vi "CRYO_MASTER_FULL_RUN4.vi"() -> ()   [LabVIEW 2017]
uses:
  LSI218Data.lvclass
  LSI336Data.lvclass
  USBData.lvclass
  6240AData.lvclass
  DMMsData.lvclass
  LMData.lvclass
  <vilib>/DAQmx/miscellaneous.llb/DAQmx Fill In Error Info.vi
  <vilib>/DAQmx/create/channels.llb/DAQmx Create Channel (DO-Digital Output).vi
  <vilib>/DAQmx/create/channels.llb/DAQmx Create Channel (AO-Voltage-Basic).vi
  <vilib>/express/express arith-compare/Formula/XNode/ExpressFormulaBlockNode.xnode
  <vilib>/Analysis/NI_AALBase.lvlib
  istr.lib/Agilent 33XXX Series/Agilent 33XXX Series.lvlib
panel:
  out "Heat Cycle counter":i32
  in  "V_peak":dbl=65.0 format="%_4f"
  in  "Automatic \nScreenshots?":bool=TRUE
  in  "Frontpanel screenshots":bool
  in  "Screenshots interval":i64=3605
  in  "Record interval":i64=20
  out "Cycle #":u32=1
  in  "Measurement Interval (s)":dbl=1.0
  in  "Stop Button":bool
  in  "?":T1(tab)=enum."CHF"
  out "RUN Identifier":string="20210209_084357_RUNIII"
  in  "Base Path (screenshots)":path=path "C:/LabVIEW/DATA/Google/TUCAN Experiments/KEK_cryotests_2019-2020/data/screenshots"
  out "error out (USB6210/6218 AOUT)":errorcluster
  in  "AOUT Labels":string[](array[string])=["PWR400H_I", "PMC183A_I"]
  in  "DOUT Labels":string[](array[string])=["D_V1_NO", "D_V2_NC", "D_CV1", "D_H1"]
  in  "AOUT assignment":tag[](array[tag])=["Dev1/ao0", "Dev1/ao1"]
  out "AO task out":refnum<k21>="20210209_084357_RUNIII_AO"
  in  "Analog Out ON?":bool=TRUE
  in  "InstName (USB6218)":string="USB6218"
  in  "USB6218 Config":T2(array[cluster])=[{"Label"="F_1", "FileFormat"="%5.5f", "Active?"=TRUE, "Physical CH"="Dev1/ai0", " terminal\n type"=10083, "ConversionType"={"Type"=enum."SimpleProp", "ConversionParameters"=[0.0, 5.0, 0.0, 500.0]}, "VoltageLimits"=[0.0, 5.0]}, {"Label"="F_2", "FileFormat"="%5.5f", "Active?"=TRUE, "Physical CH"="Dev1/ai1", " terminal\n type"=10083, "ConversionType"={"Type"=enum."SimpleProp", "ConversionParameters"=[0.0, 5.0, 0.0, 200.0]}, "VoltageLimits"=[0.0, 5.0]}, {"Label"="F_3", "FileFormat"="%5.5f", "Active?"=TRUE, "Physical CH"="Dev1/ai2", " terminal\n type"=10083, "ConversionType"={"Type"=enum."SimpleProp", "ConversionParameters"=[0.0, 5.0, 0.0, 200.0]}, "VoltageLimits"=[0.0, 5.0]}, {"Label"="F_4", "FileFormat"="%5.5f", "Active?"=TRUE, "Physical CH"="Dev1/ai3", " terminal\n type"=10083, "ConversionType"={"Type"=enum."SimpleProp", "ConversionParameters"=[0.0, 5.0, 0.0, 500.0]}, "VoltageLimits"=[0.0, 5.0]}, {"Label"="F_5", "FileFormat"="%5.5f", "Active?"=TRUE, "Physical CH"="Dev1/ai4", " terminal\n type"=10083, "ConversionType"={"Type"=enum."SimpleProp", "ConversionParameters"=[0.0, 5.0, 0.0, 500.0]}, "VoltageLimits"=[0.0, 5.0]}, {"Label"="I_CV", "FileFormat"="%3.5f", "Active?"=TRUE, "Physical CH"="Dev1/ai5", " terminal\n type"=10083, "ConversionType"={"Type"=enum."Raw", "ConversionParameters"=[0.0, 0.0, 0.0, 0.0]}, "VoltageLimits"=[0.0, 10.0]}, {"Label"="CV1_answer", "FileFormat"="%3.5f", "Active?"=TRUE, "Physical CH"="Dev1/ai6", " terminal\n type"=10083, "ConversionType"={"Type"=enum."SimpleProp", "ConversionParameters"=[1.0, 5.0, 0.0, 100.0]}, "VoltageLimits"=[0.0, 5.0]}, {"Label"="P_Dewar", "FileFormat"="%5.5e", "Active?"=TRUE, "Physical CH"="Dev1/ai7", " terminal\n type"=10083, "ConversionType"={"Type"=enum."SimpleProp", "ConversionParameters"=[1.0, 5.0, 0.0, 200000.0]}, "VoltageLimits"=[0.0, 5.0]}, {"Label"="L_Dewar", "FileFormat"="%5.5f", "Active?"=TRUE, "Physical CH"="Dev1/ai8", " terminal\n type"=10083, "ConversionType"={"Type"=enum."SimpleProp", "ConversionParameters"=[0.0, 10.0, 0.0, 100.0]}, "VoltageLimits"=[0.0, 10.0]}] {"terminal\n type" items=["Default"=-1, "RSE"=10083, "NRSE"=10078, "Differential"=10106, "Pseudodifferential"=12529]}
  out "error out (USB6218)":errorcluster
  out "error out (USB6210/6218 DOUT)":errorcluster
  out "DOUT task out":refnum<k21>="20210209_084357_DO"
  in  "DOUT Physical CH":tag[](array[tag])=["Dev1/port1/line0", "Dev1/port1/line1", "Dev1/port1/line2", "Dev1/port1/line3"]
  in  "Digital Out ON?":bool=TRUE
  in  "USB6210 Config":T2(array[cluster])=[{"Label"="P_ins", "FileFormat"="%5.5e", "Active?"=TRUE, "Physical CH"="Dev2/ai0", " terminal\n type"=10083, "ConversionType"={"Type"=enum."CC-10_LOG", "ConversionParameters"=[0.5, 9.0, 0.0, 1.0]}, "VoltageLimits"=[0.0, 10.0]}, {"Label"="P_4Kres", "FileFormat"="%5.5e", "Active?"=TRUE, "Physical CH"="Dev2/ai1", " terminal\n type"=10083, "ConversionType"={"Type"=enum."SimpleProp", "ConversionParameters"=[1.0, 5.0, 0.0, 200000.0]}, "VoltageLimits"=[0.0, 5.0]}, {"Label"="P_3HeIN", "FileFormat"="%5.5e", "Active?"=TRUE, "Physical CH"="Dev2/ai2", " terminal\n type"=10083, "ConversionType"={"Type"=enum."SimpleProp", "ConversionParameters"=[1.0, 5.0, 0.0, 200000.0]}, "VoltageLimits"=[0.0, 5.0]}, {"Label"="P_SldRTN", "FileFormat"="%5.5e", "Active?"=TRUE, "Physical CH"="Dev2/ai3", " terminal\n type"=10083, "ConversionType"={"Type"=enum."SimpleProp", "ConversionParameters"=[1.0, 5.0, 0.0, 200000.0]}, "VoltageLimits"=[0.0, 5.0]}, {"Label"="P_3Hepot", "FileFormat"="%5.5e", "Active?"=TRUE, "Physical CH"="Dev2/ai4", " terminal\n type"=10083, "ConversionType"={"Type"=enum."SimpleProp", "ConversionParameters"=[0.0, 10.0, 0.0, 133320.0]}, "VoltageLimits"=[0.0, 10.0]}, {"Label"="P_1Kpot", "FileFormat"="%5.5e", "Active?"=TRUE, "Physical CH"="Dev2/ai5", " terminal\n type"=10083, "ConversionType"={"Type"=enum."SimpleProp", "ConversionParameters"=[0.0, 10.0, 0.0, 133320.0]}, "VoltageLimits"=[0.0, 10.0]}, {"Label"="P_Dewar(old)", "FileFormat"="%5.5e", "Active?"=FALSE, "Physical CH"="Dev2/ai6", " terminal\n type"=10083, "ConversionType"={"Type"=enum."SimpleProp", "ConversionParameters"=[1.0, 5.0, 0.0, 200000.0]}, "VoltageLimits"=[0.0, 5.0]}, {"Label"="DP_HEX4", "FileFormat"="%5.5e", "Active?"=TRUE, "Physical CH"="Dev2/ai7", " terminal\n type"=10083, "ConversionType"={"Type"=enum."SimpleProp", "ConversionParameters"=[1.0, 5.0, 0.0, 1000.0]}, "VoltageLimits"=[0.0, 5.0]}, {"Label"="DP_HEX5", "FileFormat"="%5.5e", "Active?"=TRUE, "Physical CH"="Dev2/ai8", " terminal\n type"=10083, "ConversionType"={"Type"=enum."SimpleProp", "ConversionParameters"=[1.0, 5.0, 0.0, 1000.0]}, "VoltageLimits"=[0.0, 5.0]}, {"Label"="L1(old)", "FileFormat"="%5.5f", "Active?"=TRUE, "Physical CH"="Dev2/ai9", " terminal\n type"=10083, "ConversionType"={"Type"=enum."SimpleProp", "ConversionParameters"=[0.0, 10.0, 0.0, 100.0]}, "VoltageLimits"=[0.0, 10.0]}, {"Label"="L2-1", "FileFormat"="%5.5f", "Active?"=TRUE, "Physical CH"="Dev2/ai10", " terminal\n type"=10083, "ConversionType"={"Type"=enum."SimpleProp", "ConversionParameters"=[0.0, 10.0, 0.0, 100.0]}, "VoltageLimits"=[0.0, 10.0]}, {"Label"="L2-2", "FileFormat"="%5.5f", "Active?"=TRUE, "Physical CH"="Dev2/ai11", " terminal\n type"=10083, "ConversionType"={"Type"=enum."SimpleProp", "ConversionParameters"=[0.0, 10.0, 0.0, 100.0]}, "VoltageLimits"=[0.0, 10.0]}, {"Label"="L3", "FileFormat"="%5.5f", "Active?"=TRUE, "Physical CH"="Dev2/ai12", " terminal\n type"=10083, "ConversionType"={"Type"=enum."SimpleProp", "ConversionParameters"=[0.0, 10.0, 0.0, 100.0]}, "VoltageLimits"=[0.0, 10.0]}, {"Label"="P_HEX7OUT", "FileFormat"="%5.5e", "Active?"=TRUE, "Physical CH"="Dev2/ai13", " terminal\n type"=10083, "ConversionType"={"Type"=enum."SimpleProp", "ConversionParameters"=[1.0, 5.0, 0.0, 200000.0]}, "VoltageLimits"=[0.0, 5.0]}, {"Label"="P_IP", "FileFormat"="%5.5e", "Active?"=TRUE, "Physical CH"="Dev2/ai14", " terminal\n type"=10083, "ConversionType"={"Type"=enum."CC-10_LOG", "ConversionParameters"=[0.5, 9.0, 0.0, 1.0]}, "VoltageLimits"=[0.0, 10.0]}, {"Label"="V_H1", "FileFormat"="%3.5f", "Active?"=TRUE, "Physical CH"="Dev2/ai15", " terminal\n type"=10083, "ConversionType"={"Type"=enum."Raw", "ConversionParameters"=[0.0, 1.0, 0.0, 1.0]}, "VoltageLimits"=[0.0, 10.0]}] {"terminal\n type" items=["Default"=-1, "RSE"=10083, "NRSE"=10078, "Differential"=10106, "Pseudodifferential"=12529]}
  in  "RUN label":string="RUNIII"
  in  "Base Path":path=path "C:/LabVIEW/DATA/RUN_3"
  in  "InstName (USB6210)":string="USB6210"
  out "error out (USB6210)":errorcluster
  out "File Refn USB AO":refnum<file>
  out "File Refn USB DO":refnum<file>
  in  "LM measurement interval (>0)":i64=1
  in  "Active? (HP34401 LM)":bool=TRUE
  in  "Labels (HP34401 LM)":string[](array[string])=["R_L1", "L1"]
  in  "FileFormat (HP34401 LM)":string[](array[string])=["%.4f", "%.4f"]
  in  "VISA (HP34401 LM)":refnum<visa-resource-name>="GPIB0::24::INSTR"
  in  "LevelCalibration (R0, R1, L0, L1)":dbl[](array[numeric])=[179.74, 0.0, 0.0, 100.0]
  in  "InstName (HP34401 LM)":string="HP34401LM"
  out "error out (LSI336)":errorcluster
  in  "InstName (LSI336)":string="LSI336"
  in  "FileFormat (336)":string="%4.4f"
  in  "LSI336Settings(X,Y)":T3(array[cluster])=[{"LSIName"="LSi336X", "Labels"=["T1K3-1", "T1K3-2", "T3He5", "T3He8"], "SensorLocations"=[enum."T1K3-1", enum."T1K3-2", enum."T3He5", enum."T3He8"], "Active?"=TRUE, "VISA res. name"="COM15_LSI336Y"}, {"LSIName"="LSi336Y", "Labels"=["T3He6-1", "T3He6-2", "T3He7-1", "T3He7-2"], "SensorLocations"=[enum."T3He6-1", enum."T3He6-2", enum."T3He7-1", enum."T3He7-2"], "Active?"=TRUE, "VISA res. name"="COM20_LSI336X"}]
  in  "FileFormat (218)":string="%4.4f"
  in  "InstName (LSI218)":string="LSI218"
  in  "LSI218Settings(A-F)":T3(array[cluster])=[{"LSIName"="LSI218A", "Labels"=["T3He10", "T3He1-1", "TTH3", "TTH4", "TTH1", "TTH2", "T4He1", "T1K1"], "SensorLocations"=[enum."T3He10", enum."T3He1-1", enum."TTH3", enum."TTH4", enum."TTH1", enum."TTH2", enum."T4He1", enum."T1K1"], "Active?"=TRUE, "VISA res. name"="GPIB0::7::INSTR"}, {"LSIName"="LSI218B", "Labels"=["N.C.", "N.C.", "N.C.", "N.C.", "T3He2-1", "T3He2-2", "T3He3", "T3He1-4"], "SensorLocations"=[enum."N.C.", enum."N.C.", enum."N.C.", enum."N.C.", enum."T3He2-1", enum."T3He2-2", enum."T3He3", enum."T3He1-4"], "Active?"=TRUE, "VISA res. name"="GPIB0::4::INSTR"}, {"LSIName"="LSI218C", "Labels"=["T4He3-1", "T4He3-2", "T4He3-3", "T4He3-4", "T4He2-1", "T4He2-2", "T4He4", "T4He5"], "SensorLocations"=[enum."T4He3-1", enum."T4He3-2", enum."T4He3-3", enum."T4He3-4", enum."T4He2-1", enum."T4He2-2", enum."T4He4", enum."T4He5"], "Active?"=TRUE, "VISA res. name"="GPIB0::3::INSTR"}, {"LSIName"="LSI218D", "Labels"=["T4He6", "T4He9", "T3He1-2", "T3He1-3", "T4He7", "T4He8", "T4He10", "T1K6"], "SensorLocations"=[enum."T4He6", enum."T4He9", enum."T3He1-2", enum."T3He1-3", enum."T4He7", enum."T4He8", enum."T4He10", enum."T1K6"], "Active?"=TRUE, "VISA res. name"="GPIB0::5::INSTR"}, {"LSIName"="LSI218E", "Labels"=["TIP1", "N.C.", "TIP2", "N.C.", "TIP3", "TIP4", "TIP5", "N.C."], "SensorLocations"=[enum."TIP1", enum."N.C.", enum."TIP2", enum."N.C.", enum."TIP3", enum."TIP4", enum."TIP5", enum."N.C."], "Active?"=TRUE, "VISA res. name"="GPIB0::11::INSTR"}, {"LSIName"="LSI218F", "Labels"=["T1K2", "T1K4", "T1K5", "T3He4", "T3He9", "TIP6", "N.C.", "N.C."], "SensorLocations"=[enum."T1K2", enum."T1K4", enum."T1K5", enum."T3He4", enum."T3He9", enum."TIP6", enum."N.C.", enum."N.C."], "Active?"=TRUE, "VISA res. name"="GPIB0::8::INSTR"}]
  out "error out (LSI218)":errorcluster={"status"=TRUE, "code"=-1073807338, "source"="VISA Close in Lake Shore Cryotronics 218.lvlib:Close.vi->LSI218Data.lvclass:LSI218Data_terminate.vi->CRYO_MASTER_FULL_RUN3.vi"}
  out "RUN Identifier 2":string="20210209_084357_RUNIII" caption="RUN Identifier"
  out "error out (HP34401 LM)":errorcluster
  out "Graph 3":T4(graph)=[{"TimeArray"=[timestamp(3695672639.4136896 s since 1904-01-01)], "DataArray"=[-0.36185606613019977]}, {"TimeArray"=[timestamp(3695672639.4136896 s since 1904-01-01)], "DataArray"=[-1.4204433335631088]}, {"TimeArray"=[timestamp(3695672639.4136896 s since 1904-01-01)], "DataArray"=[0.28794373208354185]}, {"TimeArray"=[timestamp(3695672639.4136896 s since 1904-01-01)], "DataArray"=[-3.0973798990583647]}, {"TimeArray"=[timestamp(3695672639.4136896 s since 1904-01-01)], "DataArray"=[18.382396544680894]}, {"TimeArray"=[timestamp(3695672639.4136896 s since 1904-01-01)], "DataArray"=[-0.0024966396874153696]}, {"TimeArray"=[timestamp(3695672639.4136896 s since 1904-01-01)], "DataArray"=[107.20664477077275]}] caption="XY Graph"
  out "Graph 1":T4(graph)=[{"TimeArray"=[timestamp(3695672639.4087214 s since 1904-01-01)], "DataArray"=[18.674861858538797]}, {"TimeArray"=[timestamp(3695672639.4087214 s since 1904-01-01)], "DataArray"=[97865.81349287118]}, {"TimeArray"=[timestamp(3695672639.4087214 s since 1904-01-01)], "DataArray"=[100998.44453584745]}, {"TimeArray"=[timestamp(3695672639.4087214 s since 1904-01-01)], "DataArray"=[100709.02551899779]}, {"TimeArray"=[timestamp(3695672639.4087214 s since 1904-01-01)], "DataArray"=[101407.09548804205]}, {"TimeArray"=[timestamp(3695672639.4087214 s since 1904-01-01)], "DataArray"=[101279.08758660906]}, {"TimeArray"=[timestamp(3695672639.4087214 s since 1904-01-01)], "DataArray"=[0.0]}, {"TimeArray"=[timestamp(3695672639.4087214 s since 1904-01-01)], "DataArray"=[100273.25274306418]}, {"TimeArray"=[timestamp(3695672639.4087214 s since 1904-01-01)], "DataArray"=[4.684755546764993e-05]}, {"TimeArray"=[timestamp(3695672639.4136896 s since 1904-01-01)], "DataArray"=[102243.79868545999]}] caption="XY Graph"
  in  "FIle suffix 4":string="Graph4_noise"
  in  "Take Screenshot! 4":bool
  in  "Take Screenshot! 3":bool
  in  "Take Screenshot! 2":bool
  in  "Take Screenshot! 1":bool
  in  "FIle suffix 3":string="Graph3_noise"
  in  "FIle suffix 2":string="Graph2_noise"
  in  "FIle suffix 1":string="Graph1_noise"
  in  "log/linear 2":bool
  in  "Tab Control 2":T5(tab)
  in  "Plot selecter (USB6210)\n    1      2     3     4":bool[][](array[boolean])=[[TRUE, FALSE, FALSE, FALSE], [TRUE, FALSE, FALSE, FALSE], [TRUE, FALSE, FALSE, FALSE], [TRUE, FALSE, FALSE, FALSE], [TRUE, FALSE, FALSE, FALSE], [TRUE, FALSE, FALSE, FALSE], [TRUE, FALSE, FALSE, FALSE], [FALSE, TRUE, FALSE, FALSE], [FALSE, TRUE, FALSE, FALSE], [FALSE, TRUE, FALSE, FALSE], [FALSE, TRUE, FALSE, FALSE], [FALSE, TRUE, FALSE, FALSE], [FALSE, TRUE, FALSE, FALSE], [TRUE, FALSE, FALSE, FALSE], [TRUE, FALSE, FALSE, FALSE], [FALSE, FALSE, FALSE, FALSE]]
  out "All Labels (USB6210)":string[](array[string])=["P_ins", "P_4Kres", "P_3HeIN", "P_SldRTN", "P_3Hepot", "P_1Kpot", "P_Dewar(old)", "DP_HEX4", "DP_HEX5", "L1(old)", "L2-1", "L2-2", "L3", "P_HEX7OUT", "P_IP", "V_H1"]
  out "Last Data \n(USB6210)":dbl[](array[numeric])=[18.674861858538797, 97865.81349287118, 100998.44453584745, 100709.02551899779, 101407.09548804205, 101279.08758660906, 0.0, -48.20456535494683, 0.06691412080322978, 10.108489682314854, 0.1698011167381339, -0.07483544992953703, 0.04024895650740204, 100273.25274306418, 4.684755546764993e-05, 5.953981760223165] format="%#_6e"
  out "Time of Last Measurement (USB6210)":timestamp=timestamp(3695672639.4087214 s since 1904-01-01)
  out "USB6210 Status":T6(ring)=enum."Ready"
  out "Last Vol\n(USB6210)":dbl[](array[numeric])=[8.135628698970727, 2.9573162698574236, 3.019968890716949, 3.0141805103799557, 7.606292790882241, 7.596691238119492, 0.0, 0.8071817385802127, 1.000267656483213, 1.0108489682314854, 0.01698011167381339, -0.007483544992953703, 0.004024895650740204, 3.0054650548612836, 5.335343467039768, 5.953981760223165] format="%_5f"
  out "Labels (HP34401 LM) 2":string[](array[string])=["R_L1", "L1"]
  out "LastData (HP34401 LM)":dbl[](array[numeric])=[166.68232, 7.2647602091910555]
  in  "Plot selecter (HP34401A)\n    1      2     3     4":bool[][](array[boolean])=[[FALSE, TRUE, FALSE, FALSE], [FALSE, TRUE, FALSE, FALSE], [TRUE, FALSE, FALSE, FALSE], [TRUE, FALSE, FALSE, FALSE], [TRUE, FALSE, FALSE, FALSE], [TRUE, FALSE, FALSE, FALSE], [TRUE, FALSE, FALSE, FALSE], [FALSE, TRUE, FALSE, FALSE], [FALSE, TRUE, FALSE, FALSE], [FALSE, TRUE, FALSE, FALSE], [FALSE, TRUE, FALSE, FALSE], [FALSE, TRUE, FALSE, FALSE], [FALSE, TRUE, FALSE, FALSE], [TRUE, FALSE, FALSE, FALSE], [TRUE, FALSE, FALSE, FALSE], [FALSE, FALSE, FALSE, FALSE]]
  out "Time of Last Measurement (USB6218)":timestamp=timestamp(3695672639.4136896 s since 1904-01-01)
  out "USB6218 Status":T6(ring)=enum."Ready"
  out "Last Vol \n(USB6218)":dbl[](array[numeric])=[-0.003618560661301998, -0.03551108333907772, 0.0071985933020885465, -0.030973798990583647, 0.18382396544680896, -0.0024966396874153696, -0.0029609827608362395, 3.0448759737091997, 10.720664477077275] format="%_5f"
  out "Last Data \n(USB6218)":dbl[](array[numeric])=[-0.36185606613019977, -1.4204433335631088, 0.28794373208354185, -3.0973798990583647, 18.382396544680894, -0.0024966396874153696, -25.07402456902091, 102243.79868545999, 107.20664477077275] format="%#_6e"
  out "All Labels (USB6218)":string[](array[string])=["F_1", "F_2", "F_3", "F_4", "F_5", "I_CV", "CV1_answer", "P_Dewar", "L_Dewar"]
  in  "Plot selecter (USB6218)\n    1      2     3     4":bool[][](array[boolean])=[[FALSE, FALSE, TRUE, FALSE], [FALSE, FALSE, TRUE, FALSE], [FALSE, FALSE, TRUE, FALSE], [FALSE, FALSE, TRUE, FALSE], [FALSE, FALSE, TRUE, FALSE], [FALSE, FALSE, TRUE, FALSE], [FALSE, FALSE, FALSE, FALSE], [TRUE, FALSE, FALSE, FALSE], [FALSE, FALSE, TRUE, FALSE], [FALSE, FALSE, FALSE, TRUE], [FALSE, FALSE, FALSE, TRUE], [FALSE, FALSE, FALSE, TRUE], [FALSE, FALSE, FALSE, TRUE], [FALSE, FALSE, FALSE, FALSE], [FALSE, FALSE, FALSE, FALSE], [FALSE, FALSE, FALSE, FALSE]]
  out "Time of Last Measurement (LSI218)":timestamp=timestamp(3695672639.4087214 s since 1904-01-01)
  out "LSI218 Status":T7(ring)=enum."Measuring"
  out "Last Data \nLSI218 (1)":dbl[](array[numeric])=[286.39, 292.79, 245.71, 242.82, 192.73, 208.05, 129.14, 157.86, 30.0, 0.0, 0.0, 0.0, 214.32, 209.26, 161.19, 290.41, 293.53, 293.65, 291.53, 291.58, 216.58, 205.59, 215.41, 218.49]
  out "Labels LSI218 (1)":string[](array[string])=["T3He10", "T3He1-1", "TTH3", "TTH4", "TTH1", "TTH2", "T4He1", "T1K1", "N.C.", "N.C.", "N.C.", "N.C.", "T3He2-1", "T3He2-2", "T3He3", "T3He1-4", "T4He3-1", "T4He3-2", "T4He3-3", "T4He3-4", "T4He2-1", "T4He2-2", "T4He4", "T4He5"]
  in  "Plot selecter LSI218(1)\n    1      2     3     4":bool[][](array[boolean])=[[FALSE, FALSE, FALSE, FALSE], [FALSE, FALSE, FALSE, FALSE], [FALSE, FALSE, FALSE, TRUE], [FALSE, FALSE, FALSE, TRUE], [FALSE, FALSE, FALSE, TRUE], [FALSE, FALSE, FALSE, TRUE], [FALSE, FALSE, FALSE, TRUE], [FALSE, FALSE, FALSE, TRUE], [FALSE, FALSE, FALSE, FALSE], [FALSE, FALSE, FALSE, FALSE], [FALSE, FALSE, FALSE, FALSE], [FALSE, FALSE, FALSE, FALSE], [FALSE, FALSE, FALSE, TRUE], [FALSE, FALSE, FALSE, TRUE], [FALSE, FALSE, FALSE, FALSE], [FALSE, FALSE, FALSE, FALSE], [FALSE, FALSE, FALSE, TRUE], [FALSE, FALSE, FALSE, TRUE], [FALSE, FALSE, FALSE, TRUE], [FALSE, FALSE, FALSE, TRUE], [FALSE, FALSE, FALSE, TRUE], [FALSE, FALSE, FALSE, TRUE], [FALSE, FALSE, FALSE, TRUE], [FALSE, FALSE, FALSE, FALSE]]
  out "Active?\n (1)":bool[](array[boolean])=[TRUE, TRUE, TRUE, TRUE, TRUE, TRUE, TRUE, TRUE, TRUE, TRUE, TRUE, TRUE, TRUE, TRUE, TRUE, TRUE, TRUE, TRUE, TRUE, TRUE, TRUE, TRUE, TRUE, TRUE]
  out "Labels LSI218 (2)":string[](array[string])=["T4He6", "T4He9", "T3He1-2", "T3He1-3", "T4He7", "T4He8", "T4He10", "T1K6", "TIP1", "N.C.", "TIP2", "N.C.", "TIP3", "TIP4", "TIP5", "N.C.", "T1K2", "T1K4", "T1K5", "T3He4", "T3He9", "TIP6", "N.C.", "N.C."]
  out "Active?\n(2)":bool[](array[boolean])=[TRUE, TRUE, TRUE, TRUE, TRUE, TRUE, TRUE, TRUE, TRUE, TRUE, TRUE, TRUE, TRUE, TRUE, TRUE, TRUE, TRUE, TRUE, TRUE, TRUE, TRUE, TRUE, TRUE, TRUE]
  out "Last Data \nLSI218 (2)":dbl[](array[numeric])=[214.17, 227.11, 292.96, 290.69, 256.79, 281.72, 274.72, 287.38, 279.49, 0.0, 232.53, 688.49, 216.83, 149.55, 173.98, 688.58, 178.46, 128.79, 144.74, 152.95, 140.88, 150.1, 0.433, 0.0]
  in  "Plot selecter LSI218(2)\n    1      2     3     4":bool[][](array[boolean])=[[FALSE, FALSE, FALSE, FALSE], [FALSE, FALSE, FALSE, FALSE], [FALSE, FALSE, FALSE, FALSE], [FALSE, FALSE, FALSE, FALSE], [FALSE, FALSE, FALSE, FALSE], [FALSE, FALSE, FALSE, FALSE], [FALSE, FALSE, FALSE, FALSE], [FALSE, FALSE, FALSE, FALSE], [FALSE, FALSE, FALSE, FALSE], [FALSE, FALSE, FALSE, FALSE], [FALSE, FALSE, FALSE, FALSE], [FALSE, FALSE, FALSE, FALSE], [FALSE, FALSE, FALSE, FALSE], [FALSE, FALSE, FALSE, FALSE], [FALSE, FALSE, FALSE, FALSE], [FALSE, FALSE, FALSE, FALSE], [FALSE, FALSE, FALSE, TRUE], [FALSE, FALSE, FALSE, TRUE], [FALSE, FALSE, FALSE, TRUE], [FALSE, FALSE, FALSE, TRUE], [FALSE, FALSE, FALSE, FALSE], [FALSE, FALSE, FALSE, FALSE], [FALSE, FALSE, FALSE, FALSE], [FALSE, FALSE, FALSE, FALSE]]
  in  "Plot selecter LSI336 \n     1      2     3     4":bool[][](array[boolean])=[[FALSE, FALSE, FALSE, TRUE], [FALSE, FALSE, FALSE, TRUE], [FALSE, FALSE, FALSE, TRUE], [FALSE, FALSE, FALSE, TRUE], [FALSE, FALSE, FALSE, TRUE], [FALSE, FALSE, FALSE, TRUE], [FALSE, FALSE, FALSE, TRUE], [FALSE, FALSE, FALSE, TRUE]]
  out "Time of Last Measurement (LSI336)":timestamp=timestamp(3695672639.4087214 s since 1904-01-01)
  out "Last Data \nLSI336":dbl[](array[numeric])=[117.963, 117.927, 169.419, 129.275, 167.919, 163.1, 162.659, 160.848]
  out "Active?\n(LSI336)":bool[](array[boolean])=[TRUE, TRUE, TRUE, TRUE, TRUE, TRUE, TRUE, TRUE]
  out "Labels LSI336":string[](array[string])=["T1K3-1", "T1K3-2", "T3He5", "T3He8", "T3He6-1", "T3He6-2", "T3He7-1", "T3He7-2"]
  out "LSI336 Status":T7(ring)=enum."Measuring"
  in  "log/linear 1":bool
  out "Graph 2":T4(graph)=[{"TimeArray"=[timestamp(3695672639.4087214 s since 1904-01-01)], "DataArray"=[-48.20456535494683]}, {"TimeArray"=[timestamp(3695672639.4087214 s since 1904-01-01)], "DataArray"=[0.06691412080322978]}, {"TimeArray"=[timestamp(3695672639.4087214 s since 1904-01-01)], "DataArray"=[10.108489682314854]}, {"TimeArray"=[timestamp(3695672639.4087214 s since 1904-01-01)], "DataArray"=[0.1698011167381339]}, {"TimeArray"=[timestamp(3695672639.4087214 s since 1904-01-01)], "DataArray"=[-0.07483544992953703]}, {"TimeArray"=[timestamp(3695672639.4087214 s since 1904-01-01)], "DataArray"=[0.04024895650740204]}, {"TimeArray"=[timestamp(3695672639.4087214 s since 1904-01-01)], "DataArray"=[166.68232]}, {"TimeArray"=[timestamp(3695672639.4087214 s since 1904-01-01)], "DataArray"=[7.2647602091910555]}] caption="XY Graph"
  out "Graph 4":T4(graph)=[{"TimeArray"=[timestamp(3695672639.4087214 s since 1904-01-01)], "DataArray"=[245.71]}, {"TimeArray"=[timestamp(3695672639.4087214 s since 1904-01-01)], "DataArray"=[242.82]}, {"TimeArray"=[timestamp(3695672639.4087214 s since 1904-01-01)], "DataArray"=[192.73]}, {"TimeArray"=[timestamp(3695672639.4087214 s since 1904-01-01)], "DataArray"=[208.05]}, {"TimeArray"=[timestamp(3695672639.4087214 s since 1904-01-01)], "DataArray"=[129.14]}, {"TimeArray"=[timestamp(3695672639.4087214 s since 1904-01-01)], "DataArray"=[157.86]}, {"TimeArray"=[timestamp(3695672639.4087214 s since 1904-01-01)], "DataArray"=[214.32]}, {"TimeArray"=[timestamp(3695672639.4087214 s since 1904-01-01)], "DataArray"=[209.26]}, {"TimeArray"=[timestamp(3695672639.4087214 s since 1904-01-01)], "DataArray"=[293.53]}, {"TimeArray"=[timestamp(3695672639.4087214 s since 1904-01-01)], "DataArray"=[293.65]}, {"TimeArray"=[timestamp(3695672639.4087214 s since 1904-01-01)], "DataArray"=[291.53]}, {"TimeArray"=[timestamp(3695672639.4087214 s since 1904-01-01)], "DataArray"=[291.58]}, {"TimeArray"=[timestamp(3695672639.4087214 s since 1904-01-01)], "DataArray"=[216.58]}, {"TimeArray"=[timestamp(3695672639.4087214 s since 1904-01-01)], "DataArray"=[205.59]}, {"TimeArray"=[timestamp(3695672639.4087214 s since 1904-01-01)], "DataArray"=[215.41]}, {"TimeArray"=[timestamp(3695672639.4087214 s since 1904-01-01)], "DataArray"=[178.46]}, {"TimeArray"=[timestamp(3695672639.4087214 s since 1904-01-01)], "DataArray"=[128.79]}, {"TimeArray"=[timestamp(3695672639.4087214 s since 1904-01-01)], "DataArray"=[144.74]}, {"TimeArray"=[timestamp(3695672639.4087214 s since 1904-01-01)], "DataArray"=[152.95]}, {"TimeArray"=[timestamp(3695672639.4087214 s since 1904-01-01)], "DataArray"=[117.963]}, {"TimeArray"=[timestamp(3695672639.4087214 s since 1904-01-01)], "DataArray"=[117.927]}, {"TimeArray"=[timestamp(3695672639.4087214 s since 1904-01-01)], "DataArray"=[169.419]}, {"TimeArray"=[timestamp(3695672639.4087214 s since 1904-01-01)], "DataArray"=[129.275]}, {"TimeArray"=[timestamp(3695672639.4087214 s since 1904-01-01)], "DataArray"=[167.919]}, {"TimeArray"=[timestamp(3695672639.4087214 s since 1904-01-01)], "DataArray"=[163.1]}, {"TimeArray"=[timestamp(3695672639.4087214 s since 1904-01-01)], "DataArray"=[162.659]}, {"TimeArray"=[timestamp(3695672639.4087214 s since 1904-01-01)], "DataArray"=[160.848]}] caption="XY Graph"
  in  "log/linear 4":bool
  in  "log/linear 3":bool
  out "RUN Identifier 3":string="20210209_084357_RUNIII" caption="RUN Identifier"
  in  "AutoFill Source (P)":T8(ring)=enum."USB6218AI"
  in  "AutoFill Source (L)":T8(ring)
  out "RUN Identifier 4":string="20210209_084357_RUNIII" caption="RUN Identifier"
  out "Fill (false)":bool=TRUE
  in  "Fill state":bool
  out "state 1 (false)":bool=TRUE
  out "state 1":bool
  out "state 2":bool
  out "state 2 (false)":bool=TRUE
  out "Status V2 CTRL":enum16{"Pressurize", "Release"}(ring)=enum."Release"
  out "Status V1 CTRL":enum16{"Pressurize", "Release"}(ring)
  out "Lav (%)":dbl=43.184746563343246 format="%0.2f"
  out "Lstd":dbl=0.005294410757043201 format="%0.2f"
  out "Last N M.A. Levels":dbl[](array[numeric])=[43.182022097916416, 43.178240727788925, 43.177254283449095, 43.18267972752829, 43.18366617192395, 43.184323801491566, 43.18859839376898, 43.188105171572296, 43.18498143104121, 43.18300854229432, 43.18415939405067, 43.181528875721675, 43.189256023335034, 43.19862724492309] format="%_5e"
  out "Lstd history":dbl(graph)=0.00311953003864109
  out "Lav history":dbl(graph)=43.183302126935246
  out "Target Index (L)":i32=12
  in  "Auto Fll He L. label":string="L3"
  out "Target Index (P)":i32=7
  in  "Auto Fll Dewar P. label":string="P_Dewar"
  out "He Level":T9(graph)=[{"TimeArray"=[timestamp(3695183960.9608912 s since 1904-01-01), timestamp(3695183961.957368 s since 1904-01-01), timestamp(3695183962.9580655 s since 1904-01-01), timestamp(3695183963.961592 s since 1904-01-01), timestamp(3695183964.958559 s since 1904-01-01), timestamp(3695183965.95824 s since 1904-01-01), timestamp(3695183966.9615526 s since 1904-01-01), timestamp(3695183967.9570584 s since 1904-01-01), timestamp(3695183969.170517 s since 1904-01-01), timestamp(3695183970.170328 s since 1904-01-01), timestamp(3695183971.2289977 s since 1904-01-01), timestamp(3695183972.234284 s since 1904-01-01), timestamp(3695183973.2368255 s since 1904-01-01), timestamp(3695183974.2384686 s since 1904-01-01)], "Filtered X"=[43.18185769046936, 43.17462376512705, 43.179227172287, 43.19501028222973, 43.18580346805203, 43.1772542833975, 43.19632554139665, 43.19303739344301, 43.17330850592768, 43.16936272840992, 43.20092894842209, 43.18251532012701, 43.204217096381115, 43.20684761476211]}, {"TimeArray"=[timestamp(3695183960.9608912 s since 1904-01-01), timestamp(3695183961.957368 s since 1904-01-01), timestamp(3695183962.9580655 s since 1904-01-01), timestamp(3695183963.961592 s since 1904-01-01), timestamp(3695183964.958559 s since 1904-01-01), timestamp(3695183965.95824 s since 1904-01-01), timestamp(3695183966.9615526 s since 1904-01-01), timestamp(3695183967.9570584 s since 1904-01-01), timestamp(3695183969.170517 s since 1904-01-01), timestamp(3695183970.170328 s since 1904-01-01), timestamp(3695183971.2289977 s since 1904-01-01), timestamp(3695183972.234284 s since 1904-01-01), timestamp(3695183973.2368255 s since 1904-01-01), timestamp(3695183974.2384686 s since 1904-01-01)], "Filtered X"=[43.182022097916416, 43.178240727788925, 43.177254283449095, 43.18267972752829, 43.18366617192395, 43.184323801491566, 43.18859839376898, 43.188105171572296, 43.18498143104121, 43.18300854229432, 43.18415939405067, 43.181528875721675, 43.189256023335034, 43.19862724492309]}] caption="XY Graph"
  in  "P_safelimit_high (Pa)":dbl=300000.0 format="%_4e"
  in  "P_safelimit_low (Pa)":dbl=100.0 format="%_4e"
  in  "Auto Fill ON?":bool
  out "Pstd history":dbl(graph)=65.22033190545778
  out "Pav history":dbl(graph)=109652.45552761255
  in  "Mov. Avg Interval":i64=4
  in  "V2 (N.C.)":bool
  in  "V1 (N.O.)":bool=TRUE
  in  "N for sampling":i64=7
  in  "L_low (%)":dbl=100.0 format="%_3f"
  in  "L_high (%)":dbl=100.0 format="%_3g"
  in  "P_2_low (Pa)":dbl=105000.0 format="%_4e"
  in  "P_1_low (Pa)":dbl=120000.0 format="%_4g"
  in  "P_2_high (Pa)":dbl=110000.0 format="%_4e"
  in  "P_1_high (Pa)":dbl=123000.0 format="%_4e"
  out "Dewar Pressure":T9(graph)=[{"TimeArray"=[timestamp(3695183960.9608912 s since 1904-01-01), timestamp(3695183961.957368 s since 1904-01-01), timestamp(3695183962.9580655 s since 1904-01-01), timestamp(3695183963.961592 s since 1904-01-01), timestamp(3695183964.958559 s since 1904-01-01), timestamp(3695183965.95824 s since 1904-01-01), timestamp(3695183966.9615526 s since 1904-01-01), timestamp(3695183967.9570584 s since 1904-01-01), timestamp(3695183969.170517 s since 1904-01-01), timestamp(3695183970.170328 s since 1904-01-01), timestamp(3695183971.2289977 s since 1904-01-01), timestamp(3695183972.234284 s since 1904-01-01), timestamp(3695183973.2368255 s since 1904-01-01), timestamp(3695183974.2384686 s since 1904-01-01)], "Filtered X"=[109963.7475690302, 109450.83786052199, 109450.8378612322, 109845.38379062472, 109769.7624867718, 109506.73186680171, 109649.75476646093, 109764.8306628372, 109529.74704682652, 109345.62561207346, 109794.42160760953, 109480.4288056041, 109766.4746046815, 109687.56541811737]}, {"TimeArray"=[timestamp(3695183960.9608912 s since 1904-01-01), timestamp(3695183961.957368 s since 1904-01-01), timestamp(3695183962.9580655 s since 1904-01-01), timestamp(3695183963.961592 s since 1904-01-01), timestamp(3695183964.958559 s since 1904-01-01), timestamp(3695183965.95824 s since 1904-01-01), timestamp(3695183966.9615526 s since 1904-01-01), timestamp(3695183967.9570584 s since 1904-01-01), timestamp(3695183969.170517 s since 1904-01-01), timestamp(3695183970.170328 s since 1904-01-01), timestamp(3695183971.2289977 s since 1904-01-01), timestamp(3695183972.234284 s since 1904-01-01), timestamp(3695183973.2368255 s since 1904-01-01), timestamp(3695183974.2384686 s since 1904-01-01)], "Filtered X"=[109738.52760097096, 109708.93665645414, 109668.24910755549, 109677.70177035227, 109629.20549978768, 109643.17900135761, 109692.90822766478, 109672.76994571791, 109612.7660857316, 109572.48952204952, 109608.65623233668, 109537.55576802841, 109596.73765749215, 109682.22260900313]}] caption="XY Graph"
  out "Last N M.A. Pressures":dbl[](array[numeric])=[109738.52760097096, 109708.93665645414, 109668.24910755549, 109677.70177035227, 109629.20549978768, 109643.17900135761, 109692.90822766478, 109672.76994571791, 109612.7660857316, 109572.48952204952, 109608.65623233668, 109537.55576802841, 109596.73765749215, 109682.22260900313] format="%_5e"
  out "Pav (Pa)":dbl=109645.85040603587 format="%0.4e"
  out "Pstd":dbl=55.905802738156126 format="%0.4e"
  out "File Refn DewarCTRL":refnum<file>
  out "Error Out (Dewar CTRL":errorcluster
  in  "lower limit (mA) \n(PMC)":dbl=4.0 format="%_3f"
  in  "upper limit (mA)\n (PMC)":dbl=40.0 format="%_3f"
  in  "OUTPUT\n(PMC)":bool
  in  "Set Current (mA)\n (PMC)":dbl=4.0 min=4.0 max=40.0 format="%_3g"
  in  "update values":bool
  out "Monitor Current (mA)":dbl=-0.1982033970495195 min=0.0 max=1.9 format="%_4e"
  in  "update current":bool
  out "USB 6218 AOUT":dbl[](array[numeric])=[0.004, 0.004, 0.06969546425555169, 0.06969546425555169]
  out "Graph 7":T10(graph) caption="XY Graph"
  in  "lower limit (mA) \n(PWR)":dbl=4.0 format="%_3f"
  in  "upper limit (mA)\n (PWR)":dbl=20.0 format="%_3f"
  in  "lower limit (mA)":dbl=4.0 format="%_3f"
  in  "SetCurrent 2 (mA)":dbl=4.0 min=4.0 max=500.0 format="%_3f"
  in  "upper limit (mA)":dbl=500.0 format="%_3f"
  out "error out (KIKUSI CTRL)":errorcluster
  out "ActualVoltage (V)":dbl[](array[numeric]) format="%_6g"
  out "ActualCurrent (A)":dbl[](array[numeric])=[0.004, 0.004] format="%_3e"
  in  "SetCurrent 1 (mA)":dbl=4.0 min=4.0 max=500.0 format="%_3g"
  in  "Output\n (ADCMT)":bool[](array[boolean])=[FALSE, FALSE]
  out "error out (ADCMT6420A)":errorcluster
  in  "Voltage limits (V)":dbl[](array[numeric])=[12.0, 12.0] format="%_3f"
  in  "CtrlLabels":string[](array[string])=["CV2", "CV3"]
  in  "VISA":refnum<visa-resource-name>[](array[refnum])=["GPIB0::1::INSTR", "GPIB0::12::INSTR"]
  out "Initialized?":bool
  in  "InstName":string="ADCMT6240"
  out "Graph 6":T9(graph)=[{"TimeArray"=[timestamp(3695085214.3168983 s since 1904-01-01), timestamp(3695085244.964852 s since 1904-01-01), timestamp(3695085246.0168433 s since 1904-01-01), timestamp(3695085588.0010176 s since 1904-01-01)], "Filtered X"=[0.001, 0.005, 0.005, 0.01]}, {"TimeArray"=[timestamp(3695085214.3168983 s since 1904-01-01), timestamp(3695085244.964852 s since 1904-01-01), timestamp(3695085246.0168433 s since 1904-01-01), timestamp(3695085588.0010176 s since 1904-01-01)], "Filtered X"=[0.004, 0.004, 0.004, 0.004]}, {"TimeArray"=[timestamp(3695085214.3168983 s since 1904-01-01), timestamp(3695085244.964852 s since 1904-01-01), timestamp(3695085246.0168433 s since 1904-01-01), timestamp(3695085588.0010176 s since 1904-01-01)], "Filtered X"=[0.001, 0.005, 0.005, 0.01]}, {"TimeArray"=[timestamp(3695085214.3168983 s since 1904-01-01), timestamp(3695085244.964852 s since 1904-01-01), timestamp(3695085246.0168433 s since 1904-01-01), timestamp(3695085588.0010176 s since 1904-01-01)], "Filtered X"=[0.004, 0.004, 0.004, 0.004]}] caption="XY Graph"
  in  "Initialize":bool
  in  "CONTROL KIKUSUI?":bool=TRUE
  in  "OUTPUT\n(PWR)":bool
  in  "Set Current (mA)\n (PWR)":dbl=4.0 min=4.0 max=20.0 format="%_3g"
  out "RUN Identifier 5":string="20210209_084357_RUNIII" caption="RUN Identifier"
  in  "DMMsConfig":T11(array[cluster])=[{"Label"="I_H1", "Active?"=TRUE, "VISA resource name"="USB0::0x1334::0x0204::262800066::INSTR", "Device"=enum."ADCMT7351", "Measurement"=enum."DC Currents", "FileFormat"="%.4e"}, {"Label"="V_H1", "Active?"=TRUE, "VISA resource name"="USB0::0x1334::0x0204::262800451::INSTR", "Device"=enum."ADCMT7351", "Measurement"=enum."DC Volts", "FileFormat"="%.4e"}, {"Label"="I_H2", "Active?"=TRUE, "VISA resource name"="GPIB0::23::INSTR", "Device"=enum."ADCMT7451", "Measurement"=enum."DC Currents", "FileFormat"="%.4e"}, {"Label"="V_H2", "Active?"=TRUE, "VISA resource name"="GPIB0::22::INSTR", "Device"=enum."Agilent34401A", "Measurement"=enum."DC Volts", "FileFormat"="%.4e"}, {"Label"="I_H4", "Active?"=TRUE, "VISA resource name"="GPIB0::21::INSTR", "Device"=enum."Agilent34401A", "Measurement"=enum."DC Currents", "FileFormat"="%.4e"}, {"Label"="V_H4", "Active?"=TRUE, "VISA resource name"="GPIB0::25::INSTR", "Device"=enum."Agilent34401A", "Measurement"=enum."DC Volts", "FileFormat"="%.4e"}]
  out "ƒ¢T=T_2 -T_1":dbl=-101388.71309149737
  out "Graph DMMs 3":T4(graph)=[{"TimeArray"=[timestamp(3695672642.6155486 s since 1904-01-01)], "DataArray"=[-2.68e-05]}, {"TimeArray"=[timestamp(3695672642.6155486 s since 1904-01-01)], "DataArray"=[-0.0014684]}, {"TimeArray"=[timestamp(3695672642.6155486 s since 1904-01-01)], "DataArray"=[-1.232e-05]}, {"TimeArray"=[timestamp(3695672642.6155486 s since 1904-01-01)], "DataArray"=[2.8262e-06]}, {"TimeArray"=[timestamp(3695672642.6155486 s since 1904-01-01)], "DataArray"=[3.71392e-06]}, {"TimeArray"=[timestamp(3695672642.6155486 s since 1904-01-01)], "DataArray"=[0.000182]}, {"TimeArray"=[timestamp(3695672642.6155486 s since 1904-01-01)], "DataArray"=[101407.09548804205]}, {"TimeArray"=[timestamp(3695672642.6155486 s since 1904-01-01)], "DataArray"=[-0.36185606613019977]}, {"TimeArray"=[timestamp(3695672642.6155486 s since 1904-01-01)], "DataArray"=[-3.0973798990583647]}, {"TimeArray"=[timestamp(3695672642.6155486 s since 1904-01-01)], "DataArray"=[18.382396544680894]}, {"TimeArray"=[timestamp(3695672642.6155486 s since 1904-01-01)], "DataArray"=[-48.20456535494683]}, {"TimeArray"=[timestamp(3695672642.6155486 s since 1904-01-01)], "DataArray"=[167.919]}, {"TimeArray"=[timestamp(3695672642.6155486 s since 1904-01-01)], "DataArray"=[163.1]}, {"TimeArray"=[timestamp(3695672642.6155486 s since 1904-01-01)], "DataArray"=[162.659]}, {"TimeArray"=[timestamp(3695672642.6155486 s since 1904-01-01)], "DataArray"=[160.848]}] caption="XY Graph"
  out "Q = I *V":dbl=3.935312e-08
  in  "index I":i64
  in  "index V":i64=1
  out "VariableSources":T12(array[ring])=[enum."USB6210", enum."USB6218AI", enum."USB6218AI", enum."USB6218AI", enum."USB6210", enum."LSI336", enum."LSI336", enum."LSI336", enum."LSI336"]
  in  "DMMsConfig (variables)":T13(array[cluster])=[{"Label"="P_3Hepot", "Active?"=TRUE, "Source"=enum."USB6210", "SourceLabel"="P_3Hepot", "FileFormat"="%6.4e"}, {"Label"="F_1", "Active?"=TRUE, "Source"=enum."USB6218AI", "SourceLabel"="F_1", "FileFormat"="%3.4f"}, {"Label"="F_4", "Active?"=TRUE, "Source"=enum."USB6218AI", "SourceLabel"="F_4", "FileFormat"="%3.4f"}, {"Label"="F_5", "Active?"=TRUE, "Source"=enum."USB6218AI", "SourceLabel"="F_5", "FileFormat"="%3.4f"}, {"Label"="DP_HEX4", "Active?"=TRUE, "Source"=enum."USB6210", "SourceLabel"="DP_HEX4", "FileFormat"="%4.3e"}, {"Label"="T3He6-1", "Active?"=TRUE, "Source"=enum."LSI336", "SourceLabel"="T3He6-1", "FileFormat"="%3.4f"}, {"Label"="T3He6-2", "Active?"=TRUE, "Source"=enum."LSI336", "SourceLabel"="T3He6-2", "FileFormat"="%3.4f"}, {"Label"="T3He7-1", "Active?"=TRUE, "Source"=enum."LSI336", "SourceLabel"="T3He7-1", "FileFormat"="%3.4f"}, {"Label"="T3He7-2", "Active?"=TRUE, "Source"=enum."LSI336", "SourceLabel"="T3He7-2", "FileFormat"="%3.4f"}]
  in  "Measure DMMs?":bool=TRUE
  out "DMMsLabels":string[](array[string])=["I_H1", "V_H1", "I_H2", "V_H2", "I_H4", "V_H4", "P_3Hepot", "F_1", "F_4", "F_5", "DP_HEX4", "T3He6-1", "T3He6-2", "T3He7-1", "T3He7-2"]
  out "Active?":bool[](array[boolean])=[TRUE, TRUE, TRUE, TRUE, TRUE, TRUE, TRUE, TRUE, TRUE, TRUE, TRUE, TRUE, TRUE, TRUE, TRUE]
  out "DMM LastMeasurements":dbl[](array[numeric])=[-2.68e-05, -0.0014684, -1.232e-05, 2.8262e-06, 3.71392e-06, 0.000182, 101407.09548804205, -0.36185606613019977, -3.0973798990583647, 18.382396544680894, -48.20456535494683, 167.919, 163.1, 162.659, 160.848]
  out "Graph DMMs 2":T4(graph)=[{"TimeArray"=[timestamp(3695672642.6155486 s since 1904-01-01)], "DataArray"=[-2.68e-05]}, {"TimeArray"=[timestamp(3695672642.6155486 s since 1904-01-01)], "DataArray"=[-0.0014684]}, {"TimeArray"=[timestamp(3695672642.6155486 s since 1904-01-01)], "DataArray"=[-1.232e-05]}, {"TimeArray"=[timestamp(3695672642.6155486 s since 1904-01-01)], "DataArray"=[2.8262e-06]}, {"TimeArray"=[timestamp(3695672642.6155486 s since 1904-01-01)], "DataArray"=[3.71392e-06]}, {"TimeArray"=[timestamp(3695672642.6155486 s since 1904-01-01)], "DataArray"=[0.000182]}, {"TimeArray"=[timestamp(3695672642.6155486 s since 1904-01-01)], "DataArray"=[101407.09548804205]}, {"TimeArray"=[timestamp(3695672642.6155486 s since 1904-01-01)], "DataArray"=[-0.36185606613019977]}, {"TimeArray"=[timestamp(3695672642.6155486 s since 1904-01-01)], "DataArray"=[-3.0973798990583647]}, {"TimeArray"=[timestamp(3695672642.6155486 s since 1904-01-01)], "DataArray"=[18.382396544680894]}, {"TimeArray"=[timestamp(3695672642.6155486 s since 1904-01-01)], "DataArray"=[-48.20456535494683]}, {"TimeArray"=[timestamp(3695672642.6155486 s since 1904-01-01)], "DataArray"=[167.919]}, {"TimeArray"=[timestamp(3695672642.6155486 s since 1904-01-01)], "DataArray"=[163.1]}, {"TimeArray"=[timestamp(3695672642.6155486 s since 1904-01-01)], "DataArray"=[162.659]}, {"TimeArray"=[timestamp(3695672642.6155486 s since 1904-01-01)], "DataArray"=[160.848]}] caption="XY Graph"
  out "DMMFileName":string="20210209_084357_RUNIII_DMMs_20210209_084357.csv"
  out "error out (DMMs)":errorcluster
  out "cycle # (DMMs)":i32=1
  in  "Measurement Interval DMMs (ms)":i64=500
  in  "InstName DMMs":string="DMMs"
  in  "Initialize (DMMs)":bool
  out "Graph DMMs 1":T4(graph)=[{"TimeArray"=[timestamp(3695672642.6155486 s since 1904-01-01)], "DataArray"=[-2.68e-05]}, {"TimeArray"=[timestamp(3695672642.6155486 s since 1904-01-01)], "DataArray"=[-0.0014684]}, {"TimeArray"=[timestamp(3695672642.6155486 s since 1904-01-01)], "DataArray"=[-1.232e-05]}, {"TimeArray"=[timestamp(3695672642.6155486 s since 1904-01-01)], "DataArray"=[2.8262e-06]}, {"TimeArray"=[timestamp(3695672642.6155486 s since 1904-01-01)], "DataArray"=[3.71392e-06]}, {"TimeArray"=[timestamp(3695672642.6155486 s since 1904-01-01)], "DataArray"=[0.000182]}, {"TimeArray"=[timestamp(3695672642.6155486 s since 1904-01-01)], "DataArray"=[101407.09548804205]}, {"TimeArray"=[timestamp(3695672642.6155486 s since 1904-01-01)], "DataArray"=[-0.36185606613019977]}, {"TimeArray"=[timestamp(3695672642.6155486 s since 1904-01-01)], "DataArray"=[-3.0973798990583647]}, {"TimeArray"=[timestamp(3695672642.6155486 s since 1904-01-01)], "DataArray"=[18.382396544680894]}, {"TimeArray"=[timestamp(3695672642.6155486 s since 1904-01-01)], "DataArray"=[-48.20456535494683]}, {"TimeArray"=[timestamp(3695672642.6155486 s since 1904-01-01)], "DataArray"=[167.919]}, {"TimeArray"=[timestamp(3695672642.6155486 s since 1904-01-01)], "DataArray"=[163.1]}, {"TimeArray"=[timestamp(3695672642.6155486 s since 1904-01-01)], "DataArray"=[162.659]}, {"TimeArray"=[timestamp(3695672642.6155486 s since 1904-01-01)], "DataArray"=[160.848]}] caption="XY Graph"
  out "error out (DMM graphs)":errorcluster
  in  "Sample #":i32=5
  in  "index T_ 1":i64=6
  in  "index T_2":i64=9
  out "error out (DMMs) 2":errorcluster
  out "P_HEX7OUT":dbl=101021.4665932051 format="%_4e"
  out "P (HEX7 out)":dbl=101021.4665932051 format="%_4e"
  out "DP HEX5":dbl=-4.397643774686294 format="%_4e"
  out "DP_HEX5":dbl=-4.397643774686294 format="%_4e"
  in  "Diff pressure HEX5":string="DP_HEX5"
  out "3He pot level":dbl=7.365405585846229 format="%_4f"
  in  "3He pot":string="L1"
  out "He level (3He)":dbl(slide)=7.365405585846229 scale=0.0..100.0
  out "He level (1K) b":dbl(slide)=-0.047872817403439266 scale=0.0..100.0
  out "He level (1K)":dbl(slide)=0.13428935722636412 scale=0.0..100.0
  out "He level (4K)":dbl(slide)=-0.023540685641880416 scale=0.0..100.0
  out "1K pot(b1)":dbl=-0.047872817403439266 format="%_4f"
  in  "1K pot (b)":string="L2-2"
  in  "1K pot level":string="L2-1"
  out "L(1K) (a1)":dbl=0.13428935722636412 format="%_4f"
  in  "SensorLocation 2":T14(ring)=enum."T3He5"
  out "Temperature 2":dbl=167.912
  out "DP HEX4":dbl=-47.57146989712546 format="%_4e"
  in  "Diff pressure HEX4":string="DP_HEX4"
  out "V2":bool
  out "V1":bool=TRUE
  out "F5 (1K pump ex.)":dbl=17.202044578830606 format="%_4f"
  out "F4 (3He in to HEX7)":dbl=-7.769469766427424 format="%_3f"
  out "F3 (4He rtn flw via HEX7)":dbl=2.98269711881182 format="%_4f"
  out "F1 (3He pump exhaust) flow":dbl=-5.195052785009831 format="%_4f"
  out "P (Dewar)":dbl=102950.69349153554 format="%_4e"
  out "P (1K pot)":dbl=101443.04292994068 format="%_4e"
  out "P (3He pot)":dbl=101551.76197190638 format="%_4e"
  out "P (shield return)":dbl=101480.26148830613 format="%_4e"
  out "P (3He IN)":dbl=100240.36414180837 format="%_4e"
  out "P (4K reservoir)":dbl=97813.1918911886 format="%_4e"
  out "P (insulation)":dbl=18.32747458588863 format="%_4e"
  in  "1Kpot pump exhaust flow":string="F_5"
  out "F_5":dbl=17.202044578830606 format="%_4f"
  in  "3He incoming flow into HEX7":string="F_4"
  out "F_4":dbl=-7.769469766427424 format="%_4f"
  out "F_3":dbl=2.98269711881182 format="%_4f"
  in  "4He return flow from HEX7":string="F_3"
  out "F_2":dbl=0.20377377393752083 format="%_4f"
  in  "Shield flow":string="F_2"
  out "P_SldRTN":dbl=101480.26148830613 format="%_4e"
  in  "3He pot pressure":string="P_3Hepot"
  out "P_3Hepot":dbl=101551.76197190638 format="%_4e"
  in  "Shield return press.":string="P_SldRTN"
  out "F_1":dbl=-5.195052785009831 format="%_4f"
  in  "3He pump exhaust flow":string="F_1"
  out "P_Dewar":dbl=102950.69349153554 format="%_4e"
  in  "Dewar pressure":string="P_Dewar"
  out "P_1Kpot":dbl=101443.04292994068 format="%_4e"
  in  "1Kpot pressure":string="P_1Kpot"
  out "P_3HeIN":dbl=100240.36414180837 format="%_4e"
  in  "3He inlet pressure":string="P_3HeIN"
  in  "4K reservoir pressure":string="P_4Kres"
  out "P_4Kres":dbl=97813.1918911886 format="%_4e"
  out "P_ins":dbl=18.32747458588863 format="%_4e"
  in  "Insulation vacuum":string="P_ins"
  out "T3He7-1/6-2 (3He pot) 2":dbl=159.065 format="%_4f"
  out "T3He7-1/7-2 (HEX1)":dbl=160.911 format="%_4f"
  out "T3He6-1/6-2 (3He pot) 2":dbl=161.329 format="%_4f"
  out "T3He6-1/6-2 (HEX1)":dbl=166.258 format="%_4f"
  out "T1K3-1/3-2 (1K pot) 2":dbl=116.203 format="%_4f"
  out "T1K3-1/3-2 (1K pot)":dbl=116.239 format="%_4f"
  out "T4He1 (4K reservoir )":dbl=127.38 format="%_4f"
  out "Temperature 1":dbl=206.95
  in  "SensorLocation 1":T14(ring)=enum."TTH2"
  out "TIP7":dbl format="%_4g"
  out "T3He6-2":dbl=161.329 format="%_4g"
  out "T3He7-2":dbl=159.065 format="%_4g"
  out "T3He6-1":dbl=166.258 format="%_4g"
  out "T3He4":dbl=154.09 format="%_4g"
  out "T3He7-1":dbl=160.911 format="%_4g"
  out "T3He8":dbl=127.318 format="%_4g"
  out "T3He5":dbl=167.912 format="%_4g"
  out "T1K3-2":dbl=116.203 format="%_4g"
  out "T1K3-1":dbl=116.239 format="%_4g"
  out "TIP6":dbl=147.89 format="%_4g"
  out "T3He9":dbl=137.88 format="%_4g"
  out "T1K5":dbl=143.12 format="%_4g"
  out "T1K4":dbl=127.59 format="%_4g"
  out "T1K2":dbl=178.09 format="%_4g"
  out "TIP5":dbl=172.64 format="%_4g"
  out "TIP4":dbl=147.93 format="%_4g"
  out "TIP3":dbl=215.82 format="%_4g"
  out "TIP2":dbl=231.74 format="%_4g"
  out "TIP1":dbl=279.25 format="%_4g"
  out "T1K6":dbl=286.82 format="%_4g"
  out "T4He10":dbl=274.41 format="%_4g"
  out "T4He8":dbl=281.47 format="%_4g"
  out "T4He7":dbl=256.33 format="%_4g"
  out "T3He1-3":dbl=289.96 format="%_4g"
  out "T3He1-2":dbl=292.25 format="%_4g"
  out "T4He9":dbl=226.25 format="%_4g"
  out "T4He6":dbl=213.01 format="%_4g"
  out "T4He5":dbl=217.43 format="%_4g"
  out "T4He4":dbl=214.31 format="%_4g"
  out "T4He2-2":dbl=204.35 format="%_4g"
  out "T4He2-1":dbl=215.52 format="%_4g"
  out "T4He3-4":dbl=290.83 format="%_4g"
  out "T4He3-3":dbl=290.77 format="%_4g"
  out "T4He3-2":dbl=292.95 format="%_4g"
  out "T4He3-1":dbl=292.82 format="%_4g"
  out "T3He1-4":dbl=289.7 format="%_4g"
  out "T3He3":dbl=159.56 format="%_4g"
  out "T3He2-2":dbl=208.05 format="%_4g"
  out "T3He2-1":dbl=213.16 format="%_4g"
  out "T1K1":dbl=156.15 format="%_4g"
  out "T4He1":dbl=127.38 format="%_4g"
  out "TTH1":dbl=191.48 format="%_4g"
  out "TTH2":dbl=206.95 format="%_4g"
  out "TTH4":dbl=242.22 format="%_4g"
  out "TTH3":dbl=244.99 format="%_4g"
  out "T3He1-1":dbl=291.98 format="%_4g"
  out "T3He10":dbl=285.72 format="%_4g"
  out "F2 (shield flow)":dbl=0.20377377393752083 format="%_4f"
  out "DP_HEX4":dbl=-47.57146989712546 format="%_4e"
  in  "4K reservoir level":string="L3"
  out "L3":dbl=-0.023540685641880416 format="%_4f"
  out "RUN Identifier 6":string="20210209_084357_RUNIII" caption="RUN Identifier"
  in  "HEX7 out pressure":string="P_HEX7OUT"
  in  "CHF Graph Comment":string="CHF_TEST2"
  in  "REFRESH GRAPH":bool
  in  "RECORD GRAPH":bool
  out "Graph CHF log 2":T4(graph) caption="XY Graph"
  out "ƒ¢T_array":dbl[](array[numeric])=[52.7753, 52.7753, 52.7113, 52.7149, 52.7149, 52.4737, 52.4737, 52.4737, 52.3482, 52.3482, 52.178799999999995, 52.165000000000006, 52.165000000000006, 52.165000000000006, 52.0492, 52.0492, 51.9912, 51.9912, 51.9912, 51.7804, 51.7804, 51.7804, 51.6556, 51.6556, 51.6556, 51.5194, 51.5194, 51.447500000000005, 51.3779, 51.3779, 51.3779, 51.1899, 51.1899, 51.2118, 51.2118, 51.2118, 51.182199999999995, 51.1555, 51.1555, 51.0157, 51.0157, 51.0157, 50.9915, 50.9915, 50.8838, 50.926899999999996, 50.926899999999996, 50.861599999999996, 50.861599999999996, 50.861599999999996, 50.876400000000004, 50.876400000000004, 50.748400000000004, 50.7998, 50.7998, 50.7998, 50.7818, 50.7818, 50.8097, 50.8097, 50.8097, 50.7905, 50.7905, 50.7905, 50.8299, 50.8299, 50.8299, 50.8304, 50.8304, 50.8908, 50.884699999999995, 50.884699999999995, 51.0378, 51.0378, 51.0378, 51.019000000000005, 51.019000000000005, 51.120799999999996, 51.156600000000005, 51.156600000000005, 51.156600000000005, 51.2329, 51.2329, 51.369299999999996, 51.369299999999996, 51.369299999999996, 51.5356, 51.5356, 51.5356, 51.6671, 51.6671, 51.6671, 51.8208, 51.8208, 51.987899999999996, 52.0073, 52.0073, 52.2344, 52.2344, 52.2344, 52.459, 52.459, 52.672399999999996, 52.708999999999996, 52.708999999999996, 52.708999999999996, 52.9287, 52.9287, 53.1942, 53.1942, 53.1942, 53.5324, 53.5324, 53.5324, 53.849000000000004, 53.849000000000004, 53.849000000000004, 54.1092, 54.1092, 54.4229, 54.5156, 54.5156, 54.8154, 54.8154, 54.8154, 55.2085, 55.2085, 55.5868, 55.656800000000004, 55.656800000000004]
  out "Graph CHF":cluster{dbl[], dbl[]}(graph)={[52.7753, 52.7753, 52.7113, 52.7149, 52.7149, 52.4737, 52.4737, 52.4737, 52.3482, 52.3482, 52.178799999999995, 52.165000000000006, 52.165000000000006, 52.165000000000006, 52.0492, 52.0492, 51.9912, 51.9912, 51.9912, 51.7804, 51.7804, 51.7804, 51.6556, 51.6556, 51.6556, 51.5194, 51.5194, 51.447500000000005, 51.3779, 51.3779, 51.3779, 51.1899, 51.1899, 51.2118, 51.2118, 51.2118, 51.182199999999995, 51.1555, 51.1555, 51.0157, 51.0157, 51.0157, 50.9915, 50.9915, 50.8838, 50.926899999999996, 50.926899999999996, 50.861599999999996, 50.861599999999996, 50.861599999999996, 50.876400000000004, 50.876400000000004, 50.748400000000004, 50.7998, 50.7998, 50.7998, 50.7818, 50.7818, 50.8097, 50.8097, 50.8097, 50.7905, 50.7905, 50.7905, 50.8299, 50.8299, 50.8299, 50.8304, 50.8304, 50.8908, 50.884699999999995, 50.884699999999995, 51.0378, 51.0378, 51.0378, 51.019000000000005, 51.019000000000005, 51.120799999999996, 51.156600000000005, 51.156600000000005, 51.156600000000005, 51.2329, 51.2329, 51.369299999999996, 51.369299999999996, 51.369299999999996, 51.5356, 51.5356, 51.5356, 51.6671, 51.6671, 51.6671, 51.8208, 51.8208, 51.987899999999996, 52.0073, 52.0073, 52.2344, 52.2344, 52.2344, 52.459, 52.459, 52.672399999999996, 52.708999999999996, 52.708999999999996, 52.708999999999996, 52.9287, 52.9287, 53.1942, 53.1942, 53.1942, 53.5324, 53.5324, 53.5324, 53.849000000000004, 53.849000000000004, 53.849000000000004, 54.1092, 54.1092, 54.4229, 54.5156, 54.5156, 54.8154, 54.8154, 54.8154, 55.2085, 55.2085, 55.5868, 55.656800000000004, 55.656800000000004], [64.988847618, 0.0008371808639999999, 0.0008371808639999999, 0.0008371808639999999, 0.0008371808639999999, 0.0008371808639999999, 0.0008371808639999999, 0.0008371808639999999, 0.0008371808639999999, 0.0008371808639999999, 0.027133083646800005, 0.027133083646800005, 0.027133083646800005, 0.027133083646800005, 0.027133083646800005, 0.027133083646800005, 0.027133083646800005, 0.027133083646800005, 0.497141592024, 0.497141592024, 0.497141592024, 0.497141592024, 0.497141592024, 0.497141592024, 0.497141592024, 0.497141592024, 1.476215545728, 1.476215545728, 1.476215545728, 1.476215545728, 1.476215545728, 1.476215545728, 1.476215545728, 1.476215545728, 1.476215545728, 3.02773055424, 3.02773055424, 3.02773055424, 3.02773055424, 3.02773055424, 3.02773055424, 3.02773055424, 3.02773055424, 4.86484683444, 4.86484683444, 4.86484683444, 4.86484683444, 4.86484683444, 4.86484683444, 4.86484683444, 4.86484683444, 4.86484683444, 7.4475440352, 7.4475440352, 7.4475440352, 7.4475440352, 7.4475440352, 7.4475440352, 7.4475440352, 7.4475440352, 10.986195312400001, 10.986195312400001, 10.986195312400001, 10.986195312400001, 10.986195312400001, 10.986195312400001, 10.986195312400001, 10.986195312400001, 14.5582761144, 14.5582761144, 14.5582761144, 14.5582761144, 14.5582761144, 14.5582761144, 14.5582761144, 14.5582761144, 14.5582761144, 16.831454674799996, 16.831454674799996, 16.831454674799996, 16.831454674799996, 16.831454674799996, 16.831454674799996, 16.831454674799996, 16.831454674799996, 23.431170976799997, 23.431170976799997, 23.431170976799997, 23.431170976799997, 23.431170976799997, 23.431170976799997, 23.431170976799997, 23.431170976799997, 28.729140804, 28.729140804, 28.729140804, 28.729140804, 28.729140804, 28.729140804, 28.729140804, 28.729140804, 28.729140804, 31.9837009252, 31.9837009252, 31.9837009252, 31.9837009252, 31.9837009252, 31.9837009252, 31.9837009252, 31.9837009252, 40.691919848000005, 40.691919848000005, 40.691919848000005, 40.691919848000005, 40.691919848000005, 40.691919848000005, 40.691919848000005, 40.691919848000005, 47.4670420756, 47.4670420756, 47.4670420756, 47.4670420756, 47.4670420756, 47.4670420756, 47.4670420756, 47.4670420756, 47.4670420756, 50.1891742, 50.1891742, 50.1891742]}
  in  "V_lim_low (V)":dbl format="%_5f"
  in  "V_lim_up (V)":dbl=120.0 format="%_5f"
  out "V":dbl=52.931
  out "I":dbl=0.9481999999999999
  out "Q":dbl=50.1891742
  out "T_low":dbl=4.3544
  out "error out (Agilent)":errorcluster
  in  "VISA (Agilent 34402)":refnum<visa-resource-name>="USB0::0x0957::0x0407::MY44010230::INSTR"
  out "Agilent\nIntialized?":bool
  in  "Initialize (Agilent)":bool=TRUE
  in  "OUTPUT \nKenwood":bool
  in  "Kenwood set V (V)":dbl min=0.0 max=120.0 format="%_5f"
  out "Graph CHF log 1":T4(graph) caption="XY Graph"
  out "CHF Data Labels":string[](array[string])=["I_H1", "V_H1", "P_3Hepot", "F_1", "F_4", "F_5", "DP_HEX4", "T3He6-1", "T3He6-2", "T3He7-1", "T3He7-2", "T1K3-1", "T1K3-2"]
  out "CHF last data":dbl[](array[numeric])=[0.9481999999999999, 52.931, 102652.98108709365, 62.055409553750465, -0.5229626466829013, 2.2553033880524875, -50.30940195270617, 4.3544, 51.4202, 48.6656, 60.0112, 4.2108, 4.2278]
  out "Error out (CHF rec)":errorcluster
  out "CHF measurement counter":i32
  out "T_high":dbl=60.0112
  out "ƒ¢T":dbl=55.656800000000004
  out "Q_array":dbl[](array[numeric])=[64.988847618, 0.0008371808639999999, 0.0008371808639999999, 0.0008371808639999999, 0.0008371808639999999, 0.0008371808639999999, 0.0008371808639999999, 0.0008371808639999999, 0.0008371808639999999, 0.0008371808639999999, 0.027133083646800005, 0.027133083646800005, 0.027133083646800005, 0.027133083646800005, 0.027133083646800005, 0.027133083646800005, 0.027133083646800005, 0.027133083646800005, 0.497141592024, 0.497141592024, 0.497141592024, 0.497141592024, 0.497141592024, 0.497141592024, 0.497141592024, 0.497141592024, 1.476215545728, 1.476215545728, 1.476215545728, 1.476215545728, 1.476215545728, 1.476215545728, 1.476215545728, 1.476215545728, 1.476215545728, 3.02773055424, 3.02773055424, 3.02773055424, 3.02773055424, 3.02773055424, 3.02773055424, 3.02773055424, 3.02773055424, 4.86484683444, 4.86484683444, 4.86484683444, 4.86484683444, 4.86484683444, 4.86484683444, 4.86484683444, 4.86484683444, 4.86484683444, 7.4475440352, 7.4475440352, 7.4475440352, 7.4475440352, 7.4475440352, 7.4475440352, 7.4475440352, 7.4475440352, 10.986195312400001, 10.986195312400001, 10.986195312400001, 10.986195312400001, 10.986195312400001, 10.986195312400001, 10.986195312400001, 10.986195312400001, 14.5582761144, 14.5582761144, 14.5582761144, 14.5582761144, 14.5582761144, 14.5582761144, 14.5582761144, 14.5582761144, 14.5582761144, 16.831454674799996, 16.831454674799996, 16.831454674799996, 16.831454674799996, 16.831454674799996, 16.831454674799996, 16.831454674799996, 16.831454674799996, 23.431170976799997, 23.431170976799997, 23.431170976799997, 23.431170976799997, 23.431170976799997, 23.431170976799997, 23.431170976799997, 23.431170976799997, 28.729140804, 28.729140804, 28.729140804, 28.729140804, 28.729140804, 28.729140804, 28.729140804, 28.729140804, 28.729140804, 31.9837009252, 31.9837009252, 31.9837009252, 31.9837009252, 31.9837009252, 31.9837009252, 31.9837009252, 31.9837009252, 40.691919848000005, 40.691919848000005, 40.691919848000005, 40.691919848000005, 40.691919848000005, 40.691919848000005, 40.691919848000005, 40.691919848000005, 47.4670420756, 47.4670420756, 47.4670420756, 47.4670420756, 47.4670420756, 47.4670420756, 47.4670420756, 47.4670420756, 47.4670420756, 50.1891742, 50.1891742, 50.1891742]
  out "CHF file name":string="20210205_150936_RUNIII_CHF20210205_154539_CHF_TEST1.csv"
  out "Graph CHF log 3":T4(graph) caption="XY Graph"
  out "File Refnum (CHF)":refnum<file>
  in  "Tab Control":T15(tab)=enum."Beam heat emulation"
  in  "ƒ¢V / cycle (V)":dbl=0.5 format="%_4f"
  in  "V start (V)":dbl format="%_4f"
  in  "V_end (V)":dbl=65.0 format="%_4f"
  in  "CHF cycle interval (s) (>1s)":dbl=1.0 format="%_3f"
  in  "Data I":T16={"Source"=enum."DMMs", "SourceLabel"="I_H1"}
  in  "Data V":T16={"Source"=enum."DMMs", "SourceLabel"="V_H1"}
  in  "RecordSettings":T17(array[cluster])=[{"Source"=enum."DMMs", "SourceLabel"="I_H1", "FileFormat"="%4.4e"}, {"Source"=enum."DMMs", "SourceLabel"="V_H1", "FileFormat"="%4.4f"}, {"Source"=enum."USB6210", "SourceLabel"="P_3Hepot", "FileFormat"="%4.4e"}, {"Source"=enum."USB6218AI", "SourceLabel"="F_1", "FileFormat"="%4.4f"}, {"Source"=enum."USB6218AI", "SourceLabel"="F_4", "FileFormat"="%4.4f"}, {"Source"=enum."USB6218AI", "SourceLabel"="F_5", "FileFormat"="%4.4f"}, {"Source"=enum."USB6210", "SourceLabel"="DP_HEX4", "FileFormat"="%4.4e"}, {"Source"=enum."LSI336", "SourceLabel"="T3He6-1", "FileFormat"="%4.4f"}, {"Source"=enum."LSI336", "SourceLabel"="T3He6-2", "FileFormat"="%4.4f"}, {"Source"=enum."LSI336", "SourceLabel"="T3He7-1", "FileFormat"="%4.4f"}, {"Source"=enum."LSI336", "SourceLabel"="T3He7-2", "FileFormat"="%4.4f"}, {"Source"=enum."LSI336", "SourceLabel"="T1K3-1", "FileFormat"="%4.4f"}, {"Source"=enum."LSI336", "SourceLabel"="T1K3-2", "FileFormat"="%4.4f"}]
  in  "Data T_high":T16={"Source"=enum."LSI336", "SourceLabel"="T3He7-2"}
  in  "Data T_low":T16={"Source"=enum."LSI336", "SourceLabel"="T3He6-1"}
  out "CHF log file name":string="20210205_150936_RUNIII_20210205_155058_CHFlog.csv"
  in  "STOP CHF":bool
  in  "START CHF":bool=TRUE
  in  "t_off":dbl=20.0 format="%_4f"
  in  "t_on":dbl=30.0 format="%_4f"
  in  "Q_input":dbl=65.0 format="%_4f"
  out "V_input":dbl=65.0 format="%_4f"
  out "R_sample":dbl=65.0 format="%_4f"
  in  "V_sample":dbl=65.0 format="%_4f"
  out "Q_sample":dbl=65.0 format="%_4f"
  in  "I_sample":dbl=1.0 format="%_4f"
  in  "START heater cycle":bool=TRUE
  in  "STOP heater cycle":bool
  out "Series 1":string[](array[string])=["P_ins", "P_4Kres", "P_3HeIN", "P_SldRTN", "P_3Hepot", "P_1Kpot", "P_Dewar(old)", "P_HEX7OUT", "P_IP", "P_Dewar"]
  out "Series 2":string[](array[string])=["DP_HEX4", "DP_HEX5", "L1(old)", "L2-1", "L2-2", "L3", "R_L1", "L1"]
  out "Series 3":string[](array[string])=["F_1", "F_2", "F_3", "F_4", "F_5", "I_CV"]
  out "Series 4":string[](array[string])=["TTH3", "TTH4", "TTH1", "TTH2", "T4He1", "T1K1", "T3He2-1", "T3He2-2", "T4He3-1", "T4He3-2", "T4He3-3", "T4He3-4", "T4He2-1", "T4He2-2", "T4He4", "T1K2", "T1K4", "T1K5", "T3He4", "T1K3-1", "T1K3-2", "T3He5", "T3He8", "T3He6-1", "T3He6-2", "T3He7-1", "T3He7-2"]
  out "Plot errors":errorcluster
  out "LastMeasurementConfig (218)":T18(array[cluster])=[{"LSIName"="LSI218A", "Active?"=TRUE, "LastData"=[286.39, 292.79, 245.71, 242.82, 192.73, 208.05, 129.14, 157.86], "Labels"=["T3He10", "T3He1-1", "TTH3", "TTH4", "TTH1", "TTH2", "T4He1", "T1K1"]}, {"LSIName"="LSI218B", "Active?"=TRUE, "LastData"=[30.0, 0.0, 0.0, 0.0, 214.32, 209.26, 161.19, 290.41], "Labels"=["N.C.", "N.C.", "N.C.", "N.C.", "T3He2-1", "T3He2-2", "T3He3", "T3He1-4"]}, {"LSIName"="LSI218C", "Active?"=TRUE, "LastData"=[293.53, 293.65, 291.53, 291.58, 216.58, 205.59, 215.41, 218.49], "Labels"=["T4He3-1", "T4He3-2", "T4He3-3", "T4He3-4", "T4He2-1", "T4He2-2", "T4He4", "T4He5"]}, {"LSIName"="LSI218D", "Active?"=TRUE, "LastData"=[214.17, 227.11, 292.96, 290.69, 256.79, 281.72, 274.72, 287.38], "Labels"=["T4He6", "T4He9", "T3He1-2", "T3He1-3", "T4He7", "T4He8", "T4He10", "T1K6"]}, {"LSIName"="LSI218E", "Active?"=TRUE, "LastData"=[279.49, 0.0, 232.53, 688.49, 216.83, 149.55, 173.98, 688.58], "Labels"=["TIP1", "N.C.", "TIP2", "N.C.", "TIP3", "TIP4", "TIP5", "N.C."]}, {"LSIName"="LSI218F", "Active?"=TRUE, "LastData"=[178.46, 128.79, 144.74, 152.95, 140.88, 150.1, 0.433, 0.0], "Labels"=["T1K2", "T1K4", "T1K5", "T3He4", "T3He9", "TIP6", "N.C.", "N.C."]}]
  out "DataArrayConv (USB6210)":dbl[][](array[numeric])=[[18.674861858538797, 97865.81349287118, 100998.44453584745, 100709.02551899779, 101407.09548804205, 101279.08758660906, 0.0, -48.20456535494683, 0.06691412080322978, 10.108489682314854, 0.1698011167381339, -0.07483544992953703, 0.04024895650740204, 100273.25274306418, 4.684755546764993e-05, 5.953981760223165]]
  out "LastMeasurementConfig (336)":T18(array[cluster])=[{"LSIName"="LSi336X", "Active?"=TRUE, "LastData"=[117.963, 117.927, 169.419, 129.275], "Labels"=["T1K3-1", "T1K3-2", "T3He5", "T3He8"]}, {"LSIName"="LSi336Y", "Active?"=TRUE, "LastData"=[167.919, 163.1, 162.659, 160.848], "Labels"=["T3He6-1", "T3He6-2", "T3He7-1", "T3He7-2"]}]
  out "DataArrayConv (USB6218)":dbl[][](array[numeric])=[[-0.36185606613019977, -1.4204433335631088, 0.28794373208354185, -3.0973798990583647, 18.382396544680894, -0.0024966396874153696, -25.07402456902091, 102243.79868545999, 107.20664477077275]]
  out "TimeArray (USB6218)":timestamp[](array[timestamp])=[timestamp(3695672639.4136896 s since 1904-01-01)]
  out "Data Array sizes (6210)":i32[](array[numeric])=[1, 16]
  out "DataArraySize (6218)":i32[](array[numeric])=[1, 9]
  out "TimeArray size (6218)":i32=1
  out "TimeArray (LSI336)":timestamp[](array[timestamp])=[timestamp(3695672639.4087214 s since 1904-01-01)]
  out "TimeArray Size (336)":i32=1
  out "DataArray (336)":dbl[][](array[numeric])=[[117.963, 117.927, 169.419, 129.275, 167.919, 163.1, 162.659, 160.848]]
  out "DataArray size (336)":i32[](array[numeric])=[1, 8]
  out "LastData (LSI218)":dbl[](array[numeric])=[286.39, 292.79, 245.71, 242.82, 192.73, 208.05, 129.14, 157.86, 30.0, 0.0, 0.0, 0.0, 214.32, 209.26, 161.19, 290.41, 293.53, 293.65, 291.53, 291.58, 216.58, 205.59, 215.41, 218.49, 214.17, 227.11, 292.96, 290.69, 256.79, 281.72, 274.72, 287.38, 279.49, 0.0, 232.53, 688.49, 216.83, 149.55, 173.98, 688.58, 178.46, 128.79, 144.74, 152.95, 140.88, 150.1, 0.433, 0.0]
  out "TempSensorsLocations":T19(array[ring])=[enum."T3He10", enum."T3He1-1", enum."TTH3", enum."TTH4", enum."TTH1", enum."TTH2", enum."T4He1", enum."T1K1", enum."N.C.", enum."N.C.", enum."N.C.", enum."N.C.", enum."T3He2-1", enum."T3He2-2", enum."T3He3", enum."T3He1-4", enum."T4He3-1", enum."T4He3-2", enum."T4He3-3", enum."T4He3-4", enum."T4He2-1", enum."T4He2-2", enum."T4He4", enum."T4He5", enum."T4He6", enum."T4He9", enum."T3He1-2", enum."T3He1-3", enum."T4He7", enum."T4He8", enum."T4He10", enum."T1K6", enum."TIP1", enum."N.C.", enum."TIP2", enum."N.C.", enum."TIP3", enum."TIP4", enum."TIP5", enum."N.C.", enum."T1K2", enum."T1K4", enum."T1K5", enum."T3He4", enum."T3He9", enum."TIP6", enum."N.C.", enum."N.C.", enum."T1K3-1", enum."T1K3-2", enum."T3He5", enum."T3He8", enum."T3He6-1", enum."T3He6-2", enum."T3He7-1", enum."T3He7-2"]
  out "AllTemperatures":dbl[](array[numeric])=[285.72, 291.98, 244.99, 242.22, 191.48, 206.95, 127.38, 156.15, 30.0, 0.0, 0.0, 0.0, 213.16, 208.05, 159.56, 289.7, 292.82, 292.95, 290.77, 290.83, 215.52, 204.35, 214.31, 217.43, 213.01, 226.25, 292.25, 289.96, 256.33, 281.47, 274.41, 286.82, 279.25, 0.0, 231.74, 688.49, 215.82, 147.93, 172.64, 688.58, 178.09, 127.59, 143.12, 154.09, 137.88, 147.89, 0.433, 0.0, 116.239, 116.203, 167.912, 127.318, 166.258, 161.329, 160.911, 159.065]
  out "error out (frontpanel screenshots)":errorcluster
  out "error out (graph operations)":errorcluster
  out "error out (monthly folder creation)":errorcluster={"status"=TRUE, "code"=10, "source"="Create Folder in CRYO_MASTER_FULL_RUN3.vi<APPEND>\nC:\\LabVIEW\\DATA\\Google\\TUCAN Experiments\\KEK_cryotests_2019-2020\\data\\screenshots\\202102"}
  out "RUN Identifier 7":string="20210209_084357_RUNIII" caption="RUN Identifier"
  out "error out (notifier)":errorcluster
  # "GLOBAL STATUS/CONTROL"
  # "Global Settings"
  # "USB6210 Analog inputs Settings"
  # "USB6218 Analog inputs Settings"
  # "USB6218 Digital Output Settings"
  # "USB6218 Analog Output Settings"
  # "LSI218 Settings"
  # "LSI336 Settings"
  # "HP 34401A (He level meter)"
  # "Graph screenshots"
  # "Configuration"
  # "Activated only when *FIll state* = TRUE"
  # "Activated only when *FIll state* = TRUE"
  # "Vavle Status"
  # "OPEN"
  # "CLOSED"
  # "ADCMT6240A Control/Status"
  # "ADCMT6240A Initialization"
  # "Set Currents (mA)"
  # "PWR400H CTRL via USB6218"
  # "PMC18-3A CTRL via USB621"
  # "DMM configurations"
  # "DMM measurements"
  # "CAUTION: ADCMT 7351 does not have 4-wire resistance measurement function. \n 4-Wire Resistance --> 2-Wire Resistance wih Low Power for this device"
  # "Representative temperatures"
  # "Pressures / Flows"
  # "Labels"
  # "Values"
  # "Helium Levels"
  # "Manual Control of Kenwood"
  # "Automatic Boiling Cruve Measurement"
  # "Before the measurement\n - Intialize Agilent 34402 (FG)\n - Refresh the CHF graph if necessary\n - Go to DMMs tab and check that DMM measurement is running \n - Fill in the CHF measurement parameters below \nThen press START CHF!"
  # "Measurement Configurations"
  # "Channel selection"
  # "Q = I x V"
  # "ƒ¢T = T_high - T_low"
  # "Record Configurations"
  # "Heat emulation"
  # "Before starting, \n - turn off the boiling curve measuremnt on the other tab\n - make sure that the DMMs are running"
  # "Calculator"
  # "Previous measurement:"
  # "Caclulate V which corresponds to derired Q:"
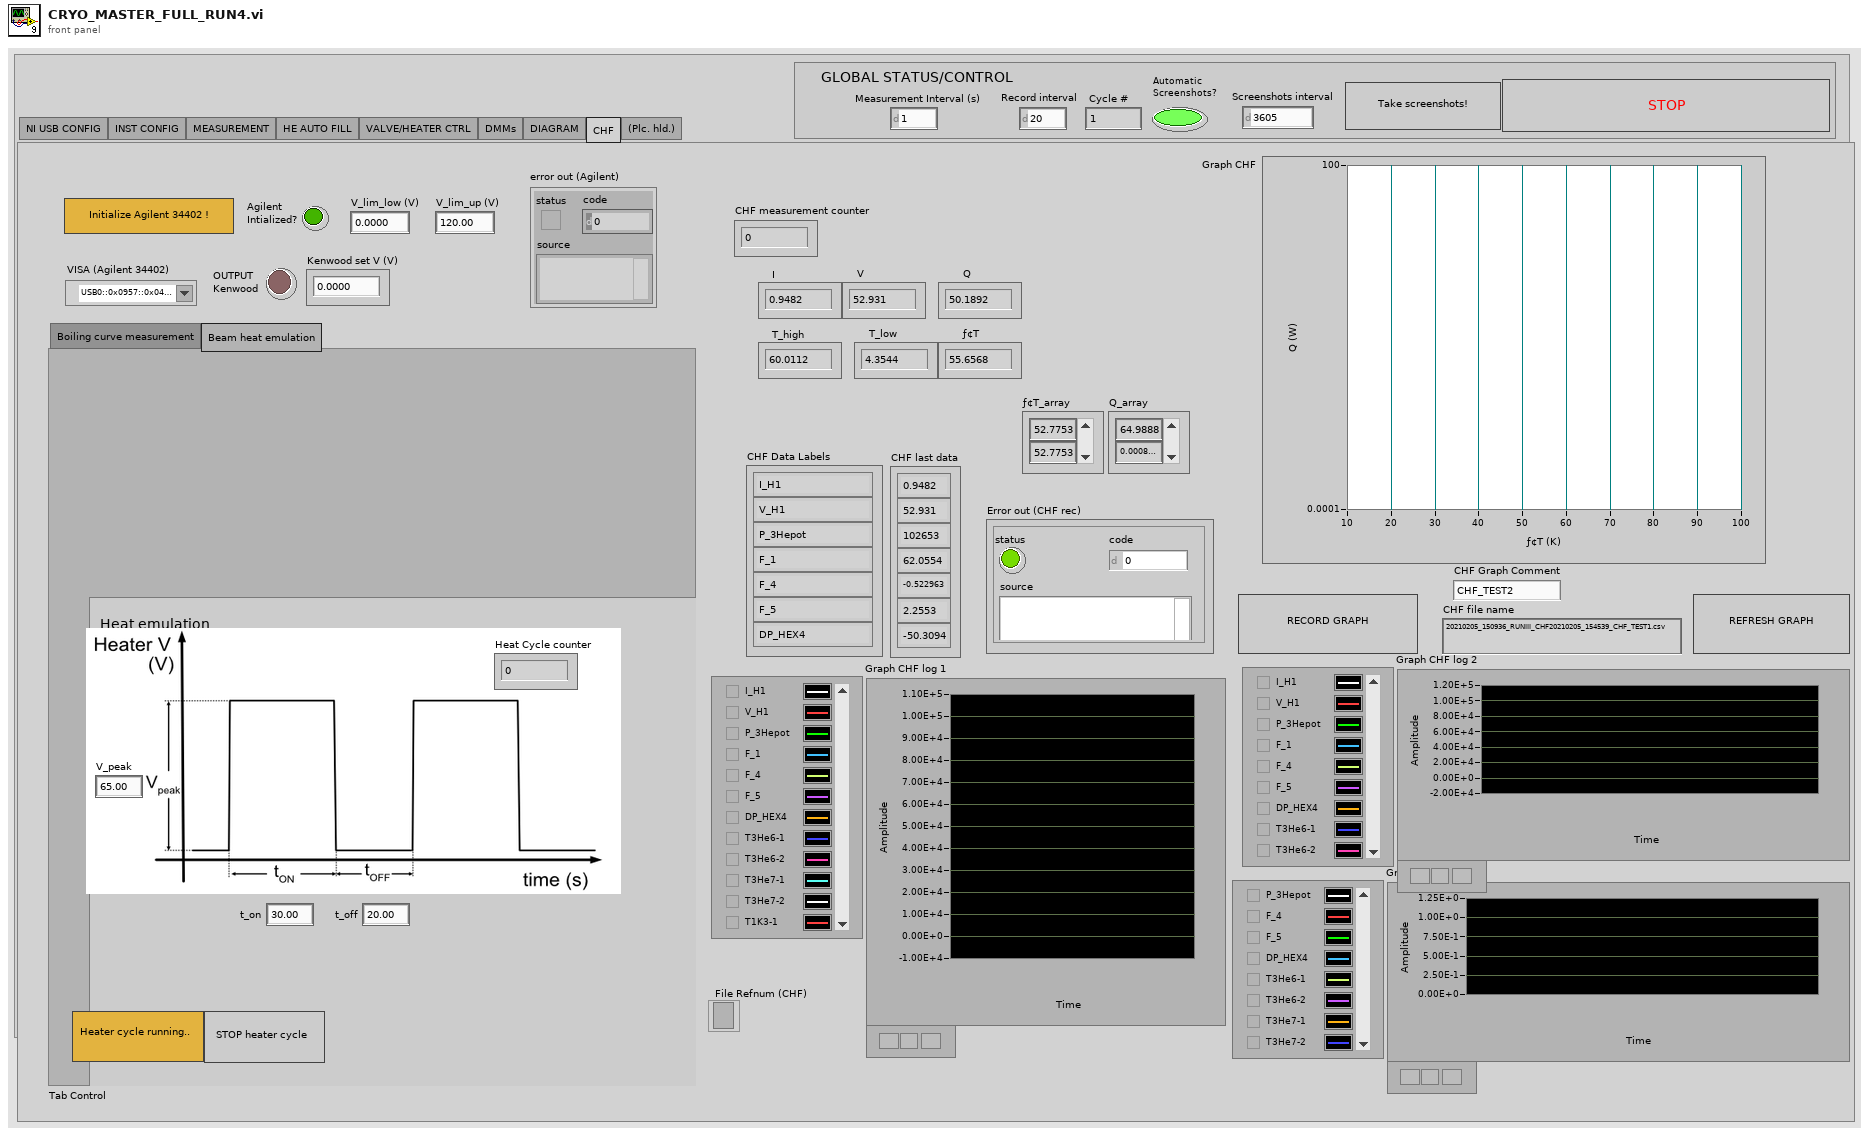
[diagram p1: front panel]
types:
  T1 = enum32{"NI USB CONFIG", "INST CONFIG", "MEASUREMENT", "HE AUTO FILL", "VALVE/HEATER CTRL", "DMMs", "DIAGRAM", "CHF", "(Plc. hld.)"}
  T2 = cluster{"Label":string, "FileFormat":string, "Active?":bool, "Physical CH":tag, " terminal\n type":i32, "ConversionType":cluster{"Type":enum16{"Raw", "SimpleProp", "CC-10_COMBINED", "CC-10_LOG", "LeakDet_EXP", "LeakDet_Mantissa", "Baratron"}, "ConversionParameters":dbl[]}, "VoltageLimits":dbl[]}[]
  T3 = cluster{"LSIName":string, "Labels":string[], "SensorLocations":enum16{"N.C.", "T3He1-1", "T3He1-2", "T3He1-3", "T3He1-4", "T3He2-1", "T3He2-2", "T3He3", "T3He4", "T3He5", "T3He6-1", "T3He6-2", "T3He7-1", "T3He7-2", "T3He8", "T3He9", "T3He10", "T4He1", "T4He2-1", "T4He2-2", "T4He3-1", "T4He3-2", "T4He3-3", "T4He3-4", "T4He4", "T4He5", "T4He6", "T4He7", "T4He8", "T4He9", "T4He10", "T1K1", "T1K2", "T1K3-1", "T1K3-2", "T1K4", "T1K5", "T1K6", "TIP1", "TIP2", "TIP3", "TIP4", "TIP5", "TIP6", "TIP7", "TTH1", "TTH2", "TTH3", "TTH4"}[], "Active?":bool, "VISA res. name":refnum<visa-resource-name>}[]
  T4 = cluster{"TimeArray":timestamp[], "DataArray":dbl[]}[]
  T5 = enum32{"USB6210", "USB6218", "Temeprature (1)", "Temperature (2)", "Temperature (3)"}
  T6 = enum16{"Intialized", "Ready", "Measuring", "Terminated"}
  T7 = enum16{"Initialized", "Ready", "Measuring", "Terminated"}
  T8 = enum16{"USB6210", "USB6218AI", "USB6218AO", "LSI218", "LSI336"}
  T9 = cluster{"TimeArray":timestamp[], "Filtered X":dbl[]}[]
  T10 = cluster{"TimeArray (USB6218)":timestamp[], "DataArrayConv (USB6218)":dbl[]}[]
  T11 = cluster{"Label":string, "Active?":bool, "VISA resource name":refnum<visa-resource-name>, "Device":enum16{"Agilent34401A", "ADCMT7351", "HP3478A", "ADCMT7451"}, "Measurement":enum16{"DC Volts", "DC Currents", "2-Wire Resistance", "4-Wire Resistance"}, "FileFormat":string}[]
  T12 = enum16{"USB6210", "USB6218AI", "USB6218AO", "LSI218", "LSI336"}[]
  T13 = cluster{"Label":string, "Active?":bool, "Source":enum16{"USB6210", "USB6218AI", "USB6218AO", "LSI218", "LSI336"}, "SourceLabel":string, "FileFormat":string}[]
  T14 = enum16{"N.C.", "T3He1-1", "T3He1-2", "T3He1-3", "T3He1-4", "T3He2-1", "T3He2-2", "T3He3", "T3He4", "T3He5", "T3He6-1", "T3He6-2", "T3He7-1", "T3He7-2", "T3He8", "T3He9", "T3He10", "T4He1", "T4He2-1", "T4He2-2", "T4He3-1", "T4He3-2", "T4He3-3", "T4He3-4", "T4He4", "T4He5", "T4He6", "T4He7", "T4He8", "T4He9", "T4He10", "T1K1", "T1K2", "T1K3-1", "T1K3-2", "T1K4", "T1K5", "T1K6", "TIP1", "TIP2", "TIP3", "TIP4", "TIP5", "TIP6", "TIP7", "TTH1", "TTH2", "TTH3", "TTH4"}
  T15 = enum32{"Boiling curve measurement", "Beam heat emulation"}
  T16 = cluster{"Source":enum16{"USB6210", "USB6218AI", "USB6218AO", "LSI218", "LSI336", "DMMs"}, "SourceLabel":string}
  T17 = cluster{"Source":enum16{"USB6210", "USB6218AI", "USB6218AO", "LSI218", "LSI336", "DMMs"}, "SourceLabel":string, "FileFormat":string}[]
  T18 = cluster{"LSIName":string, "Active?":bool, "LastData":dbl[], "Labels":string[]}[]
  T19 = enum16{"N.C.", "T3He1-1", "T3He1-2", "T3He1-3", "T3He1-4", "T3He2-1", "T3He2-2", "T3He3", "T3He4", "T3He5", "T3He6-1", "T3He6-2", "T3He7-1", "T3He7-2", "T3He8", "T3He9", "T3He10", "T4He1", "T4He2-1", "T4He2-2", "T4He3-1", "T4He3-2", "T4He3-3", "T4He3-4", "T4He4", "T4He5", "T4He6", "T4He7", "T4He8", "T4He9", "T4He10", "T1K1", "T1K2", "T1K3-1", "T1K3-2", "T1K4", "T1K5", "T1K6", "TIP1", "TIP2", "TIP3", "TIP4", "TIP5", "TIP6", "TIP7", "TTH1", "TTH2", "TTH3", "TTH4"}[]
  T20 = cluster{"TimeArray (USB6218)":timestamp[], "DataArrayConv (USB6218)":dbl[]}
  T21 = cluster{"appended array":timestamp[], "ActualCurrentArray":dbl[]}
  T22 = cluster{"appended array":timestamp[], "SetCurrentArray":dbl[]}
  T23 = cluster{"appended array":timestamp[], "SetCurrentArray":dbl[]}[]
  T24 = typedef "imagedata.ctl" = cluster{"image type":i32, "image depth":i32, "image":u8[], "mask":u8[], "colors":u32[], "Rectangle":cluster{"left":i16, "top":i16, "right":i16, "bottom":i16}}
  T25 = enum16{"open", "replace", "create", "open or create", "replace or create", "replace or create with confirmation"}
  T26 = cluster{"TimeArray":timestamp[], "DataArrayConv":dbl[]}[]
  T27 = cluster{"IndexArray":i64[], "TimeArray":timestamp[], "DataArrayRaw":dbl[][], "DataArrayConv":dbl[][], "LDArray":dbl[]}
  T28 = cluster{"InstName":string, "Active?":bool, "Status":enum16{"Intialized", "Ready", "Measuring", "Terminated"}, "Labels":string[], "LabelLD":string, "FileFormat":string[], "FileFormatLD":string, "ReadLeakDet?":bool}
  T29 = cluster{"AOUT Labels[0]":string, "AOUT Labels[1]":string, "AOUT Labels[2]":string, "AOUT Labels[3]":string, "AOUT Labels[4]":string, "AOUT Labels[5]":string, "AOUT Labels[6]":string, "AOUT Labels[7]":string, "AOUT Labels[8]":string}
  T30 = cluster{"LastTimeArray":timestamp[], "LastDataArray":dbl[]}
  T31 = cluster{"LastTimeArray":timestamp[], "LastDataArray":dbl[]}[]
  T32 = cluster{"TimeArray":timestamp[], "DataArrayConv":dbl[]}
  T33 = cluster{"TimeArray":timestamp[], "DataArrayConv (USB6218)":dbl[]}
  T34 = cluster{"TimeArray":timestamp[], "M.A. Array":dbl[]}
  T35 = cluster{"TimeArray":timestamp[], "M.A. Array":dbl[]}[]
  T36 = cluster{"TimeArray":timestamp[], "DataArray":dbl[]}
  T37 = enum16{"USB6210", "USB6218AI", "USB6218AO", "LSI218", "LSI336", "DMMs"}
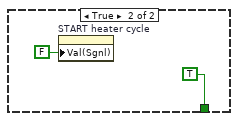
[diagram p3: hidden frame]
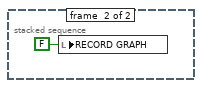
[diagram p5: hidden frame]
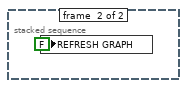
[diagram p7: hidden frame]
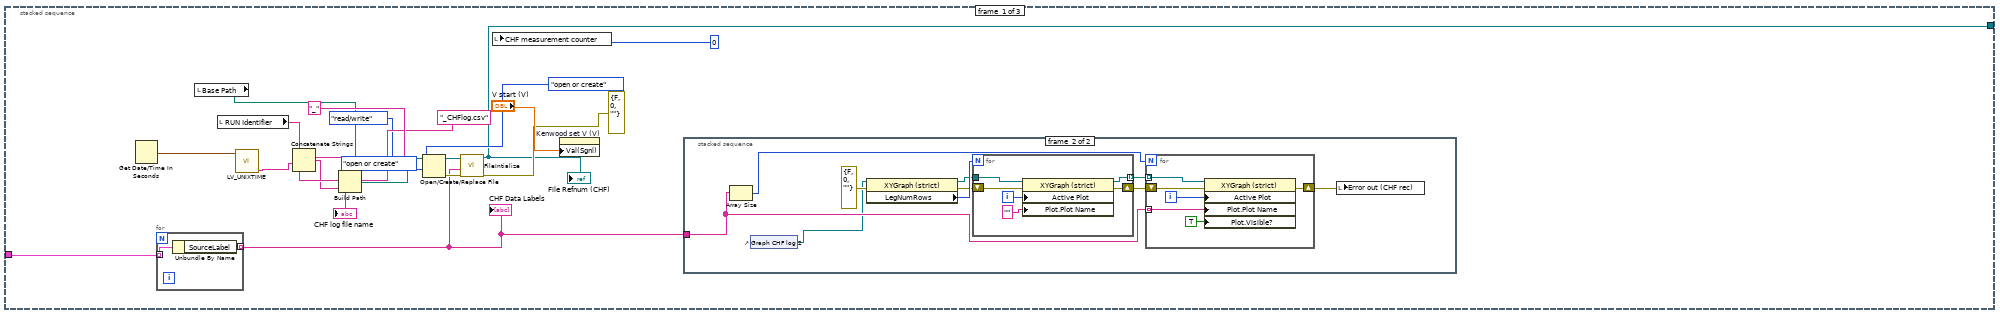
[diagram p9: hidden frame]
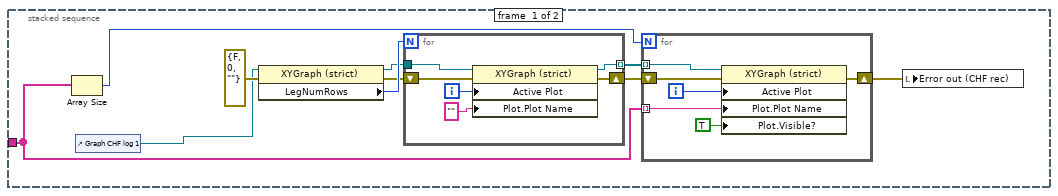
[diagram p10: hidden frame]
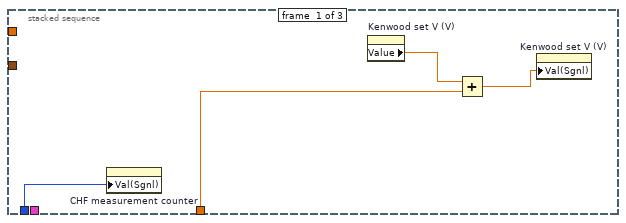
[diagram p11: hidden frame]
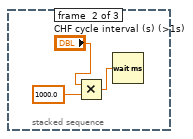
[diagram p12: hidden frame]
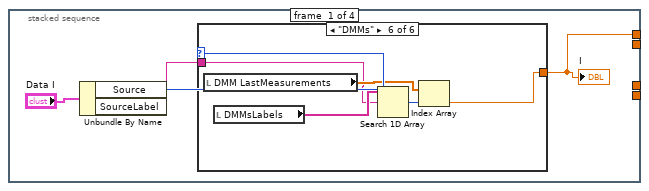
[diagram p13: hidden frame]
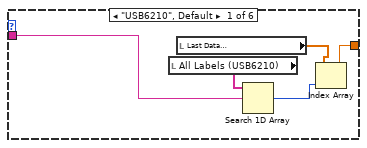
[diagram p14: hidden frame]
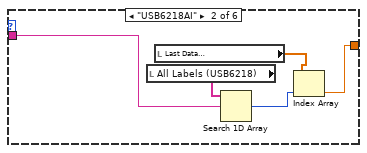
[diagram p15: hidden frame]
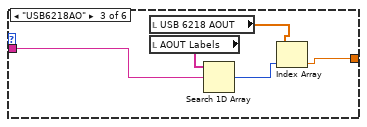
[diagram p16: hidden frame]
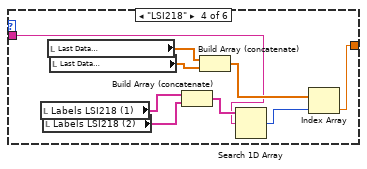
[diagram p17: hidden frame]
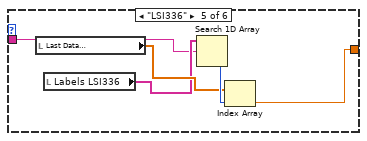
[diagram p18: hidden frame]
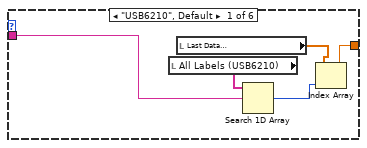
[diagram p19: hidden frame]
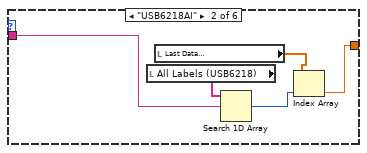
[diagram p20: hidden frame]
diagram:
  w17 = TRUE ("create if not found? (T)")
  w21 = errorcluster {"status"=FALSE, "code"=0, "source"=""} ("error in (no error)")
  w6 = errorcluster {"status"=FALSE, "code"=0, "source"=""} ("error in (no error)")
  n1 = while {
    shift-right: [w44] -> _
    shift-left: dbl[] [] -> [w50]
    shift-right: [w47] -> _
    shift-left: timestamp[] [] -> [w49]
    i -> [w48]
    stop <- w51 stop-if-true
    n2 = Wait (ms)(milliseconds to wait=u32 225) -> ()  [unwired: 1 out]
    n3 = event shown="[6] \"OUTPUT (PWR)\", \"OUTPUT (PMC)\": Value Change" {
      selector: _ -> [_ _ _ _ _ _ _]
      dyn-events: _ -> [_ _ _ _ _ _ _]
      timeout: _ -> [_ _ _ _ _ _ _]
      tunnel: [_ TRUE _ _ _ _ _] -> w51
      tunnel: w48 -> [_ _ _ _ w132 _ _]
      tunnel: [_ _ _ _ w131 w215 _] -> w44
      tunnel: w50 -> [_ _ _ _ w128 w215 _]
      tunnel: [w53 w63 _ _ w130 w214 w218] -> w47
      tunnel: w49 -> [w53 w63 _ _ w129 w214 w218]
      tunnel: w48 -> [_ _ w69 w93 _ _ w219]
      tunnel: [_ _ _ _ w119 _ _] -> w43
      event Timeout {
        n4 = event-data() -> ()  [unwired: 1 in, 3 out]
      }
      event "Stop Button": Value Change {
        w54 = FALSE
        n5 = event-data() -> ()  [unwired: 1 in, 3 out]
        n6 = local read "error out (USB6210/6218 DOUT)"() -> (w62:errorcluster)
        n7 = local read "error out (USB6210/6218 AOUT)"() -> (w59:errorcluster)
        n8 = local read "DOUT task out"() -> (w58:refnum<k21>)
        n9 = local read "AO task out"() -> (w65:refnum<k21>)
        n10 = property on="OUTPUT\n(PWR)" class="Bool (strict)"("Value"=w54) -> ()  [unwired: 2 in, 2 out]
        n11 = property on="V2 (N.C.)" class="Bool (strict)"("Val(Sgnl)"=w54) -> ()  [unwired: 2 in, 2 out]
        n12 = property on="OUTPUT\n(PMC)" class="Bool (strict)"("Value"=w54) -> ()  [unwired: 2 in, 2 out]
        n13 = Build Array(w54, w54, w54, w54) -> (w61:bool[])
        n14 = Not(x=w54) -> (.not. x?=w55:bool)
        n15 = call <vilib>:"DAQmx Clear Task.vi"("task in"=w65, "error in"=w59) -> ("error out"=w64:errorcluster)  [unwired: 13 in]
        n16 = property on="V1 (N.O.)" class="Bool (strict)"("Val(Sgnl)"=w55) -> ()  [unwired: 2 in, 2 out]
        n17 = call <vilib>:"DAQmx Write (Digital 1D Bool NChan 1Samp 1Line).vi"("task/channels in"=w58, "data"=w61, "timeout"=10.0, "error in"=w62) -> ("task out"=w57:refnum<k21>, "error out"=w56:errorcluster)  [unwired: 9 in, 1 out]
        n18 = call <vilib>:"DAQmx Clear Task.vi"("task in"=w57, "error in"=w56) -> ("error out"=w66:errorcluster)  [unwired: 13 in]
        n19 = local write "error out (USB6210/6218 AOUT)"(w64) -> ()
        n20 = local write "error out (USB6210/6218 DOUT)"(w66) -> ()
      }
      event "V1 (N.O.)": Value Change {
        n21 = event-data() -> ()  [unwired: 1 in, 3 out]
        n22 = local read "Cycle #"() -> (w72:u32)
        n23 = Greater?(x=w72, y=u32 0) -> (0:w70:bool)
        n24 = case shown="True" w70 {
          tunnel: "V1 (N.O.)" -> [_ w86]
          tunnel: w69 -> [_ w81]
          frame False {
          }
          frame True {
            n25 = Not(x=w86) -> (.not. x?=w88:bool)
            n26 = property on="OUTPUT\n(PMC)" class="Bool (strict)"() -> ("Value"=w73:bool)  [unwired: 2 in, 2 out]
            n27 = local read "error out (USB6210/6218 DOUT)"() -> (w87:errorcluster)
            n28 = property on="OUTPUT\n(PWR)" class="Bool (strict)"() -> ("Value"=w84:bool)  [unwired: 2 in, 2 out]
            n29 = property on="V2 (N.C.)" class="Bool (strict)"() -> ("Value"=w85:bool)  [unwired: 2 in, 2 out]
            n30 = local read "DOUT task out"() -> (w91:refnum<k21>)
            n31 = Build Array(w88, w85, w84, w73) -> (w77:bool[])
            n32 = local read "File Refn USB DO"() -> (w82:refnum<file>)
            n33 = Boolean To (0,1)(Boolean=w77) -> (0, 1=w76:i16[])
            n34 = Initialize Array("%d" ("element"), 3 ("dimension size")) -> (w80:string[])
            n35 = call <vilib>:"DAQmx Write (Digital 1D Bool NChan 1Samp 1Line).vi"("task/channels in"=w91, "data"=w77, "timeout"=10.0, "error in"=w87) -> ("task out"=w89:refnum<k21>, "error out"=w75:errorcluster)  [unwired: 9 in, 1 out]
            n36 = local write "DOUT task out"(w89) -> ()
            n37 = Get Date/Time In Seconds() -> (seconds since 1Jan1904=w83:timestamp)
            n38 = call "FileWrite.vi"("DataArray"=w76, "Time Stamp"=w83, "Error In"=w75, "FileFormat"=w80, "Index"=w81, "refnum in"=w82) -> ("Error Out"=w74:errorcluster)  [unwired: 4 in, 1 out]
            n39 = local write "error out (USB6210/6218 DOUT)"(w74) -> ()
          }
        }
        "V1" <- "V1 (N.O.)"
      }
      event "V2 (N.C.)": Value Change {
        n40 = event-data() -> ()  [unwired: 1 in, 3 out]
        n41 = local read "Cycle #"() -> (w96:u32)
        n42 = Greater?(x=w96, y=u32 0) -> (0:w94:bool)
        n43 = case shown="True" w94 {
          tunnel: "V2 (N.C.)" -> [_ w111]
          tunnel: w93 -> [_ w103]
          frame False {
          }
          frame True {
            n44 = property on="OUTPUT\n(PMC)" class="Bool (strict)"() -> ("Value"=w97:bool)  [unwired: 2 in, 2 out]
            n45 = property on="V1 (N.O.)" class="Bool (strict)"() -> ("Value"=w110:bool)  [unwired: 2 in, 2 out]
            n46 = Not(x=w110) -> (.not. x?=w109:bool)
            n47 = local read "error out (USB6210/6218 DOUT)"() -> (w114:errorcluster)
            n48 = property on="OUTPUT\n(PWR)" class="Bool (strict)"() -> ("Value"=w108:bool)  [unwired: 2 in, 2 out]
            n49 = local read "DOUT task out"() -> (w115:refnum<k21>)
            n50 = Build Array(w109, w111, w108, w97) -> (w106:bool[])
            n51 = local read "File Refn USB DO"() -> (w107:refnum<file>)
            n52 = Boolean To (0,1)(Boolean=w106) -> (0, 1=w105:i16[])
            n53 = Initialize Array("%d" ("element"), 3 ("dimension size")) -> (w100:string[])
            n54 = call <vilib>:"DAQmx Write (Digital 1D Bool NChan 1Samp 1Line).vi"("task/channels in"=w115, "data"=w106, "timeout"=10.0, "error in"=w114) -> ("task out"=w112:refnum<k21>, "error out"=w99:errorcluster)  [unwired: 9 in, 1 out]
            n55 = local write "DOUT task out"(w112) -> ()
            n56 = Get Date/Time In Seconds() -> (seconds since 1Jan1904=w104:timestamp)
            n57 = call "FileWrite.vi"("DataArray"=w105, "Time Stamp"=w104, "Error In"=w99, "FileFormat"=w100, "Index"=w103, "refnum in"=w107) -> ("Error Out"=w98:errorcluster)  [unwired: 4 in, 1 out]
            n58 = local write "error out (USB6210/6218 DOUT)"(w98) -> ()
          }
        }
        "V2" <- "V2 (N.C.)"
      }
      event "Set Current (mA)\n (PMC)", "Set Current (mA)\n (PWR)", "update current": Value Change {
        n59 = event-data() -> ()  [unwired: 1 in, 3 out]
        n60 = case shown="True" "CONTROL KIKUSUI?" {
          tunnel: w132 -> [_ w183]
          tunnel: [w142 w176] -> w131
          tunnel: [w145 w175] -> w130
          tunnel: w129 -> [w147 w178]
          tunnel: w128 -> [w143 w177]
          tunnel: "Set Current (mA)\n (PWR)" -> [_ w155]
          tunnel: "Set Current (mA)\n (PMC)" -> [_ w159]
          frame False {
            w144 = 0.0 ("element")
            n61 = Get Date/Time In Seconds() -> (seconds since 1Jan1904=w146:timestamp)
            n62 = local read "AO task out"() -> (w152:refnum<k21>)
            n63 = Build Array (concatenate)(w147, w146) -> (w145:timestamp[])
            n64 = Build Array (concatenate)(w143, w144) -> (w142:dbl[])
            n65 = Build Array(w144, w144) -> (w150:dbl[])
            n66 = call <vilib>:"DAQmx Write (Analog 1D DBL NChan 1Samp).vi"("task/channels in"=w152, "data"=w150, "timeout"=100.0, "error in"=errorcluster {"status"=FALSE, "code"=0, "source"=""}) -> ("task out"=w153:refnum<k21>, "error out"=w148:errorcluster)  [unwired: 9 in, 1 out]
            n67 = local write "AO task out"(w153) -> ()
            n68 = local write "error out (KIKUSI CTRL)"(w148) -> ()
          }
          frame True {
            w170 = 2 ("index")
            n69 = xnode "Formula"("X1"=w155) -> ("Result"=w172:dbl)  [unwired: 1 in, 1 out]
            n70 = xnode "Formula"("X1"=w159) -> ("Result"=w166:dbl)  [unwired: 1 in, 1 out]
            n71 = Build Array (concatenate)(w177, w155) -> (w176:dbl[])
            n72 = In Range and Coerce(upper limit=10.0, x=w172, lower limit=0.0 ("y")) -> (coerced(x)=w164:dbl, In Range?=w165:bool)
            n73 = In Range and Coerce(upper limit=10.0, x=w166, lower limit=0.0 ("y")) -> (coerced(x)=w161:dbl, In Range?=w162:bool)
            n74 = case shown="False" w165 {
              tunnel: w164 -> [_ w195]
              tunnel: [0.0 ("upper limit") w195] -> w163
              frame False {
              }
              frame True {
              }
            }
            n75 = case shown="True" w162 {
              tunnel: w161 -> [_ w193]
              tunnel: [0.0 ("upper limit") w193] -> w160
              frame False {
              }
              frame True {
              }
            }
            n76 = Multiply(x=w155, y=0.001) -> (x*y=w154:dbl)
            n77 = Multiply(x=w159, y=0.001) -> (x*y=w158:dbl)
            n78 = local read "File Refn USB AO"() -> (w184:refnum<file>)
            n79 = Build Array(w154, w158, w163, w160) -> (w171:dbl[])
            "USB 6218 AOUT" <- w171
            n80 = Initialize Array("%.3f", 4 ("dimension size")) -> (w185:string[])
            n81 = Get Date/Time In Seconds() -> (seconds since 1Jan1904=w179:timestamp)
            n82 = local read "AO task out"() -> (w189:refnum<k21>)
            n83 = call "FileWrite.vi"("DataArray"=w171, "Time Stamp"=w179, "Error In"=errorcluster {"status"=FALSE, "code"=0, "source"=""} ("error in"), "FileFormat"=w185, "Index"=w183, "refnum in"=w184) -> ("Error Out"=w181:errorcluster, "Byte Stream File Refnum"=w180:refnum<file>)  [unwired: 4 in]
            n84 = Build Array (concatenate)(w178, w179) -> (w175:timestamp[])
            n85 = Array Subset(array=w171, index=w170, length=w170) -> (w169:dbl[])
            n86 = local write "File Refn USB AO"(w180) -> ()
            n87 = call <vilib>:"DAQmx Write (Analog 1D DBL NChan 1Samp).vi"("task/channels in"=w189, "data"=w169, "timeout"=100.0, "error in"=w181) -> ("task out"=w190:refnum<k21>, "error out"=→"error out (KIKUSI CTRL)":errorcluster)  [unwired: 9 in, 1 out]
            n88 = local write "AO task out"(w190) -> ()
          }
        }
        n89 = local read "All Labels (USB6218)"() -> (w125:string[])
        n90 = local read "DataArrayConv (USB6218)"() -> (w124:dbl[][])
        n91 = local read "Last Data \n(USB6218)"() -> (w121:dbl[])
        n92 = local read "TimeArray (USB6218)"() -> (w122:timestamp[])
        n93 = Search 1D Array(1D array=w125, element="I_CV") -> (index of element=w126:i32)  [unwired: 1 in]
        n94 = Index Array(array=w124, index (row)=w126) -> (element=w123:dbl[])  [unwired: 1 in]
        n95 = Index Array(array=w121, index=w126) -> (element=w118:dbl)
        n96 = Bundle("TimeArray (USB6218)"=w122, "DataArrayConv (USB6218)"=w123) -> (w119:T20)  [unwired: 1 in]
        n97 = xnode "Formula"("X1"=w118) -> ("Result"=→"Monitor Current (mA)":dbl)  [unwired: 1 in, 1 out]
      }
      event "upper limit (mA)\n (PWR)", "lower limit (mA) \n(PWR)": Value Change {
        n98 = event-data() -> ()  [unwired: 1 in, 6 out]
        n99 = property on="Set Current (mA)\n (PWR)" class="DigNum (strict)"("Maximum"="upper limit (mA)\n (PWR)", "Minimum"="lower limit (mA) \n(PWR)") -> ()  [unwired: 2 in, 2 out]
        n100 = property on="Set Current (mA)\n (PMC)" class="DigNum (strict)"("Maximum"="upper limit (mA)\n (PMC)", "Minimum"="lower limit (mA) \n(PMC)") -> ()  [unwired: 2 in, 2 out]
      }
      event "OUTPUT\n(PWR)", "OUTPUT\n(PMC)": Value Change {
        n101 = event-data() -> ()  [unwired: 1 in, 6 out]
        n102 = local read "Cycle #"() -> (w222:u32)
        n103 = Greater?(x=w222, y=u32 0) -> (0:w220:bool)
        n104 = case shown="True" w220 {
          tunnel: w219 -> [_ w227]
          frame False {
          }
          frame True {
            n105 = property on="V1 (N.O.)" class="Bool (strict)"() -> ("Value"=w238:bool)  [unwired: 2 in, 2 out]
            n106 = Not(x=w238) -> (.not. x?=w237:bool)
            n107 = local read "error out (USB6210/6218 DOUT)"() -> (w241:errorcluster)
            n108 = property on="V2 (N.C.)" class="Bool (strict)"() -> ("Value"=w236:bool)  [unwired: 2 in, 2 out]
            n109 = local read "DOUT task out"() -> (w242:refnum<k21>)
            n110 = Build Array(w237, w236, "OUTPUT\n(PWR)", "OUTPUT\n(PMC)") -> (w225:bool[])
            n111 = local read "File Refn USB DO"() -> (w228:refnum<file>)
            n112 = Boolean To (0,1)(Boolean=w225) -> (0, 1=w224:i16[])
            n113 = call <vilib>:"DAQmx Write (Digital 1D Bool NChan 1Samp 1Line).vi"("task/channels in"=w242, "data"=w225, "timeout"=10.0, "error in"=w241) -> ("task out"=w239:refnum<k21>, "error out"=w232:errorcluster)  [unwired: 9 in, 1 out]
            n114 = Initialize Array("%d" ("element"), 3 ("dimension size")) -> (w230:string[])
            n115 = local write "DOUT task out"(w239) -> ()
            n116 = Get Date/Time In Seconds() -> (seconds since 1Jan1904=w229:timestamp)
            n117 = call "FileWrite.vi"("DataArray"=w224, "Time Stamp"=w229, "Error In"=w232, "FileFormat"=w230, "Index"=w227, "refnum in"=w228) -> ("Error Out"=w231:errorcluster, "Byte Stream File Refnum"=w226:refnum<file>)  [unwired: 4 in]
            n118 = local write "File Refn USB DO"(w226) -> ()
            n119 = local write "error out (USB6210/6218 DOUT)"(w231) -> ()
          }
        }
      }
    }
    n120 = Bundle(w47, w44) -> (w46:cluster{timestamp[], dbl[]})  [unwired: 1 in]
    n121 = Build Array(w46, w43) -> (→"Graph 7":T10)
  }
  n122 = while {
    shift-right: [w251] -> _
    shift-left: refnum<class "6240AData.lvclass"> refnum ("6240AData.lvclass") -> [w249]
    shift-right: [w247] -> _
    shift-left: errorcluster {"status"=FALSE, "code"=0, "source"=""} ("error in (no error)") -> [w248]
    i -> [w243]
    stop <- w250 stop-if-true
    n123 = Wait (ms)(milliseconds to wait=u32 231) -> ()  [unwired: 1 out]
    n124 = Equal?(x=w243, y=0) -> (x = y?=w245:bool)
    n125 = case shown="True" w245 {
      frame False {
      }
      frame True {
        n126 = property on="Initialized?" class="Bool (strict)"("Val(Sgnl)"=FALSE ("Value (Signaling)")) -> ()  [unwired: 2 in, 2 out]
      }
    }
    n127 = event shown="[2] \"upper limit (mA)\", \"lower limit (mA)\": Value Change" {
      selector: _ -> [_ _ _ _ _]
      dyn-events: _ -> [_ _ _ _ _]
      timeout: _ -> [_ _ _ _ _]
      tunnel: [w254 w269 _ w318 w339] -> w251
      tunnel: [_ _ _ _ TRUE ("Value (Signaling)")] -> w250
      tunnel: w249 -> [w254 w268 _ w302 w337]
      tunnel: w248 -> [w253 w267 _ w301 w335]
      tunnel: [w253 w266 _ w316 w338] -> w247
      tunnel: w243 -> [_ w265 _ _ _]
      tunnel: w243 -> [_ _ _ w310 _]
      event Timeout {
        n128 = event-data() -> ()  [unwired: 1 in, 3 out]
      }
      event "update values", "SetCurrent 1 (mA)", "SetCurrent 2 (mA)": Value Change {
        w258 = 1000.0 ("y")
        n129 = event-data() -> ()  [unwired: 1 in, 6 out]
        n130 = local read "Initialized?"() -> (w264:bool)
        n131 = Divide(x="SetCurrent 1 (mA)", y=w258) -> (x/y=w259:dbl)
        n132 = Divide(x="SetCurrent 2 (mA)", y=w258) -> (x/y=w260:dbl)
        n133 = Build Array(w259, w260) -> (w257:dbl[])
        n134 = Not Equal?(x=w264, y=FALSE) -> (x != y?=w262:bool)
        n135 = case shown="True" w262 {
          tunnel: [w271 w295] -> w269
          tunnel: "Output\n (ADCMT)" -> [_ w294]
          tunnel: w268 -> [w271 w293]
          tunnel: w267 -> [w270 w292]
          tunnel: [w270 w291] -> w266
          tunnel: w265 -> [_ w287]
          tunnel: w257 -> [_ w273]
          frame False {
          }
          frame True {
            w280 = 1 ("index (col)")
            w281 = 0 ("disabled index (col)")
            n136 = call-dynamic "6240AData_execute.vi"("6240AData in"=w293, "SetCurrent (A)"=w273, "FileFormat"="%3.5f", "Output status"=w294, "ExecutionIndex"=w287, "error in (no error)"=w292) -> ("ActualVoltage (V)"=w272:dbl[], "ActualCurrent (A)"=w286:dbl[], "6240AData out"=w295:refnum<class "6240AData.lvclass">, "appended array"=w276:timestamp[], "SetCurrentArray"=w282:dbl[][], "ActualCurrentArray"=w289:dbl[][], "error out"=w291:errorcluster)  [unwired: 3 in]
            n137 = property on="ActualVoltage (V)" class="Arr (strict)"("Val(Sgnl)"=w272) -> ()  [unwired: 2 in, 2 out]
            n138 = property on="ActualCurrent (A)" class="Arr (strict)"("Val(Sgnl)"=w286) -> ()  [unwired: 2 in, 2 out]
            n139 = Index Array(array=w289, index (col) #1=w281, index (col) #2=w280) -> (element #1=w290:dbl[], element #2=w284:dbl[])  [unwired: 2 in]
            n140 = Index Array(array=w282, index (col) #1=w281, index (col) #2=w280) -> (element #1=w278:dbl[], element #2=w275:dbl[])  [unwired: 2 in]
            n141 = Bundle("appended array"=w276, "ActualCurrentArray"=w290) -> (w285:T21)  [unwired: 1 in]
            n142 = Bundle("appended array"=w276, "ActualCurrentArray"=w284) -> (w279:T21)  [unwired: 1 in]
            n143 = Bundle("appended array"=w276, "SetCurrentArray"=w278) -> (w277:T22)  [unwired: 1 in]
            n144 = Bundle("appended array"=w276, "SetCurrentArray"=w275) -> (w274:T22)  [unwired: 1 in]
            n145 = Build Array(w285, w279, w277, w274) -> (→"Graph 6":T23)
          }
        }
      }
      event "upper limit (mA)", "lower limit (mA)": Value Change {
        n146 = event-data() -> ()  [unwired: 1 in, 6 out]
        n147 = property on="SetCurrent 1 (mA)" class="DigNum (strict)"("Maximum"="upper limit (mA)", "Minimum"="lower limit (mA)") -> ()  [unwired: 2 in, 2 out]
        n148 = property on="SetCurrent 2 (mA)" class="DigNum (strict)"("Maximum"="upper limit (mA)", "Minimum"="lower limit (mA)") -> ()  [unwired: 2 in, 2 out]
      }
      event "Initialize": Value Change {
        w312 = FALSE
        n149 = event-data() -> ()  [unwired: 1 in, 6 out]
        n150 = local read "Initialized?"() -> (w300:bool)
        n151 = case shown="True" w300 {
          tunnel: w302 -> [w328 w332]
          tunnel: w301 -> [w327 w331]
          tunnel: [w328 w330] -> w299
          tunnel: [w327 w329] -> w298
          frame False {
          }
          frame True {
            n152 = call-dynamic "6240AData_terrminate.vi"("error in (no error)"=w331, "6240AData in"=w332) -> ("error out"=w329:errorcluster, "6240AData out"=w330:refnum<class "6240AData.lvclass">)  [unwired: 8 in]
          }
        }
        n153 = property on="Initialized?" class="Bool (strict)"("Val(Sgnl)"=TRUE ("Value (Signaling)")) -> ()  [unwired: 2 in, 2 out]
        n154 = local read "SetCurrent 2 (mA)"() -> (w305:dbl)
        n155 = local read "SetCurrent 1 (mA)"() -> (w308:dbl)
        n156 = local read "RUN Identifier"() -> (w320:string)
        n157 = local read "Base Path"() -> (w321:path)
        n158 = Divide(x=w308, y=1000.0) -> (x/y=w307:dbl)
        n159 = Divide(x=w305, y=1000.0) -> (x/y=w304:dbl)
        n160 = Get Date/Time In Seconds() -> ()  [unwired: 1 out]
        n161 = call-dynamic "6240AData_initialize.vi"("6240AData in"=w299, "RunIdentifier"=w320, "InstName"="InstName", "base path"=w321, "VISA"="VISA", "error in (no error)"=w298, "CtrlLabels"="CtrlLabels", "Voltage limits (V)"="Voltage limits (V)") -> ("6240AData out"=w319:refnum<class "6240AData.lvclass">, "error out"=w317:errorcluster)  [unwired: 6 in]
        n162 = Build Array(w307, w304) -> (w303:dbl[])
        n163 = Build Array(w312, w312) -> (w311:bool[])
        n164 = call-dynamic "6240AData_execute.vi"("6240AData in"=w319, "SetCurrent (A)"=w303, "FileFormat"="%3.5f", "Output status"=w311, "ExecutionIndex"=w310, "error in (no error)"=w317) -> ("ActualVoltage (V)"=w314:dbl[], "ActualCurrent (A)"=w313:dbl[], "6240AData out"=w318:refnum<class "6240AData.lvclass">, "error out"=w316:errorcluster)  [unwired: 3 in, 3 out]
        n165 = property on="ActualVoltage (V)" class="Arr (strict)"("Val(Sgnl)"=w314) -> ()  [unwired: 2 in, 2 out]
        n166 = property on="ActualCurrent (A)" class="Arr (strict)"("Val(Sgnl)"=w313) -> ()  [unwired: 2 in, 2 out]
      }
      event "Stop Button": Value Change {
        n167 = event-data() -> ()  [unwired: 1 in, 6 out]
        n168 = local read "Initialized?"() -> (w333:bool)
        n169 = case shown="False" w333 {
          tunnel: w337 -> [w342 w354]
          tunnel: [w342 w353] -> w336
          tunnel: w335 -> [w341 w352]
          tunnel: [w341 w351] -> w334
          frame False {
          }
          frame True {
            w358 = FALSE
            n170 = local read "SetCurrent 2 (mA)"() -> (w344:dbl)
            n171 = local read "SetCurrent 1 (mA)"() -> (w348:dbl)
            n172 = Divide(x=w348, y=1000.0) -> (x/y=w346:dbl)
            n173 = Divide(x=w344, y=1000.0) -> (x/y=w343:dbl)
            n174 = Build Array(w346, w343) -> (w350:dbl[])
            n175 = Build Array(w358, w358) -> (w349:bool[])
            n176 = property on="Output\n (ADCMT)" class="Arr (strict)"("Val(Sgnl)"=w349) -> ()  [unwired: 2 in, 2 out]
            n177 = call-dynamic "6240AData_execute.vi"("6240AData in"=w354, "SetCurrent (A)"=w350, "FileFormat"="%3.5f", "Output status"=w349, "error in (no error)"=w352) -> ("ActualVoltage (V)"=w355:dbl[], "ActualCurrent (A)"=w356:dbl[], "6240AData out"=w353:refnum<class "6240AData.lvclass">, "error out"=w351:errorcluster)  [unwired: 4 in, 3 out]
            n178 = property on="ActualVoltage (V)" class="Arr (strict)"("Val(Sgnl)"=w355) -> ()  [unwired: 2 in, 2 out]
            n179 = property on="ActualCurrent (A)" class="Arr (strict)"("Val(Sgnl)"=w356) -> ()  [unwired: 2 in, 2 out]
          }
        }
        n180 = call-dynamic "6240AData_terrminate.vi"("error in (no error)"=w334, "6240AData in"=w336) -> ("error out"=w338:errorcluster, "6240AData out"=w339:refnum<class "6240AData.lvclass">)  [unwired: 8 in]
      }
    }
    "error out (ADCMT6420A)" <- w247
  }
  n181 = while {
    stop <- w367 stop-if-true
    n182 = Get Date/Time In Seconds() -> (seconds since 1Jan1904=w366:timestamp)
    n183 = Format Date/Time String(time format string (%c)="%Y%m", seconds (now)=w366) -> (date/time string=w363:string)  [unwired: 1 in]
    n184 = Build Path(base path="Base Path (screenshots)", name or relative path=w363) -> (appended path=w362:path)
    n185 = Create Folder(path (use dialog)=w362, error in=errorcluster {"status"=FALSE, "code"=0, "source"=""}) -> (created path=w359:path, error out=→"error out (monthly folder creation)":errorcluster)  [unwired: 1 in, 1 out]
    n186 = event shown="[1] \"Frontpanel screenshots\": Value Change" {
      selector: _ -> [_ _ _]
      dyn-events: _ -> [_ _ _]
      timeout: _ -> [_ _ _]
      tunnel: [FALSE _ TRUE] -> w367
      tunnel: w359 -> [_ w375 _]
      tunnel: w366 -> [_ w374 _]
      event Timeout {
        n187 = event-data() -> ()  [unwired: 1 in, 3 out]
      }
      event "Frontpanel screenshots": Value Change {
        n188 = event-data() -> ()  [unwired: 1 in, 3 out]
        n189 = property class="TabCtl (strict)"() -> ("Value"=w372:T1)  [unwired: 2 in, 2 out]
        n190 = stacked-sequence {
          tunnel: w375 -> [w381 w403 w425 w447 w469 w491 w513 w535 w557 _]
          tunnel: w374 -> [w380 w402 w424 w446 w468 w490 w512 w534 w556 _]
          tunnel: [w378 _ _ _ _ _ _ _ _ _] -> w373
          tunnel: w372 -> [w377 _ _ _ _ _ _ _ _ _]
          tunnel: [w377 _ _ _ _ _ _ _ _ _] -> w371
          tunnel: "cryostatus_" ("string") -> [w376 w399 w421 w443 w465 w487 w509 w531 w553 _]
          frame #0 {
            n191 = flat-sequence {
              tunnel: w380 -> [w383]
              tunnel: [w383] -> w379
              tunnel: w381 -> [w398]
              tunnel: w379 -> [w386]
              tunnel: [w385] -> w378
              tunnel: w376 -> [w384]
              frame #0 {
                n192 = property class="TabCtl (strict)"("Val(Sgnl)"=T1."NI USB CONFIG" ("Value (Signaling)")) -> ()  [unwired: 2 in, 2 out]
              }
              frame #1 {
                w396 = "_" ("string")
                n193 = local read "Cycle #"() -> (w394:u32)
                n194 = call "LV_UNIXTIME.vi"("current time"=w386) -> ("date/time string"=w397:string)  [unwired: 9 in, 1 out]
                n195 = Format Value(format string="%06d", value (0)=w394) -> (output string=w393:string)  [unwired: 1 in]
                n196 = Concatenate Strings(w384, w397, w396, w393, w396, "page1.png" ("string")) -> (w391:string)
                n197 = invoke class="TabCtl (strict)" method="Get Image"(error in=errorcluster {"status"=FALSE, "code"=0, "source"=""} ("error in (no error)")) -> (error out=w387:errorcluster, "image data"=w389:T24)  [unwired: 5 in, 4 out]
                n198 = Build Path(base path=w398, name or relative path=w391) -> (appended path=w390:path)
                n199 = call <vilib>:"Write PNG File.vi"("error in (no error)"=w387, "image data"=w389, "path to PNG file"=w390) -> ("error out"=w385:errorcluster)  [unwired: 7 in, 1 out]
              }
            }
          }
          frame #1 {
            n200 = flat-sequence {
              tunnel: w402 -> [w405]
              tunnel: [w405] -> w401
              tunnel: w403 -> [w420]
              tunnel: w401 -> [w408]
              tunnel: [w407] -> w400
              tunnel: w399 -> [w406]
              frame #0 {
                n201 = property class="TabCtl (strict)"("Val(Sgnl)"=T1."NI USB CONFIG" ("Value (Signaling)")) -> ()  [unwired: 2 in, 2 out]
              }
              frame #1 {
                w418 = "_" ("string")
                n202 = local read "Cycle #"() -> (w416:u32)
                n203 = call "LV_UNIXTIME.vi"("current time"=w408) -> ("date/time string"=w419:string)  [unwired: 9 in, 1 out]
                n204 = Format Value(format string="%06d", value (0)=w416) -> (output string=w415:string)  [unwired: 1 in]
                n205 = Concatenate Strings(w406, w419, w418, w415, w418, "page2.png" ("string")) -> (w413:string)
                n206 = invoke class="TabCtl (strict)" method="Get Image"(error in=errorcluster {"status"=FALSE, "code"=0, "source"=""} ("error in (no error)")) -> (error out=w409:errorcluster, "image data"=w411:T24)  [unwired: 5 in, 4 out]
                n207 = Build Path(base path=w420, name or relative path=w413) -> (appended path=w412:path)
                n208 = call <vilib>:"Write PNG File.vi"("error in (no error)"=w409, "image data"=w411, "path to PNG file"=w412) -> ("error out"=w407:errorcluster)  [unwired: 7 in, 1 out]
              }
            }
            n209 = local write "error out (frontpanel screenshots)"(w400) -> ()
          }
          frame #2 {
            n210 = flat-sequence {
              tunnel: w424 -> [w427]
              tunnel: [w427] -> w423
              tunnel: w425 -> [w442]
              tunnel: w423 -> [w430]
              tunnel: [w429] -> w422
              tunnel: w421 -> [w428]
              frame #0 {
                n211 = property class="TabCtl (strict)"("Val(Sgnl)"=T1."NI USB CONFIG" ("Value (Signaling)")) -> ()  [unwired: 2 in, 2 out]
              }
              frame #1 {
                w440 = "_" ("string")
                n212 = local read "Cycle #"() -> (w438:u32)
                n213 = Format Value(format string="%06d", value (0)=w438) -> (output string=w437:string)  [unwired: 1 in]
                n214 = call "LV_UNIXTIME.vi"("current time"=w430) -> ("date/time string"=w441:string)  [unwired: 9 in, 1 out]
                n215 = Concatenate Strings(w428, w441, w440, w437, w440, "page3.png" ("string")) -> (w435:string)
                n216 = invoke class="TabCtl (strict)" method="Get Image"(error in=errorcluster {"status"=FALSE, "code"=0, "source"=""} ("error in (no error)")) -> (error out=w431:errorcluster, "image data"=w433:T24)  [unwired: 5 in, 4 out]
                n217 = Build Path(base path=w442, name or relative path=w435) -> (appended path=w434:path)
                n218 = call <vilib>:"Write PNG File.vi"("error in (no error)"=w431, "image data"=w433, "path to PNG file"=w434) -> ("error out"=w429:errorcluster)  [unwired: 7 in, 1 out]
              }
            }
            n219 = local write "error out (frontpanel screenshots)"(w422) -> ()
          }
          frame #3 {
            n220 = flat-sequence {
              tunnel: w446 -> [w449]
              tunnel: [w449] -> w445
              tunnel: w447 -> [w464]
              tunnel: w445 -> [w452]
              tunnel: [w451] -> w444
              tunnel: w443 -> [w450]
              frame #0 {
                n221 = property class="TabCtl (strict)"("Val(Sgnl)"=T1."HE AUTO FILL" ("Value (Signaling)")) -> ()  [unwired: 2 in, 2 out]
              }
              frame #1 {
                w462 = "_" ("string")
                n222 = local read "Cycle #"() -> (w460:u32)
                n223 = Format Value(format string="%06d", value (0)=w460) -> (output string=w459:string)  [unwired: 1 in]
                n224 = call "LV_UNIXTIME.vi"("current time"=w452) -> ("date/time string"=w463:string)  [unwired: 9 in, 1 out]
                n225 = Concatenate Strings(w450, w463, w462, w459, w462, "page4.png" ("string")) -> (w457:string)
                n226 = invoke class="TabCtl (strict)" method="Get Image"(error in=errorcluster {"status"=FALSE, "code"=0, "source"=""} ("error in (no error)")) -> (error out=w453:errorcluster, "image data"=w455:T24)  [unwired: 5 in, 4 out]
                n227 = Build Path(base path=w464, name or relative path=w457) -> (appended path=w456:path)
                n228 = call <vilib>:"Write PNG File.vi"("error in (no error)"=w453, "image data"=w455, "path to PNG file"=w456) -> ("error out"=w451:errorcluster)  [unwired: 7 in, 1 out]
              }
            }
            n229 = local write "error out (frontpanel screenshots)"(w444) -> ()
          }
          frame #4 {
            n230 = flat-sequence {
              tunnel: w468 -> [w471]
              tunnel: [w471] -> w467
              tunnel: w469 -> [w486]
              tunnel: w467 -> [w474]
              tunnel: [w473] -> w466
              tunnel: w465 -> [w472]
              frame #0 {
                n231 = property class="TabCtl (strict)"("Val(Sgnl)"=T1."VALVE/HEATER CTRL" ("Value (Signaling)")) -> ()  [unwired: 2 in, 2 out]
              }
              frame #1 {
                w484 = "_" ("string")
                n232 = local read "Cycle #"() -> (w482:u32)
                n233 = call "LV_UNIXTIME.vi"("current time"=w474) -> ("date/time string"=w485:string)  [unwired: 9 in, 1 out]
                n234 = Format Value(format string="%06d", value (0)=w482) -> (output string=w481:string)  [unwired: 1 in]
                n235 = Concatenate Strings(w472, w485, w484, w481, w484, "page5.png" ("string")) -> (w479:string)
                n236 = invoke class="TabCtl (strict)" method="Get Image"(error in=errorcluster {"status"=FALSE, "code"=0, "source"=""} ("error in (no error)")) -> (error out=w475:errorcluster, "image data"=w477:T24)  [unwired: 5 in, 4 out]
                n237 = Build Path(base path=w486, name or relative path=w479) -> (appended path=w478:path)
                n238 = call <vilib>:"Write PNG File.vi"("error in (no error)"=w475, "image data"=w477, "path to PNG file"=w478) -> ("error out"=w473:errorcluster)  [unwired: 7 in, 1 out]
              }
            }
            n239 = local write "error out (frontpanel screenshots)"(w466) -> ()
          }
          frame #5 {
            n240 = flat-sequence {
              tunnel: w490 -> [w493]
              tunnel: [w493] -> w489
              tunnel: w491 -> [w508]
              tunnel: w489 -> [w496]
              tunnel: [w495] -> w488
              tunnel: w487 -> [w494]
              frame #0 {
                n241 = property class="TabCtl (strict)"("Val(Sgnl)"=T1."DMMs" ("Value (Signaling)")) -> ()  [unwired: 2 in, 2 out]
              }
              frame #1 {
                w506 = "_" ("string")
                n242 = local read "Cycle #"() -> (w504:u32)
                n243 = call "LV_UNIXTIME.vi"("current time"=w496) -> ("date/time string"=w507:string)  [unwired: 9 in, 1 out]
                n244 = Format Value(format string="%06d", value (0)=w504) -> (output string=w503:string)  [unwired: 1 in]
                n245 = Concatenate Strings(w494, w507, w506, w503, w506, "page6.png" ("string")) -> (w501:string)
                n246 = invoke class="TabCtl (strict)" method="Get Image"(error in=errorcluster {"status"=FALSE, "code"=0, "source"=""} ("error in (no error)")) -> (error out=w497:errorcluster, "image data"=w499:T24)  [unwired: 5 in, 4 out]
                n247 = Build Path(base path=w508, name or relative path=w501) -> (appended path=w500:path)
                n248 = call <vilib>:"Write PNG File.vi"("error in (no error)"=w497, "image data"=w499, "path to PNG file"=w500) -> ("error out"=w495:errorcluster)  [unwired: 7 in, 1 out]
              }
            }
            n249 = local write "error out (frontpanel screenshots)"(w488) -> ()
          }
          frame #6 {
            n250 = flat-sequence {
              tunnel: w512 -> [w515]
              tunnel: [w515] -> w511
              tunnel: w513 -> [w530]
              tunnel: w511 -> [w518]
              tunnel: [w517] -> w510
              tunnel: w509 -> [w516]
              frame #0 {
                n251 = property class="TabCtl (strict)"("Val(Sgnl)"=T1."DIAGRAM" ("Value (Signaling)")) -> ()  [unwired: 2 in, 2 out]
              }
              frame #1 {
                w528 = "_" ("string")
                n252 = local read "Cycle #"() -> (w526:u32)
                n253 = Format Value(format string="%06d", value (0)=w526) -> (output string=w525:string)  [unwired: 1 in]
                n254 = call "LV_UNIXTIME.vi"("current time"=w518) -> ("date/time string"=w529:string)  [unwired: 9 in, 1 out]
                n255 = Concatenate Strings(w516, w529, w528, w525, w528, "page7.png" ("string")) -> (w523:string)
                n256 = invoke class="TabCtl (strict)" method="Get Image"(error in=errorcluster {"status"=FALSE, "code"=0, "source"=""} ("error in (no error)")) -> (error out=w519:errorcluster, "image data"=w521:T24)  [unwired: 5 in, 4 out]
                n257 = Build Path(base path=w530, name or relative path=w523) -> (appended path=w522:path)
                n258 = call <vilib>:"Write PNG File.vi"("error in (no error)"=w519, "image data"=w521, "path to PNG file"=w522) -> ("error out"=w517:errorcluster)  [unwired: 7 in, 1 out]
              }
            }
            n259 = local write "error out (frontpanel screenshots)"(w510) -> ()
          }
          frame #7 {
            n260 = flat-sequence {
              tunnel: w534 -> [w537]
              tunnel: [w537] -> w533
              tunnel: w535 -> [w552]
              tunnel: w533 -> [w540]
              tunnel: [w539] -> w532
              tunnel: w531 -> [w538]
              frame #0 {
                n261 = property class="TabCtl (strict)"("Val(Sgnl)"=T1."CHF" ("Value (Signaling)")) -> ()  [unwired: 2 in, 2 out]
              }
              frame #1 {
                w550 = "_" ("string")
                n262 = local read "Cycle #"() -> (w548:u32)
                n263 = Format Value(format string="%06d", value (0)=w548) -> (output string=w547:string)  [unwired: 1 in]
                n264 = call "LV_UNIXTIME.vi"("current time"=w540) -> ("date/time string"=w551:string)  [unwired: 9 in, 1 out]
                n265 = Concatenate Strings(w538, w551, w550, w547, w550, "page8.png" ("string")) -> (w545:string)
                n266 = invoke class="TabCtl (strict)" method="Get Image"(error in=errorcluster {"status"=FALSE, "code"=0, "source"=""} ("error in (no error)")) -> (error out=w541:errorcluster, "image data"=w543:T24)  [unwired: 5 in, 4 out]
                n267 = Build Path(base path=w552, name or relative path=w545) -> (appended path=w544:path)
                n268 = call <vilib>:"Write PNG File.vi"("error in (no error)"=w541, "image data"=w543, "path to PNG file"=w544) -> ("error out"=w539:errorcluster)  [unwired: 7 in, 1 out]
              }
            }
            n269 = local write "error out (frontpanel screenshots)"(w532) -> ()
          }
          frame #8 {
            n270 = flat-sequence {
              tunnel: w556 -> [w559]
              tunnel: [w559] -> w555
              tunnel: w557 -> [w574]
              tunnel: w555 -> [w562]
              tunnel: [w561] -> w554
              tunnel: w553 -> [w560]
              frame #0 {
                n271 = property class="TabCtl (strict)"("Val(Sgnl)"=T1."(Plc. hld.)" ("Value (Signaling)")) -> ()  [unwired: 2 in, 2 out]
              }
              frame #1 {
                w572 = "_" ("string")
                n272 = local read "Cycle #"() -> (w570:u32)
                n273 = Format Value(format string="%06d", value (0)=w570) -> (output string=w569:string)  [unwired: 1 in]
                n274 = call "LV_UNIXTIME.vi"("current time"=w562) -> ("date/time string"=w573:string)  [unwired: 9 in, 1 out]
                n275 = Concatenate Strings(w560, w573, w572, w569, w572, "page8.png" ("string")) -> (w567:string)
                n276 = invoke class="TabCtl (strict)" method="Get Image"(error in=errorcluster {"status"=FALSE, "code"=0, "source"=""} ("error in (no error)")) -> (error out=w563:errorcluster, "image data"=w565:T24)  [unwired: 5 in, 4 out]
                n277 = Build Path(base path=w574, name or relative path=w567) -> (appended path=w566:path)
                n278 = call <vilib>:"Write PNG File.vi"("error in (no error)"=w563, "image data"=w565, "path to PNG file"=w566) -> ("error out"=w561:errorcluster)  [unwired: 7 in, 1 out]
              }
            }
            n279 = local write "error out (frontpanel screenshots)"(w554) -> ()
          }
          frame #9 {
            n280 = local write "Frontpanel screenshots"(FALSE ("Frontpanel screenshots")) -> ()
          }
        }
        "error out (frontpanel screenshots)" <- w373
        n281 = property class="TabCtl (strict)"("Val(Sgnl)"=w371) -> ()  [unwired: 2 in, 2 out]
      }
      event "Stop Button": Value Change {
        n282 = event-data() -> ()  [unwired: 1 in, 3 out]
      }
    }
    n283 = Wait (ms)(milliseconds to wait=u32 123) -> ()  [unwired: 1 out]
  }
  n284 = while {
    stop <- w581 stop-if-true
    n285 = event shown="[5] \"Plot selecter LSI218(1)     1      2     3     4\", \"Plot selecter LSI218(2)     1      2     3     4\", \"Plot selecter (USB6210)     1      2     3     4\", \"Plot selecter LSI336       1      2     3     4\", \"Plot selecter (USB6218)     1      2     3     4\", \"Plot selecter (HP34401A)     1      2     3     4\": Value Change" {
      selector: _ -> [_ _ _ _ _ _ _ _ _ _ _]
      dyn-events: _ -> [_ _ _ _ _ _ _ _ _ _ _]
      timeout: _ -> [_ _ _ _ _ _ _ _ _ _ _]
      tunnel: [_ _ _ _ _ _ _ _ _ _ TRUE] -> w581
      tunnel: [errorcluster {"status"=FALSE, "code"=0, "source"=""} ("error out") w585 _ _ _ _ w721 w738 w755 w772 errorcluster {"status"=FALSE, "code"=0, "source"=""} ("error out")] -> w577
      event Timeout {
        n286 = event-data() -> ()  [unwired: 1 in, 3 out]
      }
      event "log/linear 1": Value Change {
        n287 = event-data() -> ()  [unwired: 1 in, 6 out]
        n288 = flat-sequence {
          tunnel: [w586] -> w585
          frame #0 {
            n289 = Boolean To (0,1)(Boolean="log/linear 1") -> (0, 1=w591:i16)
            n290 = control-ref of="Graph 1"() -> (w587:refnum<vi>)
            n291 = property class="XYGraph (strict)"(reference=w587, error in=errorcluster {"status"=FALSE, "code"=0, "source"=""} ("error in (no error)"), "YScale.Mapping Mode"=w591) -> (error out=w589:errorcluster)  [unwired: 1 out]
            n292 = control-ref of="error out (USB6210)"() -> (w590:refnum<vi>)
            n293 = property class="Clust (strict)"(reference=w590, "Val(Sgnl)"=w589) -> (error out=w586:errorcluster)  [unwired: 1 in, 1 out]
          }
        }
      }
      event "log/linear 2": Value Change {
        n294 = event-data() -> ()  [unwired: 1 in, 6 out]
        n295 = flat-sequence {
          frame #0 {
            n296 = Boolean To (0,1)(Boolean="log/linear 2") -> (0, 1=w597:i16)
            n297 = control-ref of="Graph 2"() -> (w595:refnum<vi>)
            n298 = property class="XYGraph (strict)"(reference=w595, error in=errorcluster {"status"=FALSE, "code"=0, "source"=""} ("error in (no error)"), "YScale.Mapping Mode"=w597) -> (error out=w596:errorcluster)  [unwired: 1 out]
            n299 = control-ref of="error out (USB6210)"() -> (w594:refnum<vi>)
            n300 = property class="Clust (strict)"(reference=w594, "Value"=w596) -> ()  [unwired: 1 in, 2 out]
          }
        }
      }
      event "log/linear 3": Value Change {
        n301 = event-data() -> ()  [unwired: 1 in, 6 out]
        n302 = flat-sequence {
          frame #0 {
            n303 = Boolean To (0,1)(Boolean="log/linear 3") -> (0, 1=w603:i16)
            n304 = control-ref of="Graph 3"() -> (w599:refnum<vi>)
            n305 = property class="XYGraph (strict)"(reference=w599, error in=errorcluster {"status"=FALSE, "code"=0, "source"=""} ("error in (no error)"), "YScale.Mapping Mode"=w603) -> (error out=w602:errorcluster)  [unwired: 1 out]
            n306 = control-ref of="error out (USB6210)"() -> (w601:refnum<vi>)
            n307 = property class="Clust (strict)"(reference=w601, "Value"=w602) -> ()  [unwired: 1 in, 2 out]
          }
        }
      }
      event "log/linear 4": Value Change {
        n308 = event-data() -> ()  [unwired: 1 in, 6 out]
        n309 = flat-sequence {
          frame #0 {
            n310 = Boolean To (0,1)(Boolean="log/linear 4") -> (0, 1=w609:i16)
            n311 = control-ref of="Graph 4"() -> (w605:refnum<vi>)
            n312 = property class="XYGraph (strict)"(reference=w605, error in=errorcluster {"status"=FALSE, "code"=0, "source"=""} ("error in (no error)"), "YScale.Mapping Mode"=w609) -> (error out=w608:errorcluster)  [unwired: 1 out]
            n313 = control-ref of="error out (USB6210)"() -> (w607:refnum<vi>)
            n314 = property class="Clust (strict)"(reference=w607, "Value"=w608) -> ()  [unwired: 1 in, 2 out]
          }
        }
      }
      event "Plot selecter LSI218(1)\n    1      2     3     4", "Plot selecter LSI218(2)\n    1      2     3     4", "Plot selecter (USB6210)\n    1      2     3     4", "Plot selecter LSI336 \n     1      2     3     4", "Plot selecter (USB6218)\n    1      2     3     4", "Plot selecter (HP34401A)\n    1      2     3     4": Value Change {
        n315 = event-data() -> ()  [unwired: 1 in, 6 out]
        n316 = local read "Labels (HP34401 LM)"() -> (w616:string[])
        n317 = call "BuildPlotLegends.vi"("Plot selecter \n    1      2     3     4"="Plot selecter (HP34401A)\n    1      2     3     4", "AllLabels"=w616) -> ("Series 4"=w611:string[], "Series 3"=w612:string[], "Series 2"=w613:string[], "Series 1"=w614:string[])  [unwired: 6 in]
        n318 = local read "All Labels (USB6210)"() -> (w633:string[])
        n319 = local read "All Labels (USB6218)"() -> (w622:string[])
        n320 = local read "Labels LSI218 (1)"() -> (w635:string[])
        n321 = local read "Labels LSI218 (2)"() -> (w636:string[])
        n322 = local read "Labels LSI336"() -> (w628:string[])
        n323 = call "BuildPlotLegends_LSI218.vi"("Plot selecter (2)\n    1      2     3     5"="Plot selecter LSI218(2)\n    1      2     3     4", "Plot selecter (1)\n    1      2     3     4"="Plot selecter LSI218(1)\n    1      2     3     4", "Labels (2)"=w636, "Labels (1)"=w635) -> ("Series 4"=w646:string[], "Series 3"=w644:string[], "Series 2"=w642:string[], "Series 1"=w640:string[])  [unwired: 4 in]
        n324 = call "BuildPlotLegends.vi"("Plot selecter \n    1      2     3     4"="Plot selecter (USB6210)\n    1      2     3     4", "AllLabels"=w633) -> ("Series 4"=w645:string[], "Series 3"=w643:string[], "Series 2"=w641:string[], "Series 1"=w639:string[])  [unwired: 6 in]
        n325 = call "BuildPlotLegends.vi"("Plot selecter \n    1      2     3     4"="Plot selecter LSI336 \n     1      2     3     4", "AllLabels"=w628) -> ("Series 4"=w623:string[], "Series 3"=w624:string[], "Series 2"=w625:string[], "Series 1"=w626:string[])  [unwired: 6 in]
        n326 = call "BuildPlotLegends.vi"("Plot selecter \n    1      2     3     4"="Plot selecter (USB6218)\n    1      2     3     4", "AllLabels"=w622) -> ("Series 4"=w618:string[], "Series 3"=w617:string[], "Series 2"=w619:string[], "Series 1"=w620:string[])  [unwired: 6 in]
        n327 = Build Array (concatenate)(w641, w642, w625, w619, w613) -> (w630:string[])
        "Series 2" <- w630
        n328 = Build Array (concatenate)(w643, w644, w624, w617, w612) -> (w631:string[])
        "Series 3" <- w631
        n329 = Build Array (concatenate)(w645, w646, w623, w618, w611) -> (w632:string[])
        "Series 4" <- w632
        n330 = Build Array (concatenate)(w639, w640, w626, w620, w614) -> (w629:string[])
        "Series 1" <- w629
        n331 = stacked-sequence {
          tunnel: [w656 _ _ _] -> w650
          tunnel: [_ w674 _ _] -> w651
          tunnel: [_ _ w691 _] -> w649
          tunnel: [_ _ _ w708] -> w648
          tunnel: w629 -> [w654 _ _ _]
          tunnel: w630 -> [_ w672 _ _]
          tunnel: w631 -> [_ _ w689 _]
          tunnel: w632 -> [_ _ _ w706]
          frame #0 {
            n332 = Array Size(array=w654) -> (size(s)=w658:i32)
            n333 = control-ref of="Graph 1"() -> (w652:refnum<vi>)
            n334 = property class="XYGraph (strict)"(reference=w652) -> ("LegNumRows"=w653:u32)  [unwired: 1 in, 2 out]
            n335 = for {
              N: w653 -> [_]
              tunnel: w652 -> [w667]
              shift-right: [w665] -> w657
              shift-left: errorcluster {"status"=FALSE, "code"=0, "source"=""} ("error in (no error)") -> [w666]
              i -> [w669]
              n336 = property class="XYGraph (strict)"(reference=w667, error in=w666, "Active Plot"=w669, "Plot.Plot Name"="") -> (error out=w665:errorcluster)  [unwired: 1 out]
            }
            n337 = for {
              N: w658 -> [_]
              tunnel: w652 -> [w663]
              shift-right: [w661] -> w656
              shift-left: w657 -> [w662]
              tunnel: w654 -> [w660] mode=indexing
              i -> [w664]
              n338 = property class="XYGraph (strict)"(reference=w663, error in=w662, "Active Plot"=w664, "Plot.Plot Name"=w660, "Plot.Visible?"=TRUE ("Plot.Visible")) -> (error out=w661:errorcluster)  [unwired: 1 out]
            }
          }
          frame #1 {
            n339 = Array Size(array=w672) -> (size(s)=w676:i32)
            n340 = control-ref of="Graph 2"() -> (w671:refnum<vi>)
            n341 = property class="XYGraph (strict)"(reference=w671) -> ("LegNumRows"=w670:u32)  [unwired: 1 in, 2 out]
            n342 = for {
              N: w670 -> [_]
              shift-right: [w683] -> w675
              shift-left: errorcluster {"status"=FALSE, "code"=0, "source"=""} ("error in (no error)") -> [w684]
              tunnel: w671 -> [w682]
              i -> [w686]
              n343 = property class="XYGraph (strict)"(reference=w682, error in=w684, "Active Plot"=w686, "Plot.Plot Name"="") -> (error out=w683:errorcluster)  [unwired: 1 out]
            }
            n344 = for {
              N: w676 -> [_]
              shift-right: [w679] -> w674
              shift-left: w675 -> [w680]
              tunnel: w672 -> [w678] mode=indexing
              tunnel: w671 -> [w677]
              i -> [w681]
              n345 = property class="XYGraph (strict)"(reference=w677, error in=w680, "Active Plot"=w681, "Plot.Plot Name"=w678) -> (error out=w679:errorcluster)  [unwired: 1 out]
            }
          }
          frame #2 {
            n346 = Array Size(array=w689) -> (size(s)=w693:i32)
            n347 = control-ref of="Graph 3"() -> (w687:refnum<vi>)
            n348 = property class="XYGraph (strict)"(reference=w687) -> ("LegNumRows"=w688:u32)  [unwired: 1 in, 2 out]
            n349 = for {
              N: w688 -> [_]
              tunnel: w687 -> [w701]
              shift-right: [w699] -> w692
              shift-left: errorcluster {"status"=FALSE, "code"=0, "source"=""} ("error in (no error)") -> [w700]
              i -> [w703]
              n350 = property class="XYGraph (strict)"(reference=w701, error in=w700, "Active Plot"=w703, "Plot.Plot Name"="") -> (error out=w699:errorcluster)  [unwired: 1 out]
            }
            n351 = for {
              N: w693 -> [_]
              tunnel: w687 -> [w697]
              shift-right: [w695] -> w691
              shift-left: w692 -> [w696]
              tunnel: w689 -> [w694] mode=indexing
              i -> [w698]
              n352 = property class="XYGraph (strict)"(reference=w697, error in=w696, "Active Plot"=w698, "Plot.Plot Name"=w694) -> (error out=w695:errorcluster)  [unwired: 1 out]
            }
          }
          frame #3 {
            n353 = Array Size(array=w706) -> (size(s)=w710:i32)
            n354 = control-ref of="Graph 4"() -> (w704:refnum<vi>)
            n355 = property class="XYGraph (strict)"(reference=w704) -> ("LegNumRows"=w705:u32)  [unwired: 1 in, 2 out]
            n356 = for {
              N: w705 -> [_]
              tunnel: w704 -> [w718]
              shift-right: [w716] -> w709
              shift-left: errorcluster {"status"=FALSE, "code"=0, "source"=""} ("error in (no error)") -> [w717]
              i -> [w720]
              n357 = property class="XYGraph (strict)"(reference=w718, error in=w717, "Active Plot"=w720, "Plot.Plot Name"="") -> (error out=w716:errorcluster)  [unwired: 1 out]
            }
            n358 = for {
              N: w710 -> [_]
              tunnel: w704 -> [w714]
              shift-right: [w712] -> w708
              shift-left: w709 -> [w713]
              tunnel: w706 -> [w711] mode=indexing
              i -> [w715]
              n359 = property class="XYGraph (strict)"(reference=w714, error in=w713, "Active Plot"=w715, "Plot.Plot Name"=w711) -> (error out=w712:errorcluster)  [unwired: 1 out]
            }
          }
        }
        n360 = Merge Errors(w650, w651, w649, w648) -> (→"Plot errors":errorcluster)
      }
      event "Take Screenshot! 1": Value Change {
        n361 = event-data() -> ()  [unwired: 1 in, 6 out]
        n362 = flat-sequence {
          tunnel: [w722] -> w721
          frame #0 {
            n363 = flat-sequence {
              tunnel: [w723] -> w722
              frame #0 {
                w732 = "_" ("string")
                n364 = Get Date/Time In Seconds() -> (seconds since 1Jan1904=w729:timestamp)
                n365 = local read "RUN Identifier"() -> (w734:string)
                n366 = call "LV_UNIXTIME.vi"("current time"=w729) -> ("date/time string"=w733:string)  [unwired: 9 in, 1 out]
                n367 = control-ref of="Graph 1"() -> (w728:refnum<vi>)
                n368 = Concatenate Strings(w734, w732, w733, w732, "FIle suffix 1", ".png" ("string")) -> (w736:string)
                n369 = local read "Base Path"() -> (w735:path)
                n370 = invoke class="XYGraph (strict)" method="Get Image"(reference=w728, error in=errorcluster {"status"=FALSE, "code"=0, "source"=""} ("error in (no error)")) -> (error out=w724:errorcluster, "image data"=w727:T24)  [unwired: 4 in, 4 out]
                n371 = Build Path(base path=w735, name or relative path=w736) -> (appended path=w726:path)
                n372 = call <vilib>:"Write PNG File.vi"("error in (no error)"=w724, "image data"=w727, "path to PNG file"=w726) -> ("error out"=w723:errorcluster)  [unwired: 7 in, 1 out]
              }
              frame #1 {
                n373 = local write "Take Screenshot! 1"(FALSE ("Take Screenshot! 1")) -> ()
              }
            }
          }
        }
      }
      event "Take Screenshot! 2": Value Change {
        n374 = event-data() -> ()  [unwired: 1 in, 6 out]
        n375 = flat-sequence {
          tunnel: [w739] -> w738
          frame #0 {
            n376 = flat-sequence {
              tunnel: [w745] -> w739
              frame #0 {
                w749 = "_" ("string")
                n377 = Get Date/Time In Seconds() -> (seconds since 1Jan1904=w746:timestamp)
                n378 = local read "RUN Identifier"() -> (w751:string)
                n379 = call "LV_UNIXTIME.vi"("current time"=w746) -> ("date/time string"=w750:string)  [unwired: 9 in, 1 out]
                n380 = control-ref of="Graph 2"() -> (w740:refnum<vi>)
                n381 = Concatenate Strings(w751, w749, w750, w749, "FIle suffix 2", ".png" ("string")) -> (w753:string)
                n382 = local read "Base Path"() -> (w752:path)
                n383 = invoke class="XYGraph (strict)" method="Get Image"(reference=w740, error in=errorcluster {"status"=FALSE, "code"=0, "source"=""} ("error in (no error)")) -> (error out=w744:errorcluster, "image data"=w742:T24)  [unwired: 4 in, 4 out]
                n384 = Build Path(base path=w752, name or relative path=w753) -> (appended path=w741:path)
                n385 = call <vilib>:"Write PNG File.vi"("error in (no error)"=w744, "image data"=w742, "path to PNG file"=w741) -> ("error out"=w745:errorcluster)  [unwired: 7 in, 1 out]
              }
              frame #1 {
                n386 = local write "Take Screenshot! 2"(FALSE ("Take Screenshot! 1")) -> ()
              }
            }
          }
        }
      }
      event "Take Screenshot! 3": Value Change {
        n387 = event-data() -> ()  [unwired: 1 in, 6 out]
        n388 = flat-sequence {
          tunnel: [w756] -> w755
          frame #0 {
            n389 = flat-sequence {
              tunnel: [w758] -> w756
              frame #0 {
                w766 = "_" ("string")
                n390 = Get Date/Time In Seconds() -> (seconds since 1Jan1904=w764:timestamp)
                n391 = local read "RUN Identifier"() -> (w768:string)
                n392 = call "LV_UNIXTIME.vi"("current time"=w764) -> ("date/time string"=w767:string)  [unwired: 9 in, 1 out]
                n393 = control-ref of="Graph 3"() -> (w761:refnum<vi>)
                n394 = Concatenate Strings(w768, w766, w767, w766, "FIle suffix 3", ".png" ("string")) -> (w770:string)
                n395 = local read "Base Path"() -> (w769:path)
                n396 = invoke class="XYGraph (strict)" method="Get Image"(reference=w761, error in=errorcluster {"status"=FALSE, "code"=0, "source"=""} ("error in (no error)")) -> (error out=w759:errorcluster, "image data"=w757:T24)  [unwired: 4 in, 4 out]
                n397 = Build Path(base path=w769, name or relative path=w770) -> (appended path=w762:path)
                n398 = call <vilib>:"Write PNG File.vi"("error in (no error)"=w759, "image data"=w757, "path to PNG file"=w762) -> ("error out"=w758:errorcluster)  [unwired: 7 in, 1 out]
              }
              frame #1 {
                n399 = local write "Take Screenshot! 3"(FALSE ("Take Screenshot! 1")) -> ()
              }
            }
          }
        }
      }
      event "Take Screenshot! 4": Value Change {
        n400 = event-data() -> ()  [unwired: 1 in, 6 out]
        n401 = flat-sequence {
          tunnel: [w773] -> w772
          frame #0 {
            n402 = flat-sequence {
              tunnel: [w776] -> w773
              frame #0 {
                w783 = "_" ("string")
                n403 = Get Date/Time In Seconds() -> (seconds since 1Jan1904=w781:timestamp)
                n404 = local read "RUN Identifier"() -> (w785:string)
                n405 = call "LV_UNIXTIME.vi"("current time"=w781) -> ("date/time string"=w784:string)  [unwired: 9 in, 1 out]
                n406 = control-ref of="Graph 4"() -> (w777:refnum<vi>)
                n407 = Concatenate Strings(w785, w783, w784, w783, "FIle suffix 4", ".png" ("string")) -> (w787:string)
                n408 = local read "Base Path"() -> (w786:path)
                n409 = invoke class="XYGraph (strict)" method="Get Image"(reference=w777, error in=errorcluster {"status"=FALSE, "code"=0, "source"=""} ("error in (no error)")) -> (error out=w774:errorcluster, "image data"=w778:T24)  [unwired: 4 in, 4 out]
                n410 = Build Path(base path=w786, name or relative path=w787) -> (appended path=w779:path)
                n411 = call <vilib>:"Write PNG File.vi"("error in (no error)"=w774, "image data"=w778, "path to PNG file"=w779) -> ("error out"=w776:errorcluster)  [unwired: 7 in, 1 out]
              }
              frame #1 {
                n412 = local write "Take Screenshot! 4"(FALSE ("Take Screenshot! 1")) -> ()
              }
            }
          }
        }
      }
      event "Stop Button": Value Change {
        n413 = event-data() -> ()  [unwired: 1 in, 6 out]
      }
    }
    "error out (graph operations)" <- w577
    n414 = local write "Take Screenshot! 1"(FALSE ("Take Screenshot! 1")) -> ()
    n415 = local write "Take Screenshot! 2"(FALSE ("Take Screenshot! 1")) -> ()
    n416 = Wait (ms)(milliseconds to wait=u32 1000) -> ()  [unwired: 1 out]
    n417 = local write "Take Screenshot! 3"(FALSE ("Take Screenshot! 1")) -> ()
    n418 = local write "Take Screenshot! 4"(FALSE ("Take Screenshot! 1")) -> ()
  }
  n419 = while {
    i -> [w795]
    stop <- w792 stop-if-true
    n420 = Equal?(x=w795, y=0) -> (x = y?=w793:bool)
    n421 = case shown="True" w793 {
      frame False {
      }
      frame True {
        n422 = property on="Agilent\nIntialized?" class="Bool (strict)"("Val(Sgnl)"=FALSE ("Value (Signaling)")) -> ()  [unwired: 2 in, 2 out]
      }
    }
    n423 = Wait (ms)(milliseconds to wait=u32 123) -> ()  [unwired: 1 out]
    n424 = event shown="[3] \"OUTPUT  Kenwood\", \"Kenwood set V (V)\": Value Change" {
      selector: _ -> [_ _ _ _ _]
      dyn-events: _ -> [_ _ _ _ _]
      timeout: _ -> [_ _ _ _ _]
      tunnel: [FALSE ("Value (Signaling)") TRUE ("Value (Signaling)") _ _ _] -> w792
      tunnel: "VISA (Agilent 34402)" -> [_ _ w801 w804 _]
      event Timeout {
        n425 = event-data() -> ()  [unwired: 1 in, 3 out]
      }
      event "Stop Button": Value Change {
        n426 = event-data() -> ()  [unwired: 1 in, 3 out]
      }
      event "Initialize (Agilent)": Value Change {
        n427 = event-data() -> ()  [unwired: 1 in, 3 out]
        n428 = property on="Agilent\nIntialized?" class="Bool (strict)"("Val(Sgnl)"=TRUE ("Value (Signaling)")) -> ()  [unwired: 2 in, 2 out]
        n429 = call "Initialize.vi"("error in (no error)"=errorcluster {"status"=FALSE, "code"=0, "source"=""}, "VISA resource name"=w801) -> ("error out"=→"error out (Agilent)":errorcluster)  [unwired: 8 in, 1 out]
      }
      event "OUTPUT \nKenwood", "Kenwood set V (V)": Value Change {
        n430 = local read "Agilent\nIntialized?"() -> (w803:bool)
        n431 = event-data() -> ()  [unwired: 1 in, 3 out]
        n432 = case shown="True" w803 {
          tunnel: w804 -> [_ w810]
          frame False {
          }
          frame True {
            w812 = u16 0 items=["DC", "Sine", "Square", "Triangle", "Ramp", "Pulse", "Noise", "Sinc", "Negative Ramp", "Exponential Rise", "Exponential Fall", "Cardiac"] ("Waveform Function (1: Sine)")
            n433 = xnode "Formula"("X1"="Kenwood set V (V)") -> ("Result"=w805:dbl)  [unwired: 1 in, 1 out]
            n434 = call "Configure Standard Waveform.vi"("DC Offset (0.00 V)"=w805, "Frequency (1000 Hz)"=1.0, "error in (no error)"=errorcluster {"status"=FALSE, "code"=0, "source"=""}, "Amplitude (1)"=1.0, "Waveform Function (1: Sine)"=w812, "VISA resource name"=w810) -> ("error out"=w814:errorcluster, "VISA resource name out"=w815:refnum<visa-resource-name>)  [unwired: 4 in]
            n435 = call "Enable Output.vi"("error in (no error)"=w814, "Enable Output  (T: Enable)"="OUTPUT \nKenwood", "VISA resource name"=w815) -> ("error out"=w808:errorcluster)  [unwired: 7 in, 1 out]
            n436 = local write "error out (Agilent)"(w808) -> ()
          }
        }
      }
      event "V_lim_up (V)", "V_lim_low (V)": Value Change {
        n437 = event-data() -> ()  [unwired: 1 in, 3 out]
        n438 = property on="Kenwood set V (V)" class="DigNum (strict)"("Minimum"="V_lim_low (V)", "Maximum"="V_lim_up (V)") -> ()  [unwired: 2 in, 2 out]
      }
    }
  }
  n439 = while {
    stop <- w827 stop-if-true
    n440 = Wait (ms)(milliseconds to wait=u32 101) -> ()  [unwired: 1 out]
    n441 = event shown="[2] Timeout" {
      selector: _ -> [_ _ _]
      dyn-events: _ -> [_ _ _]
      timeout: _ -> [_ _ _]
      tunnel: [FALSE TRUE FALSE] -> w827
      event "Initialize (DMMs)": Value Change {
        w830 = T4 [] ("Value (Signaling)")
        n442 = event-data() -> ()  [unwired: 1 in, 3 out]
        n443 = property on="Graph DMMs 1" class="XYGraph (strict)"("Val(Sgnl)"=w830) -> ()  [unwired: 2 in, 2 out]
        n444 = property on="Graph DMMs 2" class="XYGraph (strict)"("Val(Sgnl)"=w830) -> ()  [unwired: 2 in, 2 out]
      }
      event "Stop Button": Value Change {
        n445 = event-data() -> ()  [unwired: 1 in, 3 out]
      }
      event Timeout {
        n446 = event-data() -> ()  [unwired: 1 in, 3 out]
      }
    }
  }
  n447 = Obtain Notifier(name (unnamed)="stop notifier", notification data type=w17, create if not found? (T)=w17, error in (no error)=errorcluster {"status"=FALSE, "code"=0, "source"=""}) -> (notifier out=w5:refnum<notifier>, error out=w4:errorcluster)  [unwired: 1 out]
  n448 = while {
    shift-right: [w943] -> w40
    shift-left: refnum<class "USBData.lvclass"> refnum ("USBData.lvclass") -> [w946]
    shift-right: [w939] -> w39
    shift-left: w6 -> [w945]
    tunnel: "Base Path" -> [w845]
    shift-right: [w921] -> w34
    shift-left: errorcluster {"status"=FALSE, "code"=0, "source"=""} ("error in (no error)") -> [w937]
    shift-right: [w922] -> w35
    shift-left: refnum<class "LSI218Data.lvclass"> refnum ("LSI218Data.lvclass") -> [w936]
    shift-right: [w909] -> w31
    shift-left: refnum<class "LSI336Data.lvclass"> refnum ("LSI336Data.lvclass") -> [w918]
    shift-right: [w908] -> w30
    shift-left: w21 -> [w917]
    shift-right: [w897] -> _
    shift-left: w6 -> [w898]
    shift-right: [w887] -> w25
    shift-left: refnum<class "USBData.lvclass"> refnum ("USBData.lvclass") -> [w895]
    shift-right: [w886] -> w24
    shift-left: errorcluster {"status"=FALSE, "code"=0, "source"=""} ("error in (no error)") -> [w894]
    shift-right: [w883] -> _
    shift-left: w21 -> [w882]
    tunnel: w5 -> [w853]
    tunnel: w4 -> [w852]
    tunnel: [w850] -> w13
    tunnel: [w849] -> w12
    shift-right: [w846] -> _
    shift-left: refnum<class "LMData.lvclass"> refnum ("LMData in") -> [w847]
    shift-right: [w843] -> _
    shift-left: errorcluster {"status"=FALSE, "code"=0, "source"=""} ("error in (no error)") -> [w844]
    i -> [w842]
    stop <- "Stop Button" stop-if-true
    w838 = T26 [] ("appended array")
    w904 = u32 24 ("Number of Rows")
    w914 = T26 [] ("appended array")
    w931 = T26 [] ("appended array")
    n449 = local read "LSI218Settings(A-F)"() -> (w874:T3)
    n450 = control-ref of="Plot selecter LSI218(2)\n    1      2     3     4"() -> (w902:refnum<vi>)
    n451 = control-ref of="Plot selecter LSI218(1)\n    1      2     3     4"() -> (w903:refnum<vi>)
    n452 = control-ref of="Plot selecter LSI336 \n     1      2     3     4"() -> (w901:refnum<vi>)
    n453 = property on="Property Node" class="Arr (strict)"(reference=w902, "Number of Rows"=w904) -> ()  [unwired: 1 in, 2 out]
    n454 = property on="Property Node" class="Arr (strict)"(reference=w903, "Number of Rows"=w904) -> ()  [unwired: 1 in, 2 out]
    n455 = local read "LSI336Settings(X,Y)"() -> (w872:T3)
    n456 = Array Size(array=w874) -> (size(s)=w873:i32)
    n457 = property on="Property Node" class="Arr (strict)"(reference=w901, "Number of Rows"=u32 8) -> ()  [unwired: 1 in, 2 out]
    n458 = Multiply(x="Measurement Interval (s)", y=u32 1000) -> (x*y=w940:dbl)
    n459 = Wait (ms)(milliseconds to wait=w940) -> ()  [unwired: 1 out]
    n460 = for {
      N: w873 -> [_]
      tunnel: w874 -> [w1034] mode=indexing
      tunnel: [w1033] -> w870 mode=concatenating
      n461 = Unbundle By Name(w1034) -> ("SensorLocations"=w1033:T19)
    }
    n462 = for {
      tunnel: w872 -> [w1032] mode=indexing
      tunnel: [w1031] -> w871 mode=concatenating
      n463 = Unbundle By Name(w1032) -> ("SensorLocations"=w1031:T19)
    }
    n464 = Quotient & Remainder(x=w842, y="Screenshots interval") -> (x-y*floor(x/y)=w858:i64)  [unwired: 1 out]
    n465 = Equal?(x=w842, y=0) -> (x = y?=w848:bool)
    n466 = case shown="True" w848 {
      tunnel: w946 -> [w2099 w2122]
      tunnel: w945 -> [w2093 w2120]
      tunnel: w842 -> [w2084 _]
      tunnel: [w2091 w2117] -> w939
      tunnel: [w2088 w2116] -> w896
      tunnel: [w2089 w2115] -> w943
      tunnel: [w2079 w2110] -> w944
      tunnel: w845 -> [_ w2109]
      tunnel: [w2078 w2106] -> w879
      frame False {
        n467 = call-dynamic "USBData_measure.vi"("USBData in"=w2099, "DAQ sample #"=i64 5, "DAQ timeout"=100.0 ("DAQ timeout (def: 100)"), "MeasurementIndex"=w2084, "error in (no error)"=w2093, "save every ... measurements"="Record interval") -> ("USBData out"=w2098:refnum<class "USBData.lvclass">, "TimeMeasuremeent"=w2095:timestamp, "Status"=→"USB6210 Status":T6, "LastDataAcquired"=w2080:dbl[], "error out"=w2094:errorcluster)  [unwired: 3 in, 2 out]
        "Time of Last Measurement (USB6210)" <- w2095
        "Last Vol\n(USB6210)" <- w2080
        n468 = call-dynamic "USBData_convert.vi"("Save every ... measurements"="Record interval", "MeasurementIndex"=w2084, "error in (no error)"=w2094, "LastDataAcquired"=w2080, "TimeMeasuremeent"=w2095, "USBData in"=w2098) -> ("error out"=w2092:errorcluster, "LeakDet_FULL"=w2087:dbl, "LastDataConverted"=w2081:dbl[], "USBData out"=w2090:refnum<class "USBData.lvclass">)  [unwired: 2 in]
        n469 = call "USBData_read.vi"("USBData in"=w2090, "error in (no error)"=w2092) -> ("Status"=w2082:T6, "USBData out"=w2089:refnum<class "USBData.lvclass">, "Data"=w2088:T27, "Basic"=w2079:T28, "error out"=w2091:errorcluster)  [unwired: 2 in, 2 out]
        n470 = local write "USB6210 Status"(w2082) -> ()
        n471 = Unbundle By Name(w2079) -> ("ReadLeakDet?"=w2086:bool)
        n472 = Unbundle By Name(w2079) -> ("Labels"=w2078:string[])
        n473 = case shown="False" w2086 {
          tunnel: w2081 -> [w2100 w2103]
          tunnel: w2087 -> [_ w2102]
          tunnel: [w2100 w2101] -> w2085
          frame False {
          }
          frame True {
            n474 = Build Array (concatenate)(w2103, w2102) -> (w2101:dbl[])
          }
        }
        "Last Data \n(USB6210)" <- w2085
      }
      frame True {
        n475 = local read "RUN Identifier"() -> (w2104:string)
        n476 = call-dynamic "USBData_initialize.vi"("USBData in"=w2122, "SeriesSetting"="USB6210 Config", "BasePath"=w2109, "RunIdentifier"=w2104, "FileName"="InstName (USB6210)", "error in (no error)"=w2120) -> ("Status"=w2105:T6, "USBData out"=w2118:refnum<class "USBData.lvclass">, "error out"=w2119:errorcluster)  [unwired: 5 in, 2 out]
        n477 = local write "USB6210 Status"(w2105) -> ()
        n478 = call "USBData_read.vi"("USBData in"=w2118, "error in (no error)"=w2119) -> ("Status"=w2108:T6, "USBData out"=w2115:refnum<class "USBData.lvclass">, "Data"=w2116:T27, "Basic"=w2110:T28, "error out"=w2117:errorcluster)  [unwired: 2 in, 2 out]
        n479 = local write "USB6210 Status"(w2108) -> ()
        n480 = Unbundle By Name(w2110) -> ("ReadLeakDet?"=w2114:bool, "Labels"=w2106:string[])
        n481 = Array Size(array=w2106) -> (size(s)=w2113:i32)
        n482 = case shown="True" w2114 {
          tunnel: w2113 -> [w2123 w2125]
          tunnel: [w2123 w2124] -> w2111
          frame False {
          }
          frame True {
            n483 = Add(x=w2125, y=1) -> (x+y=w2124:i32)
          }
        }
        n484 = Initialize Array(TRUE ("Activate 2"), w2111) -> ()  [unwired: 1 out]
      }
    }
    "error out (USB6210)" <- w939
    n485 = case shown="False" w848 {
      tunnel: [w1615 w1642] -> w886
      tunnel: [w1612 w1641] -> w893
      tunnel: [w1613 w1640] -> w887
      tunnel: [w1604 w1635] -> w892
      tunnel: [w1603 w1633] -> _
      tunnel: w895 -> [w1602 w1631]
      tunnel: w845 -> [_ w1630]
      tunnel: w894 -> [w1601 w1629]
      tunnel: w842 -> [w1600 _]
      frame False {
        n486 = local read "Record interval"() -> (w1599:i64)
        n487 = call-dynamic "USBData_measure.vi"("USBData in"=w1602, "DAQ sample #"=i64 5, "DAQ timeout"=100.0 ("DAQ timeout (def: 100)"), "MeasurementIndex"=w1600, "error in (no error)"=w1601, "save every ... measurements"=w1599) -> ("USBData out"=w1621:refnum<class "USBData.lvclass">, "TimeMeasuremeent"=w1618:timestamp, "Status"=→"USB6218 Status":T6, "LastDataAcquired"=w1605:dbl[], "error out"=w1617:errorcluster)  [unwired: 3 in, 2 out]
        "Time of Last Measurement (USB6218)" <- w1618
        "Last Vol \n(USB6218)" <- w1605
        n488 = call-dynamic "USBData_convert.vi"("Save every ... measurements"=w1599, "MeasurementIndex"=w1600, "error in (no error)"=w1617, "LastDataAcquired"=w1605, "TimeMeasuremeent"=w1618, "USBData in"=w1621) -> ("error out"=w1616:errorcluster, "LeakDet_FULL"=w1611:dbl, "LastDataConverted"=w1606:dbl[], "USBData out"=w1614:refnum<class "USBData.lvclass">)  [unwired: 2 in]
        n489 = call "USBData_read.vi"("USBData in"=w1614, "error in (no error)"=w1616) -> ("Status"=w1607:T6, "USBData out"=w1613:refnum<class "USBData.lvclass">, "Data"=w1612:T27, "Basic"=w1604:T28, "error out"=w1615:errorcluster)  [unwired: 2 in, 2 out]
        n490 = local write "USB6218 Status"(w1607) -> ()
        n491 = Unbundle By Name(w1604) -> ("ReadLeakDet?"=w1610:bool)
        n492 = Unbundle By Name(w1604) -> ("Labels"=w1603:string[])
        n493 = case shown="True" w1610 {
          tunnel: w1606 -> [w1622 w1625]
          tunnel: w1611 -> [_ w1624]
          tunnel: [w1622 w1623] -> w1609
          frame False {
          }
          frame True {
            n494 = Build Array (concatenate)(w1625, w1624) -> (w1623:dbl[])
          }
        }
        "Last Data \n(USB6218)" <- w1609
      }
      frame True {
        n495 = local read "RUN Identifier"() -> (w1626:string)
        n496 = call-dynamic "USBData_initialize.vi"("USBData in"=w1631, "SeriesSetting"="USB6218 Config", "BasePath"=w1630, "RunIdentifier"=w1626, "FileName"="InstName (USB6218)", "error in (no error)"=w1629) -> ("Status"=w1627:T6, "USBData out"=w1643:refnum<class "USBData.lvclass">, "error out"=w1644:errorcluster)  [unwired: 5 in, 2 out]
        n497 = local write "USB6218 Status"(w1627) -> ()
        n498 = call "USBData_read.vi"("USBData in"=w1643, "error in (no error)"=w1644) -> ("Status"=w1634:T6, "USBData out"=w1640:refnum<class "USBData.lvclass">, "Data"=w1641:T27, "Basic"=w1635:T28, "error out"=w1642:errorcluster)  [unwired: 2 in, 2 out]
        n499 = local write "USB6218 Status"(w1634) -> ()
        n500 = Unbundle By Name(w1635) -> ("ReadLeakDet?"=w1639:bool, "Labels"=w1633:string[])
        n501 = Array Size(array=w1633) -> (size(s)=w1638:i32)
        n502 = case shown="True" w1639 {
          tunnel: w1638 -> [w1645 w1647]
          tunnel: [w1645 w1646] -> w1636
          frame False {
          }
          frame True {
            n503 = Add(x=w1647, y=1) -> (x+y=w1646:i32)
          }
        }
        n504 = Initialize Array(TRUE ("Activate 2"), w1636) -> ()  [unwired: 1 out]
      }
    }
    "error out (USB6218)" <- w886
    n505 = case shown="True" w848 {
      frame False {
      }
      frame True {
        n506 = local read "RUN label"() -> (w1025:string)
        n507 = Get Date/Time In Seconds() -> (seconds since 1Jan1904=w1029:timestamp)
        n508 = call "LV_UNIXTIME.vi"("current time"=w1029) -> ("date/time string"=w1028:string)  [unwired: 9 in, 1 out]
        n509 = Concatenate Strings(w1028, "_" ("string"), w1025) -> (→"RUN Identifier" →"RUN Identifier 2" →"RUN Identifier 3" →"RUN Identifier 4" →"RUN Identifier 5" →"RUN Identifier 6" →"RUN Identifier 7":string)
      }
    }
    n510 = Equal?(x=w858, y=i64 0) -> (x = y?=w855:bool)
    n511 = local read "LastData (LSI218)"() -> (w868:dbl[])
    n512 = local read "Last Data \nLSI336"() -> (w867:dbl[])
    n513 = And(x="Analog Out ON?", y=w848) -> (x .and. y?=w884:bool)
    n514 = And(x=w855, y="Automatic \nScreenshots?") -> (x .and. y?=w854:bool)
    n515 = Build Array (concatenate)(w868, w867) -> (w866:dbl[])
    "AllTemperatures" <- w866
    n516 = Build Array (concatenate)(w870, w871) -> (w869:T19)
    "TempSensorsLocations" <- w869
    n517 = case shown="True" w884 {
      tunnel: w845 -> [_ w1418]
      tunnel: [w1394 w1409] -> w883
      tunnel: w882 -> [w1394 w1408]
      frame False {
      }
      frame True {
        w1401 = "_raw" ("string")
        w1425 = 10.0 ("V_lim_max")
        w1424 = 0.0 ("V_lim_min")
        w1423 = -1 items=["Default"=-1, "RSE"=10083, "Differential"=10106, "Pseudodifferential"=12529] ("output terminal configuration")
        w1422 = 10348 items=["Volts"=10348, "From Custom Scale"=10065] ("units")
        n518 = local read "RUN Identifier"() -> (w1407:string)
        n519 = Concatenate Strings(w1407, "_AO" ("string")) -> (w1427:string)
        n520 = Concatenate Strings(w1407, "_", "USB_AOUT.csv" ("string")) -> (w1419:string)
        n521 = Array To Cluster(array="AOUT Labels") -> (cluster=w1405:T29)
        n522 = Unbundle By Name(w1405) -> ("AOUT Labels[0]"=w1404:string, "AOUT Labels[1]"=w1402:string)
        n523 = Build Path(base path=w1418, name or relative path=w1419) -> (appended path=w1415:path)
        n524 = Concatenate Strings(w1404, w1401) -> (w1403:string)
        n525 = Concatenate Strings(w1402, w1401) -> (w1400:string)
        n526 = Open/Create/Replace File(file path (use dialog)=w1415, operation (0:open)=T25."open or create") -> (refnum out=w1413:refnum<file>)  [unwired: 4 in, 2 out]
        n527 = Build Array(w1404, w1402, w1403, w1400) -> (w1411:string[])
        n528 = call "FileIntialize.vi"("Error In"=w1408, "Labels"=w1411, "refnum in"=w1413) -> ("Error Out"=w1410:errorcluster, "File Refnum"=→"File Refn USB AO":refnum<file>)  [unwired: 7 in]
        n529 = call <vilib>:"DAQmx Create Task.vi"("new task name"=w1427, "auto cleanup"=FALSE, "error in"=w1410) -> ("task out"=w1426:refnum<k21>, "error out"=w1428:errorcluster)  [unwired: 11 in]
        n530 = Index Array(array="AOUT assignment", index #1=0 ("index"), index #2=1 ("index")) -> (element #1=w1397:tag, element #2=w1395:tag)
        n531 = call-poly <vilib>:"DAQmx Create Virtual Channel.vi"("task in"=w1426, "maximum value"=w1425, "minimum value"=w1424, "output terminal configuration"=w1423, "physical channels"=w1397, "units"=w1422, "error in"=w1428) -> ("task out"=w1430:refnum<k21>, "error out"=w1431:errorcluster)  [unwired: 7 in]
        n532 = call-poly <vilib>:"DAQmx Create Virtual Channel.vi"("task in"=w1430, "maximum value"=w1425, "minimum value"=w1424, "physical channels"=w1395, "error in"=w1431) -> ("task out"=w1433:refnum<k21>, "error out"=w1432:errorcluster)  [unwired: 9 in]
        n533 = call <vilib>:"DAQmx Start Task.vi"("task/channels in"=w1433, "error in"=w1432) -> ("task out"=→"AO task out":refnum<k21>, "error out"=w1409:errorcluster)  [unwired: 12 in]
      }
    }
    "error out (USB6210/6218 AOUT)" <- w883
    n534 = case shown="True" w854 {
      frame False {
      }
      frame True {
        n535 = flat-sequence {
          frame #0 {
            n536 = property on="Frontpanel screenshots" class="Bool (strict)"("Val(Sgnl)"=TRUE ("Value (Signaling)")) -> ()  [unwired: 2 in, 2 out]
          }
        }
      }
    }
    n537 = flat-sequence {
      tunnel: w866 -> [w1035]
      tunnel: w869 -> [w1036]
      tunnel: w861 -> [w1288]
      tunnel: w860 -> [w1287]
      frame #0 {
        n538 = stacked-sequence {
          tunnel: w1036 -> [w1041 w1046 w1051 w1056 w1061 w1066 w1071 w1076 w1081 w1086 w1091 w1096 w1101 w1106 w1111 w1116 w1121 w1126 w1131 w1136 w1141 w1146 w1151 w1156 w1161 w1166 w1171 w1176 w1181 w1186 w1191 w1196 w1201 w1206 w1211 w1216 w1221 w1226 w1231 w1236 w1241 w1246 w1251 w1256 w1261 w1266 w1271 w1276 w1281 w1286]
          tunnel: w1035 -> [w1039 w1044 w1049 w1054 w1059 w1064 w1069 w1074 w1079 w1084 w1089 w1094 w1099 w1104 w1109 w1114 w1119 w1124 w1129 w1134 w1139 w1144 w1149 w1154 w1159 w1164 w1169 w1174 w1179 w1184 w1189 w1194 w1199 w1204 w1209 w1214 w1219 w1224 w1229 w1234 w1239 w1244 w1249 w1254 w1259 w1264 w1269 w1274 w1279 w1284]
          frame #0 {
            n539 = Search 1D Array(1D array=w1041, element=T14."T3He1-1" ("SensorLocations")) -> (index of element=w1038:i32)  [unwired: 1 in]
            n540 = Index Array(array=w1039, index=w1038) -> (element=→"T3He1-1":dbl)
          }
          frame #1 {
            n541 = Search 1D Array(1D array=w1046, element=T14."T3He1-2" ("SensorLocations")) -> (index of element=w1043:i32)  [unwired: 1 in]
            n542 = Index Array(array=w1044, index=w1043) -> (element=→"T3He1-2":dbl)
          }
          frame #2 {
            n543 = Search 1D Array(1D array=w1051, element=T14."T3He1-3" ("SensorLocations")) -> (index of element=w1048:i32)  [unwired: 1 in]
            n544 = Index Array(array=w1049, index=w1048) -> (element=→"T3He1-3":dbl)
          }
          frame #3 {
            n545 = Search 1D Array(1D array=w1056, element=T14."T3He1-4" ("SensorLocations")) -> (index of element=w1053:i32)  [unwired: 1 in]
            n546 = Index Array(array=w1054, index=w1053) -> (element=→"T3He1-4":dbl)
          }
          frame #4 {
            n547 = Search 1D Array(1D array=w1061, element=T14."T3He2-1" ("SensorLocations")) -> (index of element=w1058:i32)  [unwired: 1 in]
            n548 = Index Array(array=w1059, index=w1058) -> (element=→"T3He2-1":dbl)
          }
          frame #5 {
            n549 = Search 1D Array(1D array=w1066, element=T14."T3He2-2" ("SensorLocations")) -> (index of element=w1063:i32)  [unwired: 1 in]
            n550 = Index Array(array=w1064, index=w1063) -> (element=→"T3He2-2":dbl)
          }
          frame #6 {
            n551 = Search 1D Array(1D array=w1071, element=T14."T3He3" ("SensorLocations")) -> (index of element=w1068:i32)  [unwired: 1 in]
            n552 = Index Array(array=w1069, index=w1068) -> (element=→"T3He3":dbl)
          }
          frame #7 {
            n553 = Search 1D Array(1D array=w1076, element=T14."T3He4" ("SensorLocations")) -> (index of element=w1073:i32)  [unwired: 1 in]
            n554 = Index Array(array=w1074, index=w1073) -> (element=→"T3He4":dbl)
          }
          frame #8 {
            n555 = Search 1D Array(1D array=w1081, element=T14."T3He5" ("SensorLocations")) -> (index of element=w1078:i32)  [unwired: 1 in]
            n556 = Index Array(array=w1079, index=w1078) -> (element=→"T3He5":dbl)
          }
          frame #9 {
            n557 = Search 1D Array(1D array=w1086, element=T14."T3He6-1" ("SensorLocations")) -> (index of element=w1083:i32)  [unwired: 1 in]
            n558 = Index Array(array=w1084, index=w1083) -> (element=→"T3He6-1" →"T3He6-1/6-2 (HEX1)":dbl)
          }
          frame #10 {
            n559 = Search 1D Array(1D array=w1091, element=T14."T3He6-2" ("SensorLocations")) -> (index of element=w1088:i32)  [unwired: 1 in]
            n560 = Index Array(array=w1089, index=w1088) -> (element=→"T3He6-2" →"T3He6-1/6-2 (3He pot) 2":dbl)
          }
          frame #11 {
            n561 = Search 1D Array(1D array=w1096, element=T14."T3He7-1" ("SensorLocations")) -> (index of element=w1093:i32)  [unwired: 1 in]
            n562 = Index Array(array=w1094, index=w1093) -> (element=→"T3He7-1" →"T3He7-1/7-2 (HEX1)":dbl)
          }
          frame #12 {
            n563 = Search 1D Array(1D array=w1101, element=T14."T3He7-2" ("SensorLocations")) -> (index of element=w1098:i32)  [unwired: 1 in]
            n564 = Index Array(array=w1099, index=w1098) -> (element=→"T3He7-2" →"T3He7-1/6-2 (3He pot) 2":dbl)
          }
          frame #13 {
            n565 = Search 1D Array(1D array=w1106, element=T14."T3He8" ("SensorLocations")) -> (index of element=w1103:i32)  [unwired: 1 in]
            n566 = Index Array(array=w1104, index=w1103) -> (element=→"T3He8":dbl)
          }
          frame #14 {
            n567 = Search 1D Array(1D array=w1111, element=T14."T3He9" ("SensorLocations")) -> (index of element=w1108:i32)  [unwired: 1 in]
            n568 = Index Array(array=w1109, index=w1108) -> (element=→"T3He9":dbl)
          }
          frame #15 {
            n569 = Search 1D Array(1D array=w1116, element=T14."T3He10" ("SensorLocations")) -> (index of element=w1113:i32)  [unwired: 1 in]
            n570 = Index Array(array=w1114, index=w1113) -> (element=→"T3He10":dbl)
          }
          frame #16 {
            n571 = Search 1D Array(1D array=w1121, element=T14."T4He1" ("SensorLocations")) -> (index of element=w1118:i32)  [unwired: 1 in]
            n572 = Index Array(array=w1119, index=w1118) -> (element=→"T4He1" →"T4He1 (4K reservoir )":dbl)
          }
          frame #17 {
            n573 = Search 1D Array(1D array=w1126, element=T14."T4He2-1" ("SensorLocations")) -> (index of element=w1123:i32)  [unwired: 1 in]
            n574 = Index Array(array=w1124, index=w1123) -> (element=→"T4He2-1":dbl)
          }
          frame #18 {
            n575 = Search 1D Array(1D array=w1131, element=T14."T4He2-2" ("SensorLocations")) -> (index of element=w1128:i32)  [unwired: 1 in]
            n576 = Index Array(array=w1129, index=w1128) -> (element=→"T4He2-2":dbl)
          }
          frame #19 {
            n577 = Search 1D Array(1D array=w1136, element=T14."T4He3-1" ("SensorLocations")) -> (index of element=w1133:i32)  [unwired: 1 in]
            n578 = Index Array(array=w1134, index=w1133) -> (element=→"T4He3-1":dbl)
          }
          frame #20 {
            n579 = Search 1D Array(1D array=w1141, element=T14."T4He3-2" ("SensorLocations")) -> (index of element=w1138:i32)  [unwired: 1 in]
            n580 = Index Array(array=w1139, index=w1138) -> (element=→"T4He3-2":dbl)
          }
          frame #21 {
            n581 = Search 1D Array(1D array=w1146, element=T14."T4He3-3" ("SensorLocations")) -> (index of element=w1143:i32)  [unwired: 1 in]
            n582 = Index Array(array=w1144, index=w1143) -> (element=→"T4He3-3":dbl)
          }
          frame #22 {
            n583 = Search 1D Array(1D array=w1151, element=T14."T4He3-4" ("SensorLocations")) -> (index of element=w1148:i32)  [unwired: 1 in]
            n584 = Index Array(array=w1149, index=w1148) -> (element=→"T4He3-4":dbl)
          }
          frame #23 {
            n585 = Search 1D Array(1D array=w1156, element=T14."T4He4" ("SensorLocations")) -> (index of element=w1153:i32)  [unwired: 1 in]
            n586 = Index Array(array=w1154, index=w1153) -> (element=→"T4He4":dbl)
          }
          frame #24 {
            n587 = Search 1D Array(1D array=w1161, element=T14."T4He5" ("SensorLocations")) -> (index of element=w1158:i32)  [unwired: 1 in]
            n588 = Index Array(array=w1159, index=w1158) -> (element=→"T4He5":dbl)
          }
          frame #25 {
            n589 = Search 1D Array(1D array=w1166, element=T14."T4He6" ("SensorLocations")) -> (index of element=w1163:i32)  [unwired: 1 in]
            n590 = Index Array(array=w1164, index=w1163) -> (element=→"T4He6":dbl)
          }
          frame #26 {
            n591 = Search 1D Array(1D array=w1171, element=T14."T4He7" ("SensorLocations")) -> (index of element=w1168:i32)  [unwired: 1 in]
            n592 = Index Array(array=w1169, index=w1168) -> (element=→"T4He7":dbl)
          }
          frame #27 {
            n593 = Search 1D Array(1D array=w1176, element=T14."T4He8" ("SensorLocations")) -> (index of element=w1173:i32)  [unwired: 1 in]
            n594 = Index Array(array=w1174, index=w1173) -> (element=→"T4He8":dbl)
          }
          frame #28 {
            n595 = Search 1D Array(1D array=w1181, element=T14."T4He9" ("SensorLocations")) -> (index of element=w1178:i32)  [unwired: 1 in]
            n596 = Index Array(array=w1179, index=w1178) -> (element=→"T4He9":dbl)
          }
          frame #29 {
            n597 = Search 1D Array(1D array=w1186, element=T14."T4He10" ("SensorLocations")) -> (index of element=w1183:i32)  [unwired: 1 in]
            n598 = Index Array(array=w1184, index=w1183) -> (element=→"T4He10":dbl)
          }
          frame #30 {
            n599 = Search 1D Array(1D array=w1191, element=T14."T1K1" ("SensorLocations")) -> (index of element=w1188:i32)  [unwired: 1 in]
            n600 = Index Array(array=w1189, index=w1188) -> (element=→"T1K1":dbl)
          }
          frame #31 {
            n601 = Search 1D Array(1D array=w1196, element=T14."T1K2" ("SensorLocations")) -> (index of element=w1193:i32)  [unwired: 1 in]
            n602 = Index Array(array=w1194, index=w1193) -> (element=→"T1K2":dbl)
          }
          frame #32 {
            n603 = Search 1D Array(1D array=w1201, element=T14."T1K3-1" ("SensorLocations")) -> (index of element=w1198:i32)  [unwired: 1 in]
            n604 = Index Array(array=w1199, index=w1198) -> (element=→"T1K3-1" →"T1K3-1/3-2 (1K pot)":dbl)
          }
          frame #33 {
            n605 = Search 1D Array(1D array=w1206, element=T14."T1K3-2" ("SensorLocations")) -> (index of element=w1203:i32)  [unwired: 1 in]
            n606 = Index Array(array=w1204, index=w1203) -> (element=→"T1K3-2" →"T1K3-1/3-2 (1K pot) 2":dbl)
          }
          frame #34 {
            n607 = Search 1D Array(1D array=w1211, element=T14."T1K4" ("SensorLocations")) -> (index of element=w1208:i32)  [unwired: 1 in]
            n608 = Index Array(array=w1209, index=w1208) -> (element=→"T1K4":dbl)
          }
          frame #35 {
            n609 = Search 1D Array(1D array=w1216, element=T14."T1K5" ("SensorLocations")) -> (index of element=w1213:i32)  [unwired: 1 in]
            n610 = Index Array(array=w1214, index=w1213) -> (element=→"T1K5":dbl)
          }
          frame #36 {
            n611 = Search 1D Array(1D array=w1221, element=T14."T1K6" ("SensorLocations")) -> (index of element=w1218:i32)  [unwired: 1 in]
            n612 = Index Array(array=w1219, index=w1218) -> (element=→"T1K6":dbl)
          }
          frame #37 {
            n613 = Search 1D Array(1D array=w1226, element=T14."TIP1" ("SensorLocations")) -> (index of element=w1223:i32)  [unwired: 1 in]
            n614 = Index Array(array=w1224, index=w1223) -> (element=→"TIP1":dbl)
          }
          frame #38 {
            n615 = Search 1D Array(1D array=w1231, element=T14."TIP2" ("SensorLocations")) -> (index of element=w1228:i32)  [unwired: 1 in]
            n616 = Index Array(array=w1229, index=w1228) -> (element=→"TIP2":dbl)
          }
          frame #39 {
            n617 = Search 1D Array(1D array=w1236, element=T14."TIP3" ("SensorLocations")) -> (index of element=w1233:i32)  [unwired: 1 in]
            n618 = Index Array(array=w1234, index=w1233) -> (element=→"TIP3":dbl)
          }
          frame #40 {
            n619 = Search 1D Array(1D array=w1241, element=T14."TIP4" ("SensorLocations")) -> (index of element=w1238:i32)  [unwired: 1 in]
            n620 = Index Array(array=w1239, index=w1238) -> (element=→"TIP4":dbl)
          }
          frame #41 {
            n621 = Search 1D Array(1D array=w1246, element=T14."TIP5" ("SensorLocations")) -> (index of element=w1243:i32)  [unwired: 1 in]
            n622 = Index Array(array=w1244, index=w1243) -> (element=→"TIP5":dbl)
          }
          frame #42 {
            n623 = Search 1D Array(1D array=w1251, element=T14."TIP6" ("SensorLocations")) -> (index of element=w1248:i32)  [unwired: 1 in]
            n624 = Index Array(array=w1249, index=w1248) -> (element=→"TIP6":dbl)
          }
          frame #43 {
            n625 = Search 1D Array(1D array=w1256, element=T14."TIP7" ("SensorLocations")) -> (index of element=w1253:i32)  [unwired: 1 in]
            n626 = Index Array(array=w1254, index=w1253) -> (element=→"TIP7":dbl)
          }
          frame #44 {
            n627 = Search 1D Array(1D array=w1261, element=T14."TTH1" ("SensorLocations")) -> (index of element=w1258:i32)  [unwired: 1 in]
            n628 = Index Array(array=w1259, index=w1258) -> (element=→"TTH1":dbl)
          }
          frame #45 {
            n629 = Search 1D Array(1D array=w1266, element=T14."TTH2" ("SensorLocations")) -> (index of element=w1263:i32)  [unwired: 1 in]
            n630 = Index Array(array=w1264, index=w1263) -> (element=→"TTH2":dbl)
          }
          frame #46 {
            n631 = Search 1D Array(1D array=w1271, element=T14."TTH3" ("SensorLocations")) -> (index of element=w1268:i32)  [unwired: 1 in]
            n632 = Index Array(array=w1269, index=w1268) -> (element=→"TTH3":dbl)
          }
          frame #47 {
            n633 = Search 1D Array(1D array=w1276, element=T14."TTH4" ("SensorLocations")) -> (index of element=w1273:i32)  [unwired: 1 in]
            n634 = Index Array(array=w1274, index=w1273) -> (element=→"TTH4":dbl)
          }
          frame #48 {
            n635 = Search 1D Array(1D array=w1281, element="SensorLocation 1") -> (index of element=w1278:i32)  [unwired: 1 in]
            n636 = Index Array(array=w1279, index=w1278) -> (element=→"Temperature 1":dbl)
          }
          frame #49 {
            n637 = Search 1D Array(1D array=w1286, element="SensorLocation 2") -> (index of element=w1283:i32)  [unwired: 1 in]
            n638 = Index Array(array=w1284, index=w1283) -> (element=→"Temperature 2":dbl)
          }
        }
      }
      frame #1 {
        n639 = stacked-sequence {
          tunnel: w1288 -> [w1293 w1298 w1303 w1308 w1313 w1318 w1323 w1328 w1333 w1338 w1343 w1348 w1353 w1358 w1363 w1368 w1373 w1378 w1383]
          tunnel: w1287 -> [w1290 w1296 w1302 w1307 w1312 w1316 w1321 w1326 w1331 w1336 w1341 w1346 w1350 w1355 w1360 w1365 w1370 w1375 _]
          tunnel: w1287 -> [_ _ _ _ _ _ _ _ _ _ _ _ _ _ _ _ _ _ w1381]
          frame #0 {
            n640 = Search 1D Array(1D array=w1293, element="Insulation vacuum") -> (index of element=w1291:i32)  [unwired: 1 in]
            n641 = Index Array(array=w1290, index=w1291) -> (element=→"P_ins" →"P (insulation)":dbl)
          }
          frame #1 {
            n642 = Search 1D Array(1D array=w1298, element="4K reservoir pressure") -> (index of element=w1295:i32)  [unwired: 1 in]
            n643 = Index Array(array=w1296, index=w1295) -> (element=→"P_4Kres" →"P (4K reservoir)":dbl)
          }
          frame #2 {
            n644 = Search 1D Array(1D array=w1303, element="3He inlet pressure") -> (index of element=w1301:i32)  [unwired: 1 in]
            n645 = Index Array(array=w1302, index=w1301) -> (element=→"P_3HeIN" →"P (3He IN)":dbl)
          }
          frame #3 {
            n646 = Search 1D Array(1D array=w1308, element="Shield return press.") -> (index of element=w1306:i32)  [unwired: 1 in]
            n647 = Index Array(array=w1307, index=w1306) -> (element=→"P_SldRTN" →"P (shield return)":dbl)
          }
          frame #4 {
            n648 = Search 1D Array(1D array=w1313, element="3He pot pressure") -> (index of element=w1311:i32)  [unwired: 1 in]
            n649 = Index Array(array=w1312, index=w1311) -> (element=→"P_3Hepot" →"P (3He pot)":dbl)
          }
          frame #5 {
            n650 = Search 1D Array(1D array=w1318, element="1Kpot pressure") -> (index of element=w1315:i32)  [unwired: 1 in]
            n651 = Index Array(array=w1316, index=w1315) -> (element=→"P_1Kpot" →"P (1K pot)":dbl)
          }
          frame #6 {
            n652 = Search 1D Array(1D array=w1323, element="Dewar pressure") -> (index of element=w1320:i32)  [unwired: 1 in]
            n653 = Index Array(array=w1321, index=w1320) -> (element=→"P_Dewar" →"P (Dewar)":dbl)
          }
          frame #7 {
            n654 = Search 1D Array(1D array=w1328, element="HEX7 out pressure") -> (index of element=w1325:i32)  [unwired: 1 in]
            n655 = Index Array(array=w1326, index=w1325) -> (element=→"P_HEX7OUT" →"P (HEX7 out)":dbl)
          }
          frame #8 {
            n656 = Search 1D Array(1D array=w1333, element="Diff pressure HEX4") -> (index of element=w1330:i32)  [unwired: 1 in]
            n657 = Index Array(array=w1331, index=w1330) -> (element=→"DP_HEX4" →"DP HEX4":dbl)
          }
          frame #9 {
            n658 = Search 1D Array(1D array=w1338, element="Diff pressure HEX5") -> (index of element=w1335:i32)  [unwired: 1 in]
            n659 = Index Array(array=w1336, index=w1335) -> (element=→"DP_HEX5" →"DP HEX5":dbl)
          }
          frame #10 {
            n660 = Search 1D Array(1D array=w1343, element="3He pump exhaust flow") -> (index of element=w1340:i32)  [unwired: 1 in]
            n661 = Index Array(array=w1341, index=w1340) -> (element=→"F_1" →"F1 (3He pump exhaust) flow":dbl)
          }
          frame #11 {
            n662 = Search 1D Array(1D array=w1348, element="Shield flow") -> (index of element=w1345:i32)  [unwired: 1 in]
            n663 = Index Array(array=w1346, index=w1345) -> (element=→"F_2" →"F2 (shield flow)":dbl)
          }
          frame #12 {
            n664 = Search 1D Array(1D array=w1353, element="4He return flow from HEX7") -> (index of element=w1351:i32)  [unwired: 1 in]
            n665 = Index Array(array=w1350, index=w1351) -> (element=→"F_3" →"F3 (4He rtn flw via HEX7)":dbl)
          }
          frame #13 {
            n666 = Search 1D Array(1D array=w1358, element="3He incoming flow into HEX7") -> (index of element=w1356:i32)  [unwired: 1 in]
            n667 = Index Array(array=w1355, index=w1356) -> (element=→"F_4" →"F4 (3He in to HEX7)":dbl)
          }
          frame #14 {
            n668 = Search 1D Array(1D array=w1363, element="1Kpot pump exhaust flow") -> (index of element=w1361:i32)  [unwired: 1 in]
            n669 = Index Array(array=w1360, index=w1361) -> (element=→"F_5" →"F5 (1K pump ex.)":dbl)
          }
          frame #15 {
            n670 = Search 1D Array(1D array=w1368, element="4K reservoir level") -> (index of element=w1366:i32)  [unwired: 1 in]
            n671 = Index Array(array=w1365, index=w1366) -> (element=→"L3" →"He level (4K)":dbl)
          }
          frame #16 {
            n672 = Search 1D Array(1D array=w1373, element="1K pot level") -> (index of element=w1371:i32)  [unwired: 1 in]
            n673 = Index Array(array=w1370, index=w1371) -> (element=→"L(1K) (a1)" →"He level (1K)":dbl)
          }
          frame #17 {
            n674 = Search 1D Array(1D array=w1378, element="1K pot (b)") -> (index of element=w1376:i32)  [unwired: 1 in]
            n675 = Index Array(array=w1375, index=w1376) -> (element=→"1K pot(b1)" →"He level (1K) b":dbl)
          }
          frame #18 {
            n676 = case shown="False" TRUE {
              tunnel: w1383 -> [w1388 _]
              tunnel: "3He pot" -> [w1387 w1392]
              tunnel: w1381 -> [w1385 _]
              tunnel: [w1384 w1391] -> w1380
              frame False {
                n677 = Search 1D Array(1D array=w1388, element=w1387) -> (index of element=w1386:i32)  [unwired: 1 in]
                n678 = Index Array(array=w1385, index=w1386) -> (element=w1384:dbl)
              }
              frame True {
                n679 = local read "Labels (HP34401 LM)"() -> (w1393:string[])
                n680 = local read "LastData (HP34401 LM)"() -> (w1389:dbl[])
                n681 = Search 1D Array(1D array=w1393, element=w1392) -> (index of element=w1390:i32)  [unwired: 1 in]
                n682 = Index Array(array=w1389, index=w1390) -> (element=w1391:dbl)
              }
            }
            "3He pot level" <- w1380
            "He level (3He)" <- w1380
          }
        }
      }
    }
    n683 = case shown="True" w848 {
      tunnel: [w1954 w1966] -> w908
      tunnel: [w1944 w1965] -> w916
      tunnel: [w1953 w1964] -> w909
      tunnel: [w1952 timestamp[] [] ("TimeArray")] -> w878
      tunnel: [w1951 dbl[][] [] ("DataArray")] -> w876
      tunnel: w918 -> [w1950 w1961]
      tunnel: w917 -> [w1949 w1960]
      tunnel: w842 -> [w1945 _]
      tunnel: w845 -> [_ w1955]
      frame False {
        n684 = local read "Record interval"() -> (w1942:i64)
        n685 = call-dynamic "LSI336Data_measure.vi"("LSI336Data in"=w1950, "MeasurementIndex"=w1945, "error in (no error)"=w1949, "save every ... measurements"=w1942) -> ("Active?"=→"Active?\n(LSI336)":bool[], "TimeMeasuremeent"=→"Time of Last Measurement (LSI336)":timestamp, "LSI336Data out"=w1953:refnum<class "LSI336Data.lvclass">, "LastData"=→"Last Data \nLSI336":dbl[], "LastMeasurementConfig"=→"LastMeasurementConfig (336)":T18, "DataArray"=w1951:dbl[][], "Status"=w1944:u16, "TimeArray"=w1952:timestamp[], "error out"=w1954:errorcluster)  [unwired: 3 in]
      }
      frame True {
        n686 = local read "RUN Identifier"() -> (w1956:string)
        n687 = call-dynamic "LSI336Data_initialize.vi"("LSI336Data in"=w1961, "RunIdentifier"=w1956, "InstName"="InstName (LSI336)", "FileFormat"="FileFormat (336)", "LSI336Settings(X, Y)"="LSI336Settings(X,Y)", "error in (no error)"=w1960, "base path"=w1955) -> ("LSI336Data out"=w1964:refnum<class "LSI336Data.lvclass">, "Status"=w1965:T7, "AllLabels"=→"Labels LSI336":string[], "error out"=w1966:errorcluster)  [unwired: 5 in]
      }
    }
    "LSI336 Status" <- w916
    "error out (LSI336)" <- w908
    "TimeArray (LSI336)" <- w878
    "DataArray (336)" <- w876
    n688 = local read "Labels (HP34401 LM) 2"() -> (w841:string[])
    n689 = case shown="False" w848 {
      tunnel: [w2059 w2074] -> w921
      tunnel: [w2054 w2073] -> w938
      tunnel: [w2057 w2072] -> w922
      tunnel: w842 -> [w2058 _]
      tunnel: w937 -> [w2048 w2067]
      tunnel: w936 -> [w2049 w2066]
      tunnel: w845 -> [_ w2065]
      tunnel: [w2046 timestamp[] [] ("TimeArray")] -> w935
      tunnel: [w2045 dbl[][] [] ("DataArray")] -> w934
      frame False {
        w2052 = 24 ("index")
        n690 = local read "Record interval"() -> (w2043:i64)
        n691 = call-dynamic "LSI218Data_measure.vi"("LSI218Data in"=w2049, "MeasurementIndex"=w2058, "error in (no error)"=w2048, "save every ... measurements"=w2043) -> ("TimeMeasuremeent"=→"Time of Last Measurement (LSI218)":timestamp, "Active?"=w2053:bool[], "LSI218Data out"=w2057:refnum<class "LSI218Data.lvclass">, "LastMeasurementConfig"=→"LastMeasurementConfig (218)":T18, "LastData"=w2047:dbl[], "Status"=w2054:u16, "TimeArray"=w2046:timestamp[], "DataArray"=w2045:dbl[][], "error out"=w2059:errorcluster)  [unwired: 3 in]
        "LastData (LSI218)" <- w2047
        n692 = Split 1D Array(array=w2053, index=w2052) -> (first subarray=→"Active?\n (1)":bool[], second subarray=→"Active?\n(2)":bool[])
        n693 = Split 1D Array(array=w2047, index=w2052) -> (first subarray=→"Last Data \nLSI218 (1)":dbl[], second subarray=→"Last Data \nLSI218 (2)":dbl[])
      }
      frame True {
        n694 = local read "RUN Identifier"() -> (w2061:string)
        n695 = call-dynamic "LSI218Data_initialize.vi"("LSI218Settings(A-F)"="LSI218Settings(A-F)", "FileFormat"="FileFormat (218)", "base path"=w2065, "error in (no error)"=w2067, "InstName"="InstName (LSI218)", "RunIdentifier"=w2061, "LSI218Data in"=w2066) -> ("error out"=w2074:errorcluster, "Status"=w2073:T7, "AllLabels"=w2064:string[], "LSI218Data out"=w2072:refnum<class "LSI218Data.lvclass">)  [unwired: 1 in]
        n696 = Split 1D Array(array=w2064, index=24) -> (first subarray=→"Labels LSI218 (1)":string[], second subarray=→"Labels LSI218 (2)":string[])
      }
    }
    "LSI218 Status" <- w938
    "error out (LSI218)" <- w921
    n697 = case shown="True" w848 {
      tunnel: w847 -> [w1010 w1024]
      tunnel: [w1007 w1023] -> w846
      tunnel: w845 -> [_ w1021]
      tunnel: w844 -> [w1009 w1020]
      tunnel: [w1006 w1017] -> w843
      tunnel: w842 -> [w1008 _]
      tunnel: [w1004 dbl[][] [] ("LastDataArray")] -> w839
      tunnel: [w1003 timestamp[] [] ("LastTimeArray")] -> w837
      frame False {
        n698 = call-dynamic "LMData_measure.vi"("error in (no error)"=w1009, "MeasurementInterval(>0)"="LM measurement interval (>0)", "MeasurementIndex"=w1008, "LMData in"=w1010) -> ("error out"=w1006:errorcluster, "LastDataArray"=w1004:dbl[][], "LastMeasurement"=→"LastData (HP34401 LM)":dbl[], "LMData out"=w1007:refnum<class "LMData.lvclass">, "LastTimeArray"=w1003:timestamp[])  [unwired: 3 in]
      }
      frame True {
        n699 = local read "RUN Identifier"() -> (w1022:string)
        n700 = call-dynamic "LMData_initialize.vi"("LMData in"=w1024, "VISA resource name"="VISA (HP34401 LM)", "Labels"="Labels (HP34401 LM)", "FileFormat"="FileFormat (HP34401 LM)", "RunIdentifier"=w1022, "InstName"="InstName (HP34401 LM)", "base path"=w1021, "error in (no error)"=w1020, "LevelCalibration (R0, R1, L0, L1)"="LevelCalibration (R0, R1, L0, L1)", "Active?"="Active? (HP34401 LM)") -> ("LMData out"=w1023:refnum<class "LMData.lvclass">, "error out"=w1017:errorcluster)  [unwired: 4 in]
        "Labels (HP34401 LM) 2" <- "Labels (HP34401 LM)"
      }
    }
    "error out (HP34401 LM)" <- w843
    n701 = Array Size(array=w841) -> (size(s)=w840:i32)
    n702 = for {
      N: w840 -> [_]
      tunnel: w839 -> [w964]
      shift-right: [w951] -> w833
      shift-left: w838 -> [w950]
      shift-right: [w954] -> w835
      shift-left: w838 -> [w955]
      shift-right: [w958] -> w836
      shift-left: w838 -> [w959]
      shift-right: [w953] -> w834
      shift-left: w838 -> [w952]
      tunnel: w837 -> [w962]
      i -> [w963]
      n703 = local read "Plot selecter (HP34401A)\n    1      2     3     4"() -> (w969:bool[][])
      n704 = Index Array(array=w964, index (col)=w963) -> (element=w961:dbl[])  [unwired: 1 in]
      n705 = Bundle("LastTimeArray"=w962, "LastDataArray"=w961) -> (w960:T30)  [unwired: 1 in]
      n706 = Index Array(array=w969, index (row) #1=w963, index (col) #1=0 ("disabled index (col)"), index (row) #2=w963, index (col) #2=1 ("index (col)"), index (row) #3=w963, index (col) #3=2 ("index (col)"), index (row) #4=w963, index (col) #4=3 ("disabled index (col)")) -> (element #1=w957:bool, element #2=w956:bool, element #3=w949:bool, element #4=w948:bool)
      n707 = stacked-sequence {
        tunnel: w960 -> [w971 w978 w989 w997]
        tunnel: w959 -> [w973 _ _ _]
        tunnel: [w972 _ _ _] -> w958
        tunnel: w957 -> [w970 _ _ _]
        tunnel: w956 -> [_ w981 _ _]
        tunnel: w955 -> [_ w980 _ _]
        tunnel: [_ w979 _ _] -> w954
        tunnel: [_ _ w988 _] -> w953
        tunnel: w952 -> [_ _ w987 _]
        tunnel: [_ _ _ w996] -> w951
        tunnel: w950 -> [_ _ _ w995]
        tunnel: w949 -> [_ _ w986 _]
        tunnel: w948 -> [_ _ _ w994]
        frame #0 {
          n708 = case shown="True" w970 {
            tunnel: w973 -> [w974 w977]
            tunnel: [w974 w976] -> w972
            tunnel: w971 -> [_ w975]
            frame False {
            }
            frame True {
              n709 = Build Array (concatenate)(w977, w975) -> (w976:T31)
            }
          }
        }
        frame #1 {
          n710 = case shown="True" w981 {
            tunnel: [w982 w985] -> w979
            tunnel: w980 -> [w982 w984]
            tunnel: w978 -> [_ w983]
            frame False {
            }
            frame True {
              n711 = Build Array (concatenate)(w984, w983) -> (w985:T31)
            }
          }
        }
        frame #2 {
          n712 = case shown="True" w986 {
            tunnel: [w990 w993] -> w988
            tunnel: w989 -> [_ w992]
            tunnel: w987 -> [w990 w991]
            frame False {
            }
            frame True {
              n713 = Build Array (concatenate)(w991, w992) -> (w993:T31)
            }
          }
        }
        frame #3 {
          n714 = case shown="True" w994 {
            tunnel: [w998 w1001] -> w996
            tunnel: w997 -> [_ w1000]
            tunnel: w995 -> [w998 w999]
            frame False {
            }
            frame True {
              n715 = Build Array (concatenate)(w999, w1000) -> (w1001:T31)
            }
          }
        }
      }
    }
    n716 = local read "Last Data \n(USB6210)"() -> (w862:dbl[])
    n717 = local read "Last Data \n(USB6218)"() -> (w863:dbl[])
    n718 = local read "All Labels (USB6210)"() -> (w865:string[])
    n719 = local read "All Labels (USB6218)"() -> (w864:string[])
    n720 = flat-sequence {
      tunnel: w892 -> [w1452]
      tunnel: [w1447] -> w891
      tunnel: [w1445] -> w890
      tunnel: [w1444] -> w889
      tunnel: [w1443] -> w888
      tunnel: w893 -> [w1439]
      frame #0 {
        w1446 = T26 [] ("appended array")
        n721 = Unbundle By Name(w1439) -> ("TimeArray"=w1435:timestamp[], "DataArrayConv"=w1450:dbl[][], "LDArray"=w1449:dbl[])
        "TimeArray (USB6218)" <- w1435
        n722 = Unbundle By Name(w1452) -> ("ReadLeakDet?"=w1451:bool, "LabelLD"=w1454:string, "Labels"=w1448:string[])  [unwired: 1 out]
        n723 = case shown="True" w1451 {
          tunnel: w1454 -> [_ w1462]
          tunnel: w1450 -> [w1456 w1461]
          tunnel: w1449 -> [_ w1460]
          tunnel: [w1456 w1459] -> w1437
          tunnel: w1448 -> [w1455 w1458]
          tunnel: [w1455 w1457] -> w1440
          frame False {
          }
          frame True {
            n724 = Build Array (concatenate)(w1461, w1460) -> (w1459:dbl[][])
            n725 = Build Array (concatenate)(w1458, w1462) -> (w1457:string[])
          }
        }
        "All Labels (USB6218)" <- w1440
        "DataArrayConv (USB6218)" <- w1437
        n726 = Array Size(array=w1435) -> (size(s)=→"TimeArray size (6218)":i32)
        n727 = local read "Plot selecter (USB6218)\n    1      2     3     4"() -> (w1442:bool[][])
        n728 = control-ref of="Plot selecter (USB6218)\n    1      2     3     4"() -> (w1438:refnum<vi>)
        n729 = Array Size(array=w1440) -> (size(s)=w1441:i32)
        n730 = Array Size(array=w1440) -> (size(s)=w1453:i32)
        n731 = Array Size(array=w1437) -> (size(s)=→"DataArraySize (6218)":i32[])
        n732 = property on="Property Node" class="Arr (strict)"(reference=w1438, "Number of Rows"=w1441) -> ()  [unwired: 1 in, 2 out]
        n733 = for {
          N: w1453 -> [_]
          tunnel: w1437 -> [w1483]
          tunnel: w1435 -> [w1484]
          shift-right: [w1478] -> w1445
          shift-left: w1446 -> [w1481]
          shift-right: [w1476] -> w1443
          shift-left: w1446 -> [w1479]
          shift-right: [w1477] -> w1447
          shift-left: w1446 -> [w1475]
          shift-right: [w1474] -> w1444
          shift-left: w1446 -> [w1473]
          tunnel: w1442 -> [w1472]
          i -> [w1467]
          n734 = Index Array(array=w1483, index (col)=w1467) -> (element=w1482:dbl[])  [unwired: 1 in]
          n735 = Index Array(array=w1472, index (row) #1=w1467, index (col) #1=0 ("index (row)"), index (row) #2=w1467, index (col) #2=1 ("index (row)"), index (row) #3=w1467, index (col) #3=2 ("index (row)"), index (row) #4=w1467, index (col) #4=3 ("index (row)")) -> (element #1=w1466:bool, element #2=w1465:bool, element #3=w1464:bool, element #4=w1463:bool)
          n736 = Bundle("TimeArray"=w1484, "DataArrayConv"=w1482) -> (w1480:T32)  [unwired: 1 in]
          n737 = stacked-sequence {
            tunnel: w1466 -> [w1488 _ _ _]
            tunnel: w1481 -> [_ w1496 _ _]
            tunnel: w1464 -> [_ _ w1504 _]
            tunnel: w1480 -> [w1485 w1494 w1503 w1509]
            tunnel: w1463 -> [_ _ _ w1512]
            tunnel: w1479 -> [_ _ _ w1511]
            tunnel: [_ _ _ w1510] -> w1476
            tunnel: [_ w1495 _ _] -> w1478
            tunnel: [w1487 _ _ _] -> w1477
            tunnel: w1475 -> [w1486 _ _ _]
            tunnel: [_ _ w1502 _] -> w1474
            tunnel: w1473 -> [_ _ w1501 _]
            tunnel: w1465 -> [_ w1493 _ _]
            frame #0 {
              n738 = case shown="True" w1488 {
                tunnel: [w1489 w1492] -> w1487
                tunnel: w1485 -> [_ w1491]
                tunnel: w1486 -> [w1489 w1490]
                frame False {
                }
                frame True {
                  n739 = Build Array (concatenate)(w1490, w1491) -> (w1492:T26)
                }
              }
            }
            frame #1 {
              n740 = case shown="True" w1493 {
                tunnel: w1496 -> [w1497 w1500]
                tunnel: [w1497 w1499] -> w1495
                tunnel: w1494 -> [_ w1498]
                frame False {
                }
                frame True {
                  n741 = Build Array (concatenate)(w1500, w1498) -> (w1499:T26)
                }
              }
            }
            frame #2 {
              n742 = case shown="True" w1504 {
                tunnel: [w1505 w1508] -> w1502
                tunnel: w1503 -> [_ w1507]
                tunnel: w1501 -> [w1505 w1506]
                frame False {
                }
                frame True {
                  n743 = Build Array (concatenate)(w1506, w1507) -> (w1508:T26)
                }
              }
            }
            frame #3 {
              n744 = case shown="True" w1512 {
                tunnel: [w1513 w1516] -> w1510
                tunnel: w1509 -> [_ w1515]
                tunnel: w1511 -> [w1513 w1514]
                frame False {
                }
                frame True {
                  n745 = Build Array (concatenate)(w1514, w1515) -> (w1516:T26)
                }
              }
            }
          }
        }
      }
    }
    n746 = case shown="True" "Digital Out ON?" {
      tunnel: w848 -> [_ w1655]
      tunnel: w898 -> [w1649 w1654]
      tunnel: [w1649 w1653] -> w897
      tunnel: w896 -> [_ w1652]
      tunnel: w845 -> [_ w1651]
      tunnel: w879 -> [_ w1650]
      frame False {
      }
      frame True {
        n747 = case shown="True" w1655 {
          tunnel: w1654 -> [w1673 w1856]
          tunnel: [w1673 w1869] -> w1653
          tunnel: w1652 -> [w1674 _]
          tunnel: w1651 -> [_ w1848]
          tunnel: w1650 -> [_ _]
          frame False {
            n748 = flat-sequence {
              frame #0 {
              }
            }
            n749 = case shown="\"USB6218AI\"" "AutoFill Source (P)" {
              tunnel: [w1677 w1678] -> w1659
              frame "USB6210", Default {
                n750 = local read "All Labels (USB6210)"() -> (w1677:string[])
              }
              frame "USB6218AI" {
                n751 = local read "All Labels (USB6218)"() -> (w1678:string[])
              }
            }
            n752 = case shown="\"USB6210\", Default" "AutoFill Source (L)" {
              tunnel: [w1675 w1676] -> w1656
              frame "USB6210", Default {
                n753 = local read "All Labels (USB6210)"() -> (w1675:string[])
              }
              frame "USB6218AI" {
                n754 = local read "All Labels (USB6218)"() -> (w1676:string[])
              }
            }
            n755 = Multiply(x="N for sampling", y=i64 2) -> (x*y=w1668:i64)
            n756 = local read "Cycle #"() -> (w1672:u32)
            n757 = Search 1D Array(1D array=w1659, element="Auto Fll Dewar P. label") -> (index of element=→"Target Index (P)":i32)  [unwired: 1 in]
            n758 = Search 1D Array(1D array=w1656, element="Auto Fll He L. label") -> (index of element=→"Target Index (L)":i32)  [unwired: 1 in]
            n759 = Add(x=w1668, y="Mov. Avg Interval") -> (x+y=w1670:i64)
            n760 = Greater?(x=w1672, y=w1670) -> (0:w1666:bool)
            n761 = And(x=w1666, y="Auto Fill ON?") -> (x .and. y?=w1664:bool)
            n762 = case shown="True" w1664 {
              tunnel: w1674 -> [_ w1712]
              tunnel: "Mov. Avg Interval" -> [_ w1698]
              tunnel: w1668 -> [_ w1685]
              tunnel: "N for sampling" -> [_ w1696]
              frame False {
              }
              frame True {
                n763 = local read "AutoFill Source (L)"() -> (w1679:T8)
                n764 = local read "AutoFill Source (P)"() -> (w1680:T8)
                n765 = case shown="\"USB6218AI\"" w1680 {
                  tunnel: [w1716 w1717] -> w1681
                  frame "USB6210", Default {
                    n766 = local read "DataArrayConv (USB6210)"() -> (w1716:dbl[][])
                  }
                  frame "USB6218AI" {
                    n767 = local read "DataArrayConv (USB6218)"() -> (w1717:dbl[][])
                  }
                }
                n768 = case shown="\"USB6210\", Default" w1679 {
                  tunnel: [w1714 w1715] -> w1683
                  frame "USB6210", Default {
                    n769 = local read "DataArrayConv (USB6210)"() -> (w1714:dbl[][])
                  }
                  frame "USB6218AI" {
                    n770 = local read "DataArrayConv (USB6218)"() -> (w1715:dbl[][])
                  }
                }
                n771 = local read "Pstd"() -> (→"Pstd history":dbl)
                n772 = local read "Lstd"() -> (→"Lstd history":dbl)
                n773 = local read "Target Index (L)"() -> (w1684:i32)
                n774 = local read "Pav (Pa)"() -> (→"Pav history":dbl)
                n775 = local read "Lav (%)"() -> (→"Lav history":dbl)
                n776 = Index Array(array=w1683, index (col)=w1684) -> (element=w1682:dbl[])  [unwired: 1 in]
                n777 = local read "Target Index (P)"() -> (w1713:i32)
                n778 = Unbundle By Name(w1712) -> ("TimeArray"=w1711:timestamp[])
                n779 = Index Array(array=w1681, index (col)=w1713) -> (element=w1700:dbl[])  [unwired: 1 in]
                n780 = Delete From Array(array=w1700, length=w1685) -> (deleted portion=w1708:dbl[])  [unwired: 1 in, 1 out]
                n781 = Delete From Array(array=w1682, length=w1685) -> (deleted portion=w1695:dbl[])  [unwired: 1 in, 1 out]
                n782 = call "MovingAverage.vi"("Moving Average interval"=w1698, "Input Array"=w1682) -> ("M.A. Array"=w1697:dbl[])  [unwired: 9 in]
                n783 = call "MovingAverage.vi"("Moving Average interval"=w1698, "Input Array"=w1700) -> ("M.A. Array"=w1699:dbl[])  [unwired: 9 in]
                n784 = Delete From Array(array=w1699, length=w1685) -> (deleted portion=w1709:dbl[])  [unwired: 1 in, 1 out]
                n785 = Delete From Array(array=w1699, length=w1685) -> (deleted portion=w1705:dbl[])  [unwired: 1 in, 1 out]
                "Last N M.A. Pressures" <- w1705
                n786 = Delete From Array(array=w1697, length=w1685) -> (deleted portion=w1690:dbl[])  [unwired: 1 in, 1 out]
                "Last N M.A. Levels" <- w1690
                n787 = Delete From Array(array=w1711, length=w1685) -> (deleted portion=w1692:timestamp[])  [unwired: 1 in, 1 out]
                n788 = Bundle("TimeArray"=w1692, "DataArrayConv (USB6218)"=w1708) -> (w1707:T33)  [unwired: 1 in]
                n789 = Bundle("TimeArray"=w1692, "M.A. Array"=w1709) -> (w1710:T34)  [unwired: 1 in]
                n790 = Bundle("TimeArray"=w1692, "DataArrayConv (USB6218)"=w1695) -> (w1694:T33)  [unwired: 1 in]
                n791 = Bundle("TimeArray"=w1692, "M.A. Array"=w1690) -> (w1691:T34)  [unwired: 1 in]
                n792 = Array Size(array=w1705) -> (size(s)=w1704:i32)
                n793 = Greater Or Equal?(x=w1704, y=w1696) -> (x >= y?=w1703:bool)
                n794 = Build Array(w1707, w1710) -> (→"Dewar Pressure":T35)
                n795 = Build Array(w1694, w1691) -> (→"He Level":T35)
                n796 = case shown="True" w1703 {
                  tunnel: [w1821 w1826] -> w1689
                  tunnel: w1705 -> [_ w1827]
                  tunnel: w1690 -> [_ w1824]
                  tunnel: [w1821 w1822] -> w1688
                  frame False {
                    w1821 = nan ("mean")
                  }
                  frame True {
                    n797 = call <vilib>:"Std Deviation and Variance.vi"("X"=w1827) -> ("mean"=w1826:dbl, "standard deviation"=w1825:dbl)  [unwired: 1 in, 1 out]
                    n798 = call <vilib>:"Std Deviation and Variance.vi"("X"=w1824) -> ("mean"=w1822:dbl, "standard deviation"=w1823:dbl)  [unwired: 1 in, 1 out]
                    n799 = local write "Pstd"(w1825) -> ()
                    n800 = local write "Lstd"(w1823) -> ()
                    n801 = local write "Pav (Pa)"(w1826) -> ()
                    n802 = local write "Lav (%)"(w1822) -> ()
                  }
                }
                n803 = flat-sequence {
                  tunnel: w1689 -> [w1718]
                  tunnel: w1688 -> [w1719]
                  frame #0 {
                    n804 = flat-sequence {
                      tunnel: w1719 -> [w1721]
                      tunnel: w1718 -> [w1720]
                      tunnel: w1718 -> [w1789]
                      frame #0 {
                        n805 = stacked-sequence {
                          tunnel: w1721 -> [w1728 w1732 _ _ _ _]
                          tunnel: w1720 -> [_ _ w1746 w1755 w1764 w1773]
                          frame #0 {
                            n806 = local read "L_low (%)"() -> (w1727:dbl)
                            n807 = local read "Fill state"() -> (w1725:bool)
                            n808 = Less?(x=w1728, y=w1727) -> (x < y?=w1724:bool)
                            n809 = Equal?(x=w1725, y=FALSE) -> (x = y?=w1723:bool)
                            n810 = And(x=w1724, y=w1723) -> (x .and. y?=w1722:bool)
                            n811 = case shown="False" w1722 {
                              frame False {
                              }
                              frame True {
                                w1730 = TRUE ("Value (Signaling)")
                                n812 = property on="Fill state" class="Bool (strict)"("Val(Sgnl)"=w1730) -> ()  [unwired: 2 in, 2 out]
                                n813 = Not(x=w1730) -> (.not. x?=w1729:bool)
                                n814 = property on="Fill (false)" class="Bool (strict)"("Val(Sgnl)"=w1729) -> ()  [unwired: 2 in, 2 out]
                              }
                            }
                          }
                          frame #1 {
                            n815 = local read "L_high (%)"() -> (w1733:dbl)
                            n816 = local read "Fill state"() -> (w1736:bool)
                            n817 = Greater?(x=w1732, y=w1733) -> (0:w1731:bool)
                            n818 = Equal?(x=w1736, y=TRUE) -> (x = y?=w1735:bool)
                            n819 = And(x=w1731, y=w1735) -> (x .and. y?=w1734:bool)
                            n820 = case shown="True" w1734 {
                              frame False {
                              }
                              frame True {
                                w1738 = FALSE ("Value (Signaling)")
                                n821 = property on="Fill state" class="Bool (strict)"("Val(Sgnl)"=w1738) -> ()  [unwired: 2 in, 2 out]
                                n822 = Not(x=w1738) -> (.not. x?=w1739:bool)
                                n823 = property on="Fill (false)" class="Bool (strict)"("Val(Sgnl)"=w1739) -> ()  [unwired: 2 in, 2 out]
                              }
                            }
                          }
                          frame #2 {
                            n824 = local read "P_1_low (Pa)"() -> (w1745:dbl)
                            n825 = property on="state 1" class="Bool (strict)"() -> ("Value"=w1743:bool)  [unwired: 2 in, 2 out]
                            n826 = Less?(x=w1746, y=w1745) -> (x < y?=w1742:bool)
                            n827 = Equal?(x=w1743, y=FALSE) -> (x = y?=w1741:bool)
                            n828 = And(x=w1741, y=w1742) -> (x .and. y?=w1740:bool)
                            n829 = case shown="True" w1740 {
                              frame False {
                              }
                              frame True {
                                w1748 = TRUE ("Value (Signaling)")
                                n830 = property on="state 1" class="Bool (strict)"("Val(Sgnl)"=w1748) -> ()  [unwired: 2 in, 2 out]
                                n831 = Not(x=w1748) -> (.not. x?=w1747:bool)
                                n832 = property on="state 1 (false)" class="Bool (strict)"("Val(Sgnl)"=w1747) -> ()  [unwired: 2 in, 2 out]
                              }
                            }
                          }
                          frame #3 {
                            n833 = local read "P_1_high (Pa)"() -> (w1754:dbl)
                            n834 = property on="state 1" class="Bool (strict)"() -> ("Value"=w1752:bool)  [unwired: 2 in, 2 out]
                            n835 = Greater?(x=w1755, y=w1754) -> (0:w1751:bool)
                            n836 = Equal?(x=w1752, y=TRUE) -> (x = y?=w1750:bool)
                            n837 = And(x=w1750, y=w1751) -> (x .and. y?=w1749:bool)
                            n838 = case shown="True" w1749 {
                              frame False {
                              }
                              frame True {
                                w1757 = FALSE ("Value (Signaling)")
                                n839 = property on="state 1" class="Bool (strict)"("Val(Sgnl)"=w1757) -> ()  [unwired: 2 in, 2 out]
                                n840 = Not(x=w1757) -> (.not. x?=w1756:bool)
                                n841 = property on="state 1 (false)" class="Bool (strict)"("Val(Sgnl)"=w1756) -> ()  [unwired: 2 in, 2 out]
                              }
                            }
                          }
                          frame #4 {
                            n842 = local read "P_2_low (Pa)"() -> (w1763:dbl)
                            n843 = property on="state 2" class="Bool (strict)"() -> ("Value"=w1758:bool)  [unwired: 2 in, 2 out]
                            n844 = Less?(x=w1764, y=w1763) -> (x < y?=w1761:bool)
                            n845 = Equal?(x=w1758, y=FALSE) -> (x = y?=w1760:bool)
                            n846 = And(x=w1760, y=w1761) -> (x .and. y?=w1759:bool)
                            n847 = case shown="True" w1759 {
                              frame False {
                              }
                              frame True {
                                w1765 = TRUE ("Value (Signaling)")
                                n848 = property on="state 2" class="Bool (strict)"("Val(Sgnl)"=w1765) -> ()  [unwired: 2 in, 2 out]
                                n849 = Not(x=w1765) -> (.not. x?=w1766:bool)
                                n850 = property on="state 2 (false)" class="Bool (strict)"("Val(Sgnl)"=w1766) -> ()  [unwired: 2 in, 2 out]
                              }
                            }
                          }
                          frame #5 {
                            n851 = local read "P_2_high (Pa)"() -> (w1772:dbl)
                            n852 = property on="state 2" class="Bool (strict)"() -> ("Value"=w1767:bool)  [unwired: 2 in, 2 out]
                            n853 = Greater?(x=w1773, y=w1772) -> (0:w1770:bool)
                            n854 = Equal?(x=w1767, y=TRUE) -> (x = y?=w1769:bool)
                            n855 = And(x=w1769, y=w1770) -> (x .and. y?=w1768:bool)
                            n856 = case shown="True" w1768 {
                              frame False {
                              }
                              frame True {
                                w1774 = FALSE ("Value (Signaling)")
                                n857 = property on="state 2" class="Bool (strict)"("Val(Sgnl)"=w1774) -> ()  [unwired: 2 in, 2 out]
                                n858 = Not(x=w1774) -> (.not. x?=w1775:bool)
                                n859 = property on="state 2 (false)" class="Bool (strict)"("Val(Sgnl)"=w1775) -> ()  [unwired: 2 in, 2 out]
                              }
                            }
                          }
                        }
                      }
                      frame #1 {
                        n860 = property on="Fill state" class="Bool (strict)"() -> ("Value"=w1776:bool)  [unwired: 2 in, 2 out]
                        n861 = case shown="True" w1776 {
                          frame False {
                            n862 = property on="V1 (N.O.)" class="Bool (strict)"("Val(Sgnl)"=TRUE ("V1 (N.O.)")) -> ()  [unwired: 2 in, 2 out]
                            n863 = property on="V2 (N.C.)" class="Bool (strict)"("Val(Sgnl)"=FALSE ("Value (Signaling)")) -> ()  [unwired: 2 in, 2 out]
                          }
                          frame True {
                            n864 = property on="state 1" class="Bool (strict)"() -> ("Value"=w1780:bool)  [unwired: 2 in, 2 out]
                            n865 = property on="state 2" class="Bool (strict)"() -> ("Value"=w1779:bool)  [unwired: 2 in, 2 out]
                            n866 = case shown="True" w1780 {
                              frame False {
                                n867 = property on="V1 (N.O.)" class="Bool (strict)"("Val(Sgnl)"=TRUE ("Value (Signaling)")) -> ()  [unwired: 2 in, 2 out]
                                n868 = local write "Status V1 CTRL"(enum16{"Pressurize", "Release"}."Release" ("Status V1 CTRL")) -> ()
                              }
                              frame True {
                                n869 = property on="V1 (N.O.)" class="Bool (strict)"("Val(Sgnl)"=FALSE ("V1 (N.O.)")) -> ()  [unwired: 2 in, 2 out]
                                n870 = local write "Status V1 CTRL"(enum16{"Pressurize", "Release"}."Pressurize" ("Status V1 CTRL")) -> ()
                              }
                            }
                            n871 = case shown="True" w1779 {
                              frame False {
                                n872 = property on="V2 (N.C.)" class="Bool (strict)"("Val(Sgnl)"=FALSE ("Value (Signaling)")) -> ()  [unwired: 2 in, 2 out]
                                n873 = local write "Status V2 CTRL"(enum16{"Pressurize", "Release"}."Release" ("Status V2 CTRL")) -> ()
                              }
                              frame True {
                                n874 = property on="V2 (N.C.)" class="Bool (strict)"("Val(Sgnl)"=TRUE ("Value (Signaling)")) -> ()  [unwired: 2 in, 2 out]
                                n875 = local write "Status V2 CTRL"(enum16{"Pressurize", "Release"}."Pressurize" ("Status V2 CTRL")) -> ()
                              }
                            }
                          }
                        }
                      }
                      frame #2 {
                        n876 = Greater?(x=w1789, y="P_safelimit_high (Pa)") -> (0:w1791:bool)
                        n877 = Less?(x=w1789, y="P_safelimit_low (Pa)") -> (x < y?=w1793:bool)
                        n878 = Or(x=w1791, y=w1793) -> (x .or. y?=w1794:bool)
                        n879 = case shown="False" w1794 {
                          frame False {
                          }
                          frame True {
                            w1795 = FALSE ("Value (Signaling)")
                            w1797 = FALSE ("Value (Signaling)")
                            n880 = property on="V2 (N.C.)" class="Bool (strict)"("Val(Sgnl)"=FALSE ("V1 (N.O.)")) -> ()  [unwired: 2 in, 2 out]
                            n881 = property on="state 1" class="Bool (strict)"("Val(Sgnl)"=w1795) -> ()  [unwired: 2 in, 2 out]
                            n882 = property on="V1 (N.O.)" class="Bool (strict)"("Val(Sgnl)"=TRUE ("V1 (N.O.)")) -> ()  [unwired: 2 in, 2 out]
                            n883 = property on="state 2" class="Bool (strict)"("Val(Sgnl)"=w1797) -> ()  [unwired: 2 in, 2 out]
                            n884 = Not(x=w1795) -> (.not. x?=w1796:bool)
                            n885 = Not(x=w1797) -> (.not. x?=w1798:bool)
                            n886 = property on="state 1 (false)" class="Bool (strict)"("Val(Sgnl)"=w1796) -> ()  [unwired: 2 in, 2 out]
                            n887 = property on="state 2 (false)" class="Bool (strict)"("Val(Sgnl)"=w1798) -> ()  [unwired: 2 in, 2 out]
                          }
                        }
                      }
                    }
                  }
                  frame #1 {
                    n888 = property on="V2 (N.C.)" class="Bool (strict)"() -> ("Value"=w1808:bool)  [unwired: 2 in, 2 out]
                    n889 = property on="V1 (N.O.)" class="Bool (strict)"() -> ("Value"=w1819:bool)  [unwired: 2 in, 2 out]
                    n890 = local read "P_1_high (Pa)"() -> (w1813:dbl)
                    n891 = local read "P_2_high (Pa)"() -> (w1811:dbl)
                    n892 = local read "P_1_low (Pa)"() -> (w1814:dbl)
                    n893 = local read "P_2_low (Pa)"() -> (w1812:dbl)
                    n894 = local read "L_high (%)"() -> (w1809:dbl)
                    n895 = local read "L_low (%)"() -> (w1810:dbl)
                    n896 = local read "Pav (Pa)"() -> (w1802:dbl)
                    n897 = local read "Lav (%)"() -> (w1801:dbl)
                    n898 = Boolean To (0,1)(Boolean=w1808) -> (0, 1=w1807:i16)
                    n899 = Boolean To (0,1)(Boolean=w1819) -> (0, 1=w1820:i16)
                    n900 = local read "File Refn DewarCTRL"() -> (w1815:refnum<file>)
                    n901 = local read "Cycle #"() -> (w1818:u32)
                    n902 = Build Array(w1802, w1801, w1814, w1813, w1812, w1811, w1810, w1809, w1820, w1807) -> (w1806:dbl[])
                    n903 = Get Date/Time In Seconds() -> (seconds since 1Jan1904=w1816:timestamp)
                    n904 = call "FileWrite.vi"("DataArray"=w1806, "Time Stamp"=w1816, "Error In"=errorcluster {"status"=FALSE, "code"=0, "source"=""}, "FileFormat"=string[] ["%4.5e", "%4.2f", "%4.4e", "%4.4e", "%4.4e", "%4.4e", "%4.4e", "%d", "%d"] ("Array"), "Index"=w1818, "refnum in"=w1815) -> ("Error Out"=→"Error Out (Dewar CTRL":errorcluster, "Byte Stream File Refnum"=w1805:refnum<file>)  [unwired: 4 in]
                    n905 = local write "File Refn DewarCTRL"(w1805) -> ()
                  }
                }
              }
            }
          }
          frame True {
            w1866 = "_"
            w1829 = FALSE ("auto cleanup")
            w1831 = 1 items=["one channel for each line", "one channel for all lines"] ("line grouping")
            n906 = flat-sequence {
              frame #0 {
                w1883 = FALSE ("V1 (N.O.)")
                n907 = local write "V1 (N.O.)"(TRUE ("V1 (N.O.)")) -> ()
                n908 = local write "V2 (N.C.)"(FALSE ("V1 (N.O.)")) -> ()
                n909 = local write "state 2"(w1883) -> ()
                n910 = local write "state 1"(w1883) -> ()
                n911 = local write "Fill state"(w1883) -> ()
                n912 = Not(x=w1883) -> (.not. x?=w1885:bool)
                n913 = Not(x=w1883) -> (.not. x?=w1884:bool)
                n914 = local write "state 1 (false)"(w1884) -> ()
                n915 = local write "state 2 (false)"(w1884) -> ()
                n916 = local write "Fill (false)"(w1885) -> ()
              }
            }
            n917 = Get Date/Time In Seconds() -> (seconds since 1Jan1904=w1880:timestamp)
            n918 = call "LV_UNIXTIME.vi"("current time"=w1880) -> ("date/time string"=w1861:string)  [unwired: 9 in, 1 out]
            n919 = local read "RUN Identifier"() -> (w1828:string)
            n920 = Concatenate Strings(w1861, "_DO" ("new task name")) -> (w1877:string)
            n921 = Concatenate Strings(w1828, w1866, w1861, w1866) -> (w1847:string)
            n922 = Concatenate Strings(w1847, "DEWAR.csv" ("string")) -> (w1846:string)
            n923 = Concatenate Strings(w1847, "USB_DOUT.csv" ("string")) -> (w1850:string)
            n924 = Build Path(base path=w1848, name or relative path=w1846) -> (appended path=w1845:path)
            n925 = Build Path(base path=w1848, name or relative path=w1850) -> (appended path=w1865:path)
            n926 = Open/Create/Replace File(file path (use dialog)=w1865, error in=w1856, operation (0:open)=T25."open or create") -> (refnum out=w1863:refnum<file>, error out=w1855:errorcluster)  [unwired: 3 in, 1 out]
            n927 = call "FileIntialize.vi"("Error In"=w1855, "Labels"="DOUT Labels", "refnum in"=w1863) -> ("Error Out"=w1842:errorcluster, "File Refnum"=→"File Refn USB DO":refnum<file>)  [unwired: 7 in]
            n928 = Open/Create/Replace File(file path (use dialog)=w1845, error in=w1842, operation (0:open)=T25."open or create") -> (refnum out=w1853:refnum<file>, error out=w1854:errorcluster)  [unwired: 3 in, 1 out]
            n929 = call "FileIntialize.vi"("Error In"=w1854, "Labels"=string[] ["P_av", "L_av", "P_1_low", "P_1_high", "P_2_low", "P_2_high", "L_low", "L_high", "V1(NO)", "V2(NC)"], "refnum in"=w1853) -> ("Error Out"=w1841:errorcluster, "File Refnum"=→"File Refn DewarCTRL":refnum<file>)  [unwired: 7 in]
            n930 = Index Array(array="DOUT Physical CH", index #1=0 ("index"), index #2=1 ("index"), index #3=2 ("index"), index #4=3 ("index")) -> (element #1=w1859:tag, element #2=w1837:tag, element #3=w1836:tag, element #4=w1830:tag)
            n931 = call <vilib>:"DAQmx Create Task.vi"("new task name"=w1877, "auto cleanup"=FALSE, "error in"=w1841) -> ("task out"=w1878:refnum<k21>, "error out"=w1879:errorcluster)  [unwired: 11 in]
            n932 = call-poly <vilib>:"DAQmx Create Virtual Channel.vi"("task in"=w1878, "lines"=w1859, "line grouping"=w1831, "error in"=w1879) -> ("task out"=w1881:refnum<k21>, "error out"=w1882:errorcluster)  [unwired: 10 in]
            n933 = call-poly <vilib>:"DAQmx Create Virtual Channel.vi"("task in"=w1881, "lines"=w1837, "line grouping"=w1831, "error in"=w1882) -> ("task out"=w1868:refnum<k21>, "error out"=w1867:errorcluster)  [unwired: 10 in]
            n934 = call-poly <vilib>:"DAQmx Create Virtual Channel.vi"("task in"=w1868, "lines"=w1836, "line grouping"=w1831, "error in"=w1867) -> ("task out"=w1835:refnum<k21>, "error out"=w1834:errorcluster)  [unwired: 10 in]
            n935 = call-poly <vilib>:"DAQmx Create Virtual Channel.vi"("task in"=w1835, "lines"=w1830, "line grouping"=w1831, "error in"=w1834) -> ("task out"=w1832:refnum<k21>, "error out"=w1833:errorcluster)  [unwired: 10 in]
            n936 = call <vilib>:"DAQmx Start Task.vi"("task/channels in"=w1832, "error in"=w1833) -> ("task out"=w1872:refnum<k21>, "error out"=w1870:errorcluster)  [unwired: 12 in]
            n937 = Build Array(w1829, w1829, w1829, w1829) -> (w1873:bool[])
            n938 = call <vilib>:"DAQmx Write (Digital 1D Bool NChan 1Samp 1Line).vi"("task/channels in"=w1872, "data"=w1873, "timeout"=10.0, "error in"=w1870) -> ("task out"=→"DOUT task out":refnum<k21>, "error out"=w1869:errorcluster)  [unwired: 9 in, 1 out]
          }
        }
      }
    }
    "error out (USB6210/6218 DOUT)" <- w897
    n939 = Build Array (concatenate)(w862, w863) -> (w860:dbl[])
    n940 = Build Array (concatenate)(w865, w864) -> (w861:string[])
    n941 = flat-sequence {
      tunnel: w944 -> [w1533]
      tunnel: [w1528] -> w932
      tunnel: [w1526] -> w930
      tunnel: [w1525] -> w927
      tunnel: [w1524] -> w925
      tunnel: w896 -> [w1519]
      frame #0 {
        w1527 = T26 [] ("appended array")
        n942 = Unbundle By Name(w1519) -> ("TimeArray"=w1536:timestamp[], "DataArrayConv"=w1531:dbl[][], "LDArray"=w1530:dbl[])
        n943 = Unbundle By Name(w1533) -> ("ReadLeakDet?"=w1532:bool, "LabelLD"=w1535:string, "Labels"=w1529:string[])  [unwired: 1 out]
        n944 = case shown="True" w1532 {
          tunnel: w1535 -> [_ w1544]
          tunnel: w1531 -> [w1538 w1543]
          tunnel: w1530 -> [_ w1542]
          tunnel: [w1538 w1541] -> w1518
          tunnel: w1529 -> [w1537 w1540]
          tunnel: [w1537 w1539] -> w1521
          frame False {
          }
          frame True {
            n945 = Build Array (concatenate)(w1543, w1542) -> (w1541:dbl[][])
            n946 = Build Array (concatenate)(w1540, w1544) -> (w1539:string[])
          }
        }
        "All Labels (USB6210)" <- w1521
        "DataArrayConv (USB6210)" <- w1518
        n947 = control-ref of="Plot selecter (USB6210)\n    1      2     3     4"() -> (w1520:refnum<vi>)
        n948 = local read "Plot selecter (USB6210)\n    1      2     3     4"() -> (w1523:bool[][])
        n949 = Array Size(array=w1521) -> (size(s)=w1534:i32)
        n950 = Array Size(array=w1521) -> (size(s)=w1522:i32)
        n951 = Array Size(array=w1518) -> (size(s)=→"Data Array sizes (6210)":i32[])
        n952 = property on="Property Node" class="Arr (strict)"(reference=w1520, "Number of Rows"=w1522) -> ()  [unwired: 1 in, 2 out]
        n953 = for {
          N: w1534 -> [_]
          tunnel: w1518 -> [w1565]
          tunnel: w1536 -> [w1566]
          shift-right: [w1561] -> w1526
          shift-left: w1527 -> [w1564]
          shift-right: [w1559] -> w1524
          shift-left: w1527 -> [w1562]
          shift-right: [w1560] -> w1528
          shift-left: w1527 -> [w1558]
          shift-right: [w1557] -> w1525
          shift-left: w1527 -> [w1556]
          tunnel: w1523 -> [w1555]
          i -> [w1550]
          n954 = Index Array(array=w1565, index (col)=w1550) -> (element=w1545:dbl[])  [unwired: 1 in]
          n955 = Index Array(array=w1555, index (row) #1=w1550, index (col) #1=0 ("index (row)"), index (row) #2=w1550, index (col) #2=1 ("index (row)"), index (row) #3=w1550, index (col) #3=2 ("index (row)"), index (row) #4=w1550, index (col) #4=3 ("index (row)")) -> (element #1=w1549:bool, element #2=w1548:bool, element #3=w1547:bool, element #4=w1546:bool)
          n956 = Bundle("TimeArray"=w1566, "DataArrayConv"=w1545) -> (w1563:T32)  [unwired: 1 in]
          n957 = stacked-sequence {
            tunnel: w1549 -> [w1570 _ _ _]
            tunnel: w1564 -> [_ w1578 _ _]
            tunnel: w1547 -> [_ _ w1586 _]
            tunnel: w1563 -> [w1567 w1576 w1585 w1591]
            tunnel: w1546 -> [_ _ _ w1594]
            tunnel: w1562 -> [_ _ _ w1593]
            tunnel: [_ _ _ w1592] -> w1559
            tunnel: [_ w1577 _ _] -> w1561
            tunnel: [w1569 _ _ _] -> w1560
            tunnel: w1558 -> [w1568 _ _ _]
            tunnel: [_ _ w1584 _] -> w1557
            tunnel: w1556 -> [_ _ w1583 _]
            tunnel: w1548 -> [_ w1575 _ _]
            frame #0 {
              n958 = case shown="True" w1570 {
                tunnel: [w1571 w1574] -> w1569
                tunnel: w1567 -> [_ w1573]
                tunnel: w1568 -> [w1571 w1572]
                frame False {
                }
                frame True {
                  n959 = Build Array (concatenate)(w1572, w1573) -> (w1574:T26)
                }
              }
            }
            frame #1 {
              n960 = case shown="True" w1575 {
                tunnel: w1578 -> [w1579 w1582]
                tunnel: [w1579 w1581] -> w1577
                tunnel: w1576 -> [_ w1580]
                frame False {
                }
                frame True {
                  n961 = Build Array (concatenate)(w1582, w1580) -> (w1581:T26)
                }
              }
            }
            frame #2 {
              n962 = case shown="True" w1586 {
                tunnel: [w1587 w1590] -> w1584
                tunnel: w1585 -> [_ w1589]
                tunnel: w1583 -> [w1587 w1588]
                frame False {
                }
                frame True {
                  n963 = Build Array (concatenate)(w1588, w1589) -> (w1590:T26)
                }
              }
            }
            frame #3 {
              n964 = case shown="True" w1594 {
                tunnel: [w1595 w1598] -> w1592
                tunnel: w1591 -> [_ w1597]
                tunnel: w1593 -> [w1595 w1596]
                frame False {
                }
                frame True {
                  n965 = Build Array (concatenate)(w1596, w1597) -> (w1598:T26)
                }
              }
            }
          }
        }
      }
    }
    n966 = local read "Plot selecter LSI218(2)\n    1      2     3     4"() -> (w919:bool[][])
    n967 = local read "Plot selecter LSI218(1)\n    1      2     3     4"() -> (w920:bool[][])
    n968 = for {
      N: 48 -> [_]
      tunnel: w935 -> [w1987]
      tunnel: w934 -> [w1984]
      tunnel: w920 -> [w1968]
      tunnel: w919 -> [w1969]
      shift-right: [w1985] -> w933
      shift-left: w931 -> [w1986]
      shift-right: [w1980] -> w928
      shift-left: w931 -> [w1981]
      shift-right: [w1979] -> w926
      shift-left: w931 -> [w1978]
      shift-right: [w1977] -> w924
      shift-left: w931 -> [w1976]
      i -> [w1974]
      n969 = Index Array(array=w1984, index (col)=w1974) -> (element=w1983:dbl[])  [unwired: 1 in]
      n970 = Less?(x=w1974, y=24) -> (x < y?=w1975:bool)
      n971 = case shown="True" w1975 {
        tunnel: [w1992 w2010] -> w1973
        tunnel: [w1991 w2009] -> w1972
        tunnel: [w1990 w2007] -> w1971
        tunnel: [w1989 w2006] -> w1970
        tunnel: w1968 -> [_ w2005]
        tunnel: w1969 -> [w1999 _]
        tunnel: w1974 -> [w1994 w2002]
        frame False {
          n972 = Subtract(x=w1994, y=24) -> (x-y=w1998:i32)
          n973 = Index Array(array=w1999, index (row) #1=w1998, index (col) #1=0 ("index (row)"), index (row) #2=w1998, index (col) #2=1 ("index (row)"), index (row) #3=w1998, index (col) #3=2 ("index (row)"), index (row) #4=w1998, index (col) #4=3 ("index (row)")) -> (element #1=w1992:bool, element #2=w1991:bool, element #3=w1990:bool, element #4=w1989:bool)
        }
        frame True {
          n974 = Index Array(array=w2005, index (row) #1=w2002, index (col) #1=0 ("index (row)"), index (row) #2=w2002, index (col) #2=1 ("index (row)"), index (row) #3=w2002, index (col) #3=2 ("index (row)"), index (row) #4=w2002, index (col) #4=3 ("index (row)")) -> (element #1=w2010:bool, element #2=w2009:bool, element #3=w2007:bool, element #4=w2006:bool)
        }
      }
      n975 = Bundle("TimeArray"=w1987, "DataArray"=w1983) -> (w1982:T36)  [unwired: 1 in]
      n976 = stacked-sequence {
        tunnel: w1986 -> [w2014 _ _ _]
        tunnel: [w2013 _ _ _] -> w1985
        tunnel: w1982 -> [w2012 w2022 w2030 w2038]
        tunnel: w1981 -> [_ w2021 _ _]
        tunnel: [_ w2020 _ _] -> w1980
        tunnel: [_ _ w2029 _] -> w1979
        tunnel: w1978 -> [_ _ w2028 _]
        tunnel: [_ _ _ w2037] -> w1977
        tunnel: w1976 -> [_ _ _ w2036]
        tunnel: w1973 -> [w2011 _ _ _]
        tunnel: w1972 -> [_ w2019 _ _]
        tunnel: w1971 -> [_ _ w2027 _]
        tunnel: w1970 -> [_ _ _ w2035]
        frame #0 {
          n977 = case shown="False" w2011 {
            tunnel: w2012 -> [_ w2016]
            tunnel: w2014 -> [w2015 w2018]
            tunnel: [w2015 w2017] -> w2013
            frame False {
            }
            frame True {
              n978 = Build Array (concatenate)(w2018, w2016) -> (w2017:T4)
            }
          }
        }
        frame #1 {
          n979 = case shown="True" w2019 {
            tunnel: [w2023 w2026] -> w2020
            tunnel: w2022 -> [_ w2025]
            tunnel: w2021 -> [w2023 w2024]
            frame False {
            }
            frame True {
              n980 = Build Array (concatenate)(w2024, w2025) -> (w2026:T4)
            }
          }
        }
        frame #2 {
          n981 = case shown="True" w2027 {
            tunnel: [w2031 w2034] -> w2029
            tunnel: w2030 -> [_ w2033]
            tunnel: w2028 -> [w2031 w2032]
            frame False {
            }
            frame True {
              n982 = Build Array (concatenate)(w2032, w2033) -> (w2034:T4)
            }
          }
        }
        frame #3 {
          n983 = case shown="True" w2035 {
            tunnel: [w2039 w2042] -> w2037
            tunnel: w2038 -> [_ w2041]
            tunnel: w2036 -> [w2039 w2040]
            frame False {
            }
            frame True {
              n984 = Build Array (concatenate)(w2040, w2041) -> (w2042:T4)
            }
          }
        }
      }
    }
    n985 = local read "Labels LSI336"() -> (w907:string[])
    n986 = Array Size(array=w907) -> (size(s)=w906:i32)
    n987 = local read "Plot selecter LSI336 \n     1      2     3     4"() -> (w915:bool[][])
    n988 = for {
      N: w906 -> [_]
      tunnel: w915 -> [w1900]
      shift-right: [w1894] -> w913
      shift-left: w914 -> [w1909]
      shift-right: [w1890] -> w912
      shift-left: w914 -> [w1907]
      shift-right: [w1891] -> w911
      shift-left: w914 -> [w1906]
      shift-right: [w1889] -> w910
      shift-left: w914 -> [w1905]
      tunnel: w876 -> [w1897]
      tunnel: w878 -> [w1895]
      i -> [w1898]
      n989 = Index Array(array=w1897, index (col)=w1898) -> (element=w1896:dbl[])  [unwired: 1 in]
      n990 = Index Array(array=w1900, index (row) #1=w1898, index (col) #1=0 ("index (row)"), index (row) #2=w1898, index (col) #2=1 ("index (row)"), index (row) #3=w1898, index (col) #3=2 ("index (row)"), index (row) #4=w1898, index (col) #4=3 ("index (row)")) -> (element #1=w1899:bool, element #2=w1893:bool, element #3=w1892:bool, element #4=w1888:bool)
      n991 = Bundle("TimeArray"=w1895, "DataArray"=w1896) -> (w1908:T36)  [unwired: 1 in]
      n992 = stacked-sequence {
        tunnel: w1909 -> [w1913 _ _ _]
        tunnel: [w1912 _ _ _] -> w1894
        tunnel: w1908 -> [w1911 w1921 w1929 w1937]
        tunnel: w1907 -> [_ w1920 _ _]
        tunnel: [_ w1919 _ _] -> w1890
        tunnel: [_ _ w1928 _] -> w1891
        tunnel: w1906 -> [_ _ w1927 _]
        tunnel: [_ _ _ w1936] -> w1889
        tunnel: w1905 -> [_ _ _ w1935]
        tunnel: w1899 -> [w1910 _ _ _]
        tunnel: w1893 -> [_ w1918 _ _]
        tunnel: w1892 -> [_ _ w1926 _]
        tunnel: w1888 -> [_ _ _ w1934]
        frame #0 {
          n993 = case shown="False" w1910 {
            tunnel: w1911 -> [_ w1915]
            tunnel: w1913 -> [w1914 w1917]
            tunnel: [w1914 w1916] -> w1912
            frame False {
            }
            frame True {
              n994 = Build Array (concatenate)(w1917, w1915) -> (w1916:T4)
            }
          }
        }
        frame #1 {
          n995 = case shown="True" w1918 {
            tunnel: [w1922 w1925] -> w1919
            tunnel: w1921 -> [_ w1923]
            tunnel: w1920 -> [w1922 w1924]
            frame False {
            }
            frame True {
              n996 = Build Array (concatenate)(w1924, w1923) -> (w1925:T4)
            }
          }
        }
        frame #2 {
          n997 = case shown="True" w1926 {
            tunnel: [w1930 w1933] -> w1928
            tunnel: w1929 -> [_ w1931]
            tunnel: w1927 -> [w1930 w1932]
            frame False {
            }
            frame True {
              n998 = Build Array (concatenate)(w1932, w1931) -> (w1933:T4)
            }
          }
        }
        frame #3 {
          n999 = case shown="True" w1934 {
            tunnel: [w1938 w1941] -> w1936
            tunnel: w1937 -> [_ w1939]
            tunnel: w1935 -> [w1938 w1940]
            frame False {
            }
            frame True {
              n1000 = Build Array (concatenate)(w1940, w1939) -> (w1941:T4)
            }
          }
        }
      }
    }
    n1001 = Array Size(array=w878) -> (size(s)=→"TimeArray Size (336)":i32)
    n1002 = Array Size(array=w876) -> (size(s)=→"DataArray size (336)":i32[])
    n1003 = Build Array (concatenate)(w932, w933, w913, w891, w836) -> (→"Graph 1":T26)
    n1004 = Build Array (concatenate)(w930, w928, w912, w890, w835) -> (→"Graph 2":T26)
    n1005 = Build Array (concatenate)(w927, w926, w911, w889, w834) -> (→"Graph 3":T26)
    n1006 = Build Array (concatenate)(w925, w924, w910, w888, w833) -> (→"Graph 4":T26)
    n1007 = Send Notification(notification="Stop Button", notifier=w853, error in (no error)=w852) -> (notifier out=w849:refnum<notifier>, error out=w850:errorcluster)
    "Cycle #" <- w842
  }
  n1008 = while {
    tunnel: w5 -> [w2131]
    tunnel: w4 -> [w2130]
    stop <- w2132 stop-if-true
    n1009 = flat-sequence {
      frame #0 {
        n1010 = Divide(x="V_sample", y="I_sample") -> (x/y=w2138:dbl)
        "R_sample" <- w2138
        n1011 = Multiply(x="I_sample", y="V_sample") -> (x*y=→"Q_sample":dbl)
        n1012 = Divide(x="Q_input", y=w2138) -> (x/y=w2137:dbl)
        n1013 = Square Root(x=w2137) -> (sqrt(x)=→"V_input":dbl)
      }
    }
    n1014 = Wait (ms)(milliseconds to wait=u32 214) -> ()  [unwired: 1 out]
    n1015 = case shown="True" "RECORD GRAPH" {
      frame False {
      }
      frame True {
        n1016 = stacked-sequence {
          frame #0 {
            n1017 = Get Date/Time In Seconds() -> (seconds since 1Jan1904=w2176:timestamp)
            n1018 = local read "Base Path"() -> (w2161:path)
            n1019 = local read "RUN Identifier"() -> (w2177:string)
            n1020 = call "LV_UNIXTIME.vi"("current time"=w2176) -> ("date/time string"=w2178:string)  [unwired: 9 in, 1 out]
            n1021 = control-ref of="Graph CHF"() -> (w2167:refnum<vi>)
            n1022 = Concatenate Strings(w2177, "_CHF" ("string"), w2178, "_" ("string"), "CHF Graph Comment") -> (w2163:string)
            n1023 = Concatenate Strings(w2163, ".png" ("string")) -> (w2162:string)
            n1024 = Concatenate Strings(w2163, ".csv" ("string")) -> (w2165:string)
            "CHF file name" <- w2165
            n1025 = Build Path(base path=w2161, name or relative path=w2165) -> (appended path=w2172:path)
            n1026 = invoke class="XYGraph (strict)" method="Get Image"(reference=w2167) -> ("image data"=w2159:T24)  [unwired: 5 in, 5 out]
            n1027 = local read "ƒ¢T_array"() -> (w2169:dbl[])
            n1028 = local read "Q_array"() -> (w2168:dbl[])
            n1029 = Build Path(base path=w2161, name or relative path=w2162) -> (appended path=w2160:path)
            n1030 = Open/Create/Replace File(file path (use dialog)=w2172, operation (0:open)=T25."open or create") -> (refnum out=w2170:refnum<file>)  [unwired: 4 in, 2 out]
            n1031 = for {
              tunnel: w2170 -> [w2182]
              tunnel: w2169 -> [w2180] mode=indexing
              tunnel: w2168 -> [w2179] mode=indexing
              n1032 = Format Into String(format string="%4.4e,%4.4e\\n" ("prompt"), initial string=w2182, w2180, w2179) -> ()  [unwired: 1 in, 2 out]
            }
            n1033 = call <vilib>:"Write PNG File.vi"("image data"=w2159, "path to PNG file"=w2160) -> ()  [unwired: 8 in, 2 out]
          }
          frame #1 {
            n1034 = local write "RECORD GRAPH"(FALSE ("RECORD GRAPH")) -> ()
          }
        }
      }
    }
    n1035 = case shown="True" "START CHF" {
      tunnel: "RecordSettings" -> [_ w2187]
      frame False {
      }
      frame True {
        n1036 = stacked-sequence {
          tunnel: [w2191 _ _] -> _
          tunnel: w2187 -> [w2190 w2264 _]
          frame #0 {
            (unwired) T25."open or create" ("operation (0:open)")
            n1037 = Get Date/Time In Seconds() -> (seconds since 1Jan1904=w2203:timestamp)
            n1038 = for {
              tunnel: [w2251] -> w2189 mode=indexing
              tunnel: w2190 -> [w2250] mode=indexing
              n1039 = Unbundle By Name(w2250) -> ("SourceLabel"=w2251:string)
            }
            "CHF Data Labels" <- w2189
            n1040 = local read "Base Path"() -> (w2198:path)
            n1041 = local read "RUN Identifier"() -> (w2202:string)
            n1042 = call "LV_UNIXTIME.vi"("current time"=w2203) -> ("date/time string"=w2201:string)  [unwired: 9 in, 1 out]
            n1043 = Concatenate Strings(w2202, "_" ("string"), w2201, "_CHFlog.csv" ("string")) -> (w2197:string)
            "CHF log file name" <- w2197
            n1044 = Build Path(base path=w2198, name or relative path=w2197) -> (appended path=w2196:path)
            n1045 = Open/Create/Replace File(file path (use dialog)=w2196, error in=errorcluster {"status"=FALSE, "code"=0, "source"=""}, operation (0:open)=T25."open or create", access (0:read/write)=enum16{"read/write", "read-only", "write-only"}."read/write") -> (refnum out=w2194:refnum<file>, error out=w2193:errorcluster)  [unwired: 2 in, 1 out]
            n1046 = call "FileIntialize.vi"("Error In"=w2193, "Labels"=w2189, "refnum in"=w2194) -> ("File Refnum"=w2191:refnum<file>)  [unwired: 7 in, 1 out]
            "File Refnum (CHF)" <- w2191
            n1047 = local write "CHF measurement counter"(0 ("CHF counter")) -> ()
            n1048 = property on="Kenwood set V (V)" class="DigNum (strict)"("Val(Sgnl)"="V start (V)") -> ()  [unwired: 2 in, 2 out]
            n1049 = stacked-sequence {
              tunnel: w2189 -> [w2207 w2230]
              frame #0 {
                n1050 = Array Size(array=w2207) -> (size(s)=w2215:i32)
                n1051 = control-ref of="Graph CHF log 1"() -> (w2208:refnum<vi>)
                n1052 = property class="XYGraph (strict)"(reference=w2208, error in=errorcluster {"status"=FALSE, "code"=0, "source"=""} ("error in (no error)")) -> (reference out=w2210:refnum<vi>, error out=w2212:errorcluster, "LegNumRows"=w2213:u32)
                n1053 = for {
                  N: w2213 -> [_]
                  shift-right: [w2224] -> w2214
                  shift-left: w2212 -> [w2225]
                  tunnel: w2210 -> [w2223]
                  tunnel: [w2222] -> w2209 mode=indexing
                  i -> [w2227]
                  n1054 = property class="XYGraph (strict)"(reference=w2223, error in=w2225, "Active Plot"=w2227, "Plot.Plot Name"="") -> (reference out=w2222:refnum<vi>, error out=w2224:errorcluster)
                }
                n1055 = for {
                  N: w2215 -> [_]
                  shift-right: [w2219] -> w2206
                  shift-left: w2214 -> [w2220]
                  tunnel: w2209 -> [w2217] mode=indexing
                  tunnel: w2207 -> [w2216] mode=indexing
                  i -> [w2221]
                  n1056 = property class="XYGraph (strict)"(reference=w2217, error in=w2220, "Active Plot"=w2221, "Plot.Plot Name"=w2216, "Plot.Visible?"=TRUE ("Plot.Visible")) -> (error out=w2219:errorcluster)  [unwired: 1 out]
                }
                n1057 = local write "Error out (CHF rec)"(w2206) -> ()
              }
              frame #1 {
                n1058 = Array Size(array=w2230) -> (size(s)=w2237:i32)
                n1059 = control-ref of="Graph CHF log 2"() -> (w2229:refnum<vi>)
                n1060 = property class="XYGraph (strict)"(reference=w2229, error in=errorcluster {"status"=FALSE, "code"=0, "source"=""} ("error in (no error)")) -> (reference out=w2232:refnum<vi>, error out=w2234:errorcluster, "LegNumRows"=w2235:u32)
                n1061 = for {
                  N: w2235 -> [_]
                  shift-right: [w2246] -> w2236
                  shift-left: w2234 -> [w2247]
                  tunnel: w2232 -> [w2245]
                  tunnel: [w2244] -> w2231 mode=indexing
                  i -> [w2249]
                  n1062 = property class="XYGraph (strict)"(reference=w2245, error in=w2247, "Active Plot"=w2249, "Plot.Plot Name"="") -> (reference out=w2244:refnum<vi>, error out=w2246:errorcluster)
                }
                n1063 = for {
                  N: w2237 -> [_]
                  shift-right: [w2241] -> w2228
                  shift-left: w2236 -> [w2242]
                  tunnel: w2231 -> [w2239] mode=indexing
                  tunnel: w2230 -> [w2238] mode=indexing
                  i -> [w2243]
                  n1064 = property class="XYGraph (strict)"(reference=w2239, error in=w2242, "Active Plot"=w2243, "Plot.Plot Name"=w2238, "Plot.Visible?"=TRUE ("Plot.Visible")) -> (error out=w2241:errorcluster)  [unwired: 1 out]
                }
                n1065 = local write "Error out (CHF rec)"(w2228) -> ()
              }
            }
          }
          frame #1 {
            n1066 = local read "V start (V)"() -> (w2263:dbl)
            n1067 = Absolute Value(x="V_end (V)") -> (abs(x)=w2260:dbl)
            n1068 = Absolute Value(x=w2263) -> (abs(x)=w2261:dbl)
            n1069 = Build Array(w2261, w2260) -> (w2259:dbl[])
            n1070 = Array Max & Min(array=w2259) -> (max value=w2258:dbl, min value=w2257:dbl)  [unwired: 2 out]
            n1071 = Subtract(x=w2258, y=w2257) -> (x-y=w2256:dbl)
            n1072 = Quotient & Remainder(x=w2256, y="ƒ¢V / cycle (V)") -> (floor(x/y)=w2254:dbl)  [unwired: 1 out]
            n1073 = for {
              N: w2254 -> [_]
              tunnel: w2264 -> [w2272]
              shift-right: [w2268] -> _
              shift-left: dbl[][] [] -> [w2270]
              shift-right: [w2267] -> _
              shift-left: timestamp[] [] -> [w2269]
              tunnel: "ƒ¢V / cycle (V)" -> [w2266]
              i -> [w2271]
              n1074 = case shown="False" "STOP CHF" {
                tunnel: w2272 -> [w2288 _]
                tunnel: w2271 -> [w2287 _]
                tunnel: w2270 -> [w2286 w2513]
                tunnel: w2269 -> [w2282 w2512]
                tunnel: [w2279 w2513] -> w2268
                tunnel: [w2278 w2512] -> w2267
                tunnel: w2266 -> [w2273 _]
                frame False {
                  n1075 = stacked-sequence {
                    tunnel: w2288 -> [_ _ w2320]
                    tunnel: [_ _ w2311] -> w2277
                    tunnel: w2287 -> [_ _ w2310]
                    tunnel: w2287 -> [w2295 _ _]
                    tunnel: [_ _ w2308] -> w2276
                    tunnel: [_ _ w2307] -> w2281
                    tunnel: [_ _ w2306] -> w2285
                    tunnel: w2286 -> [_ _ w2306]
                    tunnel: [_ _ w2305] -> w2284
                    tunnel: w2282 -> [_ _ w2304]
                    tunnel: [_ _ w2304] -> w2283
                    tunnel: w2273 -> [w2294 _ _]
                    frame #0 {
                      n1076 = property on="CHF measurement counter" class="DigNum (strict)"("Val(Sgnl)"=w2295) -> ()  [unwired: 2 in, 2 out]
                      n1077 = property on="Kenwood set V (V)" class="DigNum (strict)"() -> ("Value"=w2297:dbl)  [unwired: 2 in, 2 out]
                      n1078 = Add(x=w2297, y=w2294) -> (x+y=w2296:dbl)
                      n1079 = property on="Kenwood set V (V)" class="DigNum (strict)"("Val(Sgnl)"=w2296) -> ()  [unwired: 2 in, 2 out]
                    }
                    frame #1 {
                      n1080 = Multiply(x="CHF cycle interval (s) (>1s)", y=1000.0) -> (x*y=w2299:dbl)
                      n1081 = Wait (ms)(milliseconds to wait=w2299) -> ()  [unwired: 1 out]
                    }
                    frame #2 {
                      n1082 = for {
                        tunnel: w2320 -> [w2477] mode=indexing
                        tunnel: [w2475] -> w2307 mode=indexing
                        tunnel: [w2473] -> w2318 mode=indexing
                        n1083 = Unbundle By Name(w2477) -> ("Source"=w2476:T37, "SourceLabel"=w2474:string, "FileFormat"=w2473:string)
                        n1084 = case shown="\"LSI218\"" w2476 {
                          tunnel: [w2478 w2483 w2488 w2494 w2502 w2507] -> w2475
                          tunnel: w2474 -> [w2479 w2485 w2490 w2493 w2503 w2511]
                          frame "USB6210", Default {
                            n1085 = local read "All Labels (USB6210)"() -> (w2481:string[])
                            n1086 = local read "Last Data \n(USB6210)"() -> (w2482:dbl[])
                            n1087 = Search 1D Array(1D array=w2481, element=w2479) -> (index of element=w2480:i32)  [unwired: 1 in]
                            n1088 = Index Array(array=w2482, index=w2480) -> (element=w2478:dbl)
                          }
                          frame "USB6218AI" {
                            n1089 = local read "All Labels (USB6218)"() -> (w2486:string[])
                            n1090 = local read "Last Data \n(USB6218)"() -> (w2487:dbl[])
                            n1091 = Search 1D Array(1D array=w2486, element=w2485) -> (index of element=w2484:i32)  [unwired: 1 in]
                            n1092 = Index Array(array=w2487, index=w2484) -> (element=w2483:dbl)
                          }
                          frame "USB6218AO" {
                            n1093 = local read "USB 6218 AOUT"() -> (w2492:dbl[])
                            n1094 = local read "AOUT Labels"() -> (w2491:string[])
                            n1095 = Search 1D Array(1D array=w2491, element=w2490) -> (index of element=w2489:i32)  [unwired: 1 in]
                            n1096 = Index Array(array=w2492, index=w2489) -> (element=w2488:dbl)
                          }
                          frame "LSI218" {
                            n1097 = local read "Labels LSI218 (1)"() -> (w2497:string[])
                            n1098 = local read "Labels LSI218 (2)"() -> (w2496:string[])
                            n1099 = local read "Last Data \nLSI218 (1)"() -> (w2500:dbl[])
                            n1100 = local read "Last Data \nLSI218 (2)"() -> (w2499:dbl[])
                            n1101 = Build Array (concatenate)(w2497, w2496) -> (w2495:string[])
                            n1102 = Build Array (concatenate)(w2500, w2499) -> (w2498:dbl[])
                            n1103 = Search 1D Array(1D array=w2495, element=w2493) -> (index of element=w2501:i32)  [unwired: 1 in]
                            n1104 = Index Array(array=w2498, index=w2501) -> (element=w2494:dbl)
                          }
                          frame "LSI336" {
                            n1105 = local read "Last Data \nLSI336"() -> (w2505:dbl[])
                            n1106 = local read "Labels LSI336"() -> (w2506:string[])
                            n1107 = Search 1D Array(1D array=w2506, element=w2503) -> (index of element=w2504:i32)  [unwired: 1 in]
                            n1108 = Index Array(array=w2505, index=w2504) -> (element=w2502:dbl)
                          }
                          frame "DMMs" {
                            n1109 = local read "DMM LastMeasurements"() -> (w2508:dbl[])
                            n1110 = local read "DMMsLabels"() -> (w2510:string[])
                            n1111 = Search 1D Array(1D array=w2510, element=w2511) -> (index of element=w2509:i32)  [unwired: 1 in]
                            n1112 = Index Array(array=w2508, index=w2509) -> (element=w2507:dbl)
                          }
                        }
                      }
                      "CHF last data" <- w2307
                      n1113 = stacked-sequence {
                        tunnel: [w2321 _ _ _] -> w2316
                        tunnel: [_ w2359 _ _] -> w2315
                        tunnel: [_ _ _ w2435] -> w2314
                        tunnel: [_ _ w2397 _] -> w2313
                        frame #0 {
                          n1114 = Unbundle By Name("Data I") -> ("Source"=w2323:T37, "SourceLabel"=w2322:string)
                          n1115 = case shown="\"DMMs\"" w2323 {
                            tunnel: w2322 -> [w2326 w2331 w2336 w2341 w2350 w2355]
                            tunnel: [w2325 w2330 w2335 w2340 w2349 w2354] -> w2321
                            frame "USB6210", Default {
                              n1116 = local read "All Labels (USB6210)"() -> (w2328:string[])
                              n1117 = local read "Last Data \n(USB6210)"() -> (w2327:dbl[])
                              n1118 = Search 1D Array(1D array=w2328, element=w2326) -> (index of element=w2329:i32)  [unwired: 1 in]
                              n1119 = Index Array(array=w2327, index=w2329) -> (element=w2325:dbl)
                            }
                            frame "USB6218AI" {
                              n1120 = local read "All Labels (USB6218)"() -> (w2333:string[])
                              n1121 = local read "Last Data \n(USB6218)"() -> (w2332:dbl[])
                              n1122 = Search 1D Array(1D array=w2333, element=w2331) -> (index of element=w2334:i32)  [unwired: 1 in]
                              n1123 = Index Array(array=w2332, index=w2334) -> (element=w2330:dbl)
                            }
                            frame "USB6218AO" {
                              n1124 = local read "USB 6218 AOUT"() -> (w2337:dbl[])
                              n1125 = local read "AOUT Labels"() -> (w2338:string[])
                              n1126 = Search 1D Array(1D array=w2338, element=w2336) -> (index of element=w2339:i32)  [unwired: 1 in]
                              n1127 = Index Array(array=w2337, index=w2339) -> (element=w2335:dbl)
                            }
                            frame "LSI218" {
                              n1128 = local read "Labels LSI218 (1)"() -> (w2346:string[])
                              n1129 = local read "Labels LSI218 (2)"() -> (w2347:string[])
                              n1130 = local read "Last Data \nLSI218 (1)"() -> (w2343:dbl[])
                              n1131 = local read "Last Data \nLSI218 (2)"() -> (w2344:dbl[])
                              n1132 = Build Array (concatenate)(w2346, w2347) -> (w2348:string[])
                              n1133 = Build Array (concatenate)(w2343, w2344) -> (w2345:dbl[])
                              n1134 = Search 1D Array(1D array=w2348, element=w2341) -> (index of element=w2342:i32)  [unwired: 1 in]
                              n1135 = Index Array(array=w2345, index=w2342) -> (element=w2340:dbl)
                            }
                            frame "LSI336" {
                              n1136 = local read "Last Data \nLSI336"() -> (w2352:dbl[])
                              n1137 = local read "Labels LSI336"() -> (w2351:string[])
                              n1138 = Search 1D Array(1D array=w2351, element=w2350) -> (index of element=w2353:i32)  [unwired: 1 in]
                              n1139 = Index Array(array=w2352, index=w2353) -> (element=w2349:dbl)
                            }
                            frame "DMMs" {
                              n1140 = local read "DMM LastMeasurements"() -> (w2358:dbl[])
                              n1141 = local read "DMMsLabels"() -> (w2356:string[])
                              n1142 = Search 1D Array(1D array=w2356, element=w2355) -> (index of element=w2357:i32)  [unwired: 1 in]
                              n1143 = Index Array(array=w2358, index=w2357) -> (element=w2354:dbl)
                            }
                          }
                          "I" <- w2321
                        }
                        frame #1 {
                          n1144 = Unbundle By Name("Data V") -> ("Source"=w2362:T37, "SourceLabel"=w2361:string)
                          n1145 = case shown="\"LSI218\"" w2362 {
                            tunnel: w2361 -> [w2364 w2369 w2374 w2379 w2388 w2393]
                            tunnel: [w2363 w2368 w2373 w2378 w2387 w2392] -> w2359
                            frame "USB6210", Default {
                              n1146 = local read "All Labels (USB6210)"() -> (w2366:string[])
                              n1147 = local read "Last Data \n(USB6210)"() -> (w2365:dbl[])
                              n1148 = Search 1D Array(1D array=w2366, element=w2364) -> (index of element=w2367:i32)  [unwired: 1 in]
                              n1149 = Index Array(array=w2365, index=w2367) -> (element=w2363:dbl)
                            }
                            frame "USB6218AI" {
                              n1150 = local read "All Labels (USB6218)"() -> (w2371:string[])
                              n1151 = local read "Last Data \n(USB6218)"() -> (w2370:dbl[])
                              n1152 = Search 1D Array(1D array=w2371, element=w2369) -> (index of element=w2372:i32)  [unwired: 1 in]
                              n1153 = Index Array(array=w2370, index=w2372) -> (element=w2368:dbl)
                            }
                            frame "USB6218AO" {
                              n1154 = local read "USB 6218 AOUT"() -> (w2375:dbl[])
                              n1155 = local read "AOUT Labels"() -> (w2376:string[])
                              n1156 = Search 1D Array(1D array=w2376, element=w2374) -> (index of element=w2377:i32)  [unwired: 1 in]
                              n1157 = Index Array(array=w2375, index=w2377) -> (element=w2373:dbl)
                            }
                            frame "LSI218" {
                              n1158 = local read "Labels LSI218 (1)"() -> (w2384:string[])
                              n1159 = local read "Labels LSI218 (2)"() -> (w2385:string[])
                              n1160 = local read "Last Data \nLSI218 (1)"() -> (w2381:dbl[])
                              n1161 = local read "Last Data \nLSI218 (2)"() -> (w2382:dbl[])
                              n1162 = Build Array (concatenate)(w2384, w2385) -> (w2386:string[])
                              n1163 = Build Array (concatenate)(w2381, w2382) -> (w2383:dbl[])
                              n1164 = Search 1D Array(1D array=w2386, element=w2379) -> (index of element=w2380:i32)  [unwired: 1 in]
                              n1165 = Index Array(array=w2383, index=w2380) -> (element=w2378:dbl)
                            }
                            frame "LSI336" {
                              n1166 = local read "Last Data \nLSI336"() -> (w2390:dbl[])
                              n1167 = local read "Labels LSI336"() -> (w2389:string[])
                              n1168 = Search 1D Array(1D array=w2389, element=w2388) -> (index of element=w2391:i32)  [unwired: 1 in]
                              n1169 = Index Array(array=w2390, index=w2391) -> (element=w2387:dbl)
                            }
                            frame "DMMs" {
                              n1170 = local read "DMM LastMeasurements"() -> (w2396:dbl[])
                              n1171 = local read "DMMsLabels"() -> (w2394:string[])
                              n1172 = Search 1D Array(1D array=w2394, element=w2393) -> (index of element=w2395:i32)  [unwired: 1 in]
                              n1173 = Index Array(array=w2396, index=w2395) -> (element=w2392:dbl)
                            }
                          }
                          "V" <- w2359
                        }
                        frame #2 {
                          n1174 = Unbundle By Name("Data T_low") -> ("Source"=w2400:T37, "SourceLabel"=w2399:string)
                          n1175 = case shown="\"DMMs\"" w2400 {
                            tunnel: w2399 -> [w2402 w2407 w2412 w2417 w2426 w2431]
                            tunnel: [w2401 w2406 w2411 w2416 w2425 w2430] -> w2397
                            frame "USB6210", Default {
                              n1176 = local read "All Labels (USB6210)"() -> (w2404:string[])
                              n1177 = local read "Last Data \n(USB6210)"() -> (w2403:dbl[])
                              n1178 = Search 1D Array(1D array=w2404, element=w2402) -> (index of element=w2405:i32)  [unwired: 1 in]
                              n1179 = Index Array(array=w2403, index=w2405) -> (element=w2401:dbl)
                            }
                            frame "USB6218AI" {
                              n1180 = local read "All Labels (USB6218)"() -> (w2409:string[])
                              n1181 = local read "Last Data \n(USB6218)"() -> (w2408:dbl[])
                              n1182 = Search 1D Array(1D array=w2409, element=w2407) -> (index of element=w2410:i32)  [unwired: 1 in]
                              n1183 = Index Array(array=w2408, index=w2410) -> (element=w2406:dbl)
                            }
                            frame "USB6218AO" {
                              n1184 = local read "USB 6218 AOUT"() -> (w2413:dbl[])
                              n1185 = local read "AOUT Labels"() -> (w2414:string[])
                              n1186 = Search 1D Array(1D array=w2414, element=w2412) -> (index of element=w2415:i32)  [unwired: 1 in]
                              n1187 = Index Array(array=w2413, index=w2415) -> (element=w2411:dbl)
                            }
                            frame "LSI218" {
                              n1188 = local read "Labels LSI218 (1)"() -> (w2422:string[])
                              n1189 = local read "Labels LSI218 (2)"() -> (w2423:string[])
                              n1190 = local read "Last Data \nLSI218 (1)"() -> (w2419:dbl[])
                              n1191 = local read "Last Data \nLSI218 (2)"() -> (w2420:dbl[])
                              n1192 = Build Array (concatenate)(w2422, w2423) -> (w2424:string[])
                              n1193 = Build Array (concatenate)(w2419, w2420) -> (w2421:dbl[])
                              n1194 = Search 1D Array(1D array=w2424, element=w2417) -> (index of element=w2418:i32)  [unwired: 1 in]
                              n1195 = Index Array(array=w2421, index=w2418) -> (element=w2416:dbl)
                            }
                            frame "LSI336" {
                              n1196 = local read "Last Data \nLSI336"() -> (w2428:dbl[])
                              n1197 = local read "Labels LSI336"() -> (w2427:string[])
                              n1198 = Search 1D Array(1D array=w2427, element=w2426) -> (index of element=w2429:i32)  [unwired: 1 in]
                              n1199 = Index Array(array=w2428, index=w2429) -> (element=w2425:dbl)
                            }
                            frame "DMMs" {
                              n1200 = local read "DMM LastMeasurements"() -> (w2434:dbl[])
                              n1201 = local read "DMMsLabels"() -> (w2432:string[])
                              n1202 = Search 1D Array(1D array=w2432, element=w2431) -> (index of element=w2433:i32)  [unwired: 1 in]
                              n1203 = Index Array(array=w2434, index=w2433) -> (element=w2430:dbl)
                            }
                          }
                          "T_low" <- w2397
                        }
                        frame #3 {
                          n1204 = Unbundle By Name("Data T_high") -> ("Source"=w2438:T37, "SourceLabel"=w2437:string)
                          n1205 = case shown="\"DMMs\"" w2438 {
                            tunnel: w2437 -> [w2440 w2445 w2450 w2455 w2464 w2469]
                            tunnel: [w2439 w2444 w2449 w2454 w2463 w2468] -> w2435
                            frame "USB6210", Default {
                              n1206 = local read "All Labels (USB6210)"() -> (w2442:string[])
                              n1207 = local read "Last Data \n(USB6210)"() -> (w2441:dbl[])
                              n1208 = Search 1D Array(1D array=w2442, element=w2440) -> (index of element=w2443:i32)  [unwired: 1 in]
                              n1209 = Index Array(array=w2441, index=w2443) -> (element=w2439:dbl)
                            }
                            frame "USB6218AI" {
                              n1210 = local read "All Labels (USB6218)"() -> (w2447:string[])
                              n1211 = local read "Last Data \n(USB6218)"() -> (w2446:dbl[])
                              n1212 = Search 1D Array(1D array=w2447, element=w2445) -> (index of element=w2448:i32)  [unwired: 1 in]
                              n1213 = Index Array(array=w2446, index=w2448) -> (element=w2444:dbl)
                            }
                            frame "USB6218AO" {
                              n1214 = local read "USB 6218 AOUT"() -> (w2451:dbl[])
                              n1215 = local read "AOUT Labels"() -> (w2452:string[])
                              n1216 = Search 1D Array(1D array=w2452, element=w2450) -> (index of element=w2453:i32)  [unwired: 1 in]
                              n1217 = Index Array(array=w2451, index=w2453) -> (element=w2449:dbl)
                            }
                            frame "LSI218" {
                              n1218 = local read "Labels LSI218 (1)"() -> (w2460:string[])
                              n1219 = local read "Labels LSI218 (2)"() -> (w2461:string[])
                              n1220 = local read "Last Data \nLSI218 (1)"() -> (w2457:dbl[])
                              n1221 = local read "Last Data \nLSI218 (2)"() -> (w2458:dbl[])
                              n1222 = Build Array (concatenate)(w2460, w2461) -> (w2462:string[])
                              n1223 = Build Array (concatenate)(w2457, w2458) -> (w2459:dbl[])
                              n1224 = Search 1D Array(1D array=w2462, element=w2455) -> (index of element=w2456:i32)  [unwired: 1 in]
                              n1225 = Index Array(array=w2459, index=w2456) -> (element=w2454:dbl)
                            }
                            frame "LSI336" {
                              n1226 = local read "Last Data \nLSI336"() -> (w2466:dbl[])
                              n1227 = local read "Labels LSI336"() -> (w2465:string[])
                              n1228 = Search 1D Array(1D array=w2465, element=w2464) -> (index of element=w2467:i32)  [unwired: 1 in]
                              n1229 = Index Array(array=w2466, index=w2467) -> (element=w2463:dbl)
                            }
                            frame "DMMs" {
                              n1230 = local read "DMM LastMeasurements"() -> (w2472:dbl[])
                              n1231 = local read "DMMsLabels"() -> (w2470:string[])
                              n1232 = Search 1D Array(1D array=w2470, element=w2469) -> (index of element=w2471:i32)  [unwired: 1 in]
                              n1233 = Index Array(array=w2472, index=w2471) -> (element=w2468:dbl)
                            }
                          }
                          "T_high" <- w2435
                        }
                      }
                      n1234 = local read "File Refnum (CHF)"() -> (w2301:refnum<file>)
                      n1235 = Get Date/Time In Seconds() -> (seconds since 1Jan1904=w2305:timestamp)
                      n1236 = Subtract(x=w2314, y=w2313) -> (x-y=w2309:dbl)
                      "ƒ¢T" <- w2309
                      n1237 = Multiply(x=w2316, y=w2315) -> (x*y=w2312:dbl)
                      "Q" <- w2312
                      n1238 = local read "ƒ¢T_array"() -> (w2303:dbl[])
                      n1239 = local read "Q_array"() -> (w2302:dbl[])
                      n1240 = call "FileWrite.vi"("DataArray"=w2307, "Time Stamp"=w2305, "Error In"=errorcluster {"status"=FALSE, "code"=0, "source"=""}, "FileFormat"=w2318, "Index"=w2310, "refnum in"=w2301) -> ("Error Out"=→"Error out (CHF rec)":errorcluster)  [unwired: 4 in, 1 out]
                      n1241 = Build Array (concatenate)(w2303, w2309) -> (w2308:dbl[])
                      n1242 = Build Array (concatenate)(w2302, w2312) -> (w2311:dbl[])
                    }
                  }
                  n1243 = Build Array (concatenate)(w2285, w2281) -> (w2279:dbl[][])
                  n1244 = Build Array (concatenate)(w2283, w2284) -> (w2278:timestamp[])
                  n1245 = Bundle(w2276, w2277) -> (→"Graph CHF":cluster{dbl[], dbl[]})  [unwired: 1 in]
                  n1246 = local write "ƒ¢T_array"(w2276) -> ()
                  n1247 = local write "Q_array"(w2277) -> ()
                  n1248 = Array Size(array=w2281) -> (size(s)=w2280:i32)
                  n1249 = for {
                    N: w2280 -> [_]
                    tunnel: w2279 -> [w2293]
                    tunnel: w2278 -> [w2291]
                    tunnel: [w2289] -> w2274 mode=indexing
                    i -> [w2292]
                    n1250 = Index Array(array=w2293, index (col)=w2292) -> (element=w2290:dbl[])  [unwired: 1 in]
                    n1251 = Bundle(w2291, w2290) -> (w2289:cluster{timestamp[], dbl[]})  [unwired: 1 in]
                  }
                  "Graph CHF log 2" <- w2274
                  "Graph CHF log 1" <- w2274
                  "Graph CHF log 3" <- w2274
                }
                frame True {
                }
              }
            }
          }
          frame #2 {
            n1252 = local write "CHF measurement counter"(0 ("CHF counter")) -> ()
            n1253 = local write "START CHF"(FALSE ("START CHF")) -> ()
            n1254 = local write "STOP CHF"(FALSE ("STOP CHF")) -> ()
          }
        }
      }
    }
    n1255 = case shown="True" "START heater cycle" {
      frame False {
      }
      frame True {
        n1256 = while {
          i -> [w2145]
          stop <- w2143 stop-if-true
          n1257 = flat-sequence {
            frame #0 {
              n1258 = property on="OUTPUT \nKenwood" class="Bool (strict)"("Val(Sgnl)"=TRUE ("Value (Signaling)")) -> ()  [unwired: 2 in, 2 out]
              n1259 = property on="Kenwood set V (V)" class="DigNum (strict)"("Val(Sgnl)"="V_peak") -> ()  [unwired: 2 in, 2 out]
            }
            frame #1 {
              n1260 = Multiply(x="t_on", y=1000.0) -> (x*y=w2151:dbl)
              n1261 = Wait (ms)(milliseconds to wait=w2151) -> ()  [unwired: 1 out]
            }
            frame #2 {
              n1262 = property on="OUTPUT \nKenwood" class="Bool (strict)"("Val(Sgnl)"=FALSE ("Value (Signaling)")) -> ()  [unwired: 2 in, 2 out]
              n1263 = property on="Kenwood set V (V)" class="DigNum (strict)"("Val(Sgnl)"=0.0 ("Value (Signaling)")) -> ()  [unwired: 2 in, 2 out]
            }
            frame #3 {
              n1264 = Multiply(x="t_off", y=1000.0) -> (x*y=w2158:dbl)
              n1265 = Wait (ms)(milliseconds to wait=w2158) -> ()  [unwired: 1 out]
            }
          }
          n1266 = case shown="False" "STOP heater cycle" {
            tunnel: [FALSE TRUE] -> w2143
            frame False {
            }
            frame True {
              n1267 = property on="START heater cycle" class="Bool (strict)"("Val(Sgnl)"=FALSE ("Value (Signaling)")) -> ()  [unwired: 2 in, 2 out]
            }
          }
          "Heat Cycle counter" <- w2145
        }
      }
    }
    n1268 = case shown="True" "REFRESH GRAPH" {
      frame False {
      }
      frame True {
        n1269 = stacked-sequence {
          frame #0 {
            w2185 = dbl[] [] ("ƒ¢T_array")
            n1270 = local write "ƒ¢T_array"(w2185) -> ()
            n1271 = local write "Q_array"(w2185) -> ()
            n1272 = Bundle("ƒ¢T_array"=w2185, "ƒ¢T_array"=w2185) -> (w2184:cluster{"ƒ¢T_array":dbl[], "ƒ¢T_array":dbl[]})  [unwired: 1 in]
            n1273 = local write "Graph CHF"(w2184) -> ()
          }
          frame #1 {
            n1274 = local write "REFRESH GRAPH"(FALSE ("REFRESH GRAPH")) -> ()
          }
        }
      }
    }
    n1275 = Get Notifier Status(notifier=w2131, error in (no error)=w2130) -> (current notification=w2132:bool)  [unwired: 4 out]
  }
  n1276 = while {
    shift-right: [w2526] -> w8
    shift-left: refnum<class "DMMsData.lvclass"> refnum ("DMMsData.lvclass") -> [w2525]
    shift-right: [w2524] -> w7
    shift-left: errorcluster {"status"=FALSE, "code"=0, "source"=""} ("error in (no error)") -> [w2517]
    tunnel: w5 -> [w2522]
    tunnel: w4 -> [w2521]
    tunnel: [w2520] -> w11
    i -> [w2523]
    stop <- w2519 stop-if-true
    n1277 = Equal?(x=w2523, y=0) -> (x = y?=w2527:bool)
    n1278 = Wait (ms)(milliseconds to wait="Measurement Interval DMMs (ms)") -> ()  [unwired: 1 out]
    n1279 = case shown="True" "Measure DMMs?" {
      tunnel: w2527 -> [_ w2538]
      tunnel: [w2531 w2536] -> w2526
      tunnel: w2525 -> [w2531 w2535]
      tunnel: w2517 -> [w2530 w2534]
      tunnel: [w2530 w2533] -> w2524
      tunnel: w2523 -> [_ w2532]
      frame False {
      }
      frame True {
        n1280 = Or(x="Initialize (DMMs)", y=w2538) -> (x .or. y?=w2537:bool)
        n1281 = case shown="False" w2537 {
          tunnel: w2535 -> [w2569 w2605]
          tunnel: [w2566 w2604] -> w2536
          tunnel: w2534 -> [w2568 w2601]
          tunnel: [w2567 w2598] -> w2533
          tunnel: w2532 -> [w2565 _]
          frame False {
            n1282 = local read "VariableSources"() -> (w2558:T12)
            n1283 = for {
              tunnel: w2558 -> [w2572] mode=indexing
              tunnel: [w2571] -> w2557 mode=indexing
              tunnel: [w2570] -> w2556 mode=indexing
              n1284 = case shown="\"LSI218\"" w2572 {
                tunnel: [w2574 w2576 w2578 w2579 w2585] -> w2571
                tunnel: [w2573 w2575 w2577 w2580 w2586] -> w2570
                frame "USB6210" {
                  n1285 = local read "All Labels (USB6210)"() -> (w2574:string[])
                  n1286 = local read "Last Data \n(USB6210)"() -> (w2573:dbl[])
                }
                frame "USB6218AI" {
                  n1287 = local read "Last Data \n(USB6218)"() -> (w2575:dbl[])
                  n1288 = local read "All Labels (USB6218)"() -> (w2576:string[])
                }
                frame "USB6218AO" {
                  n1289 = local read "USB 6218 AOUT"() -> (w2577:dbl[])
                  n1290 = local read "AOUT Labels"() -> (w2578:string[])
                }
                frame "LSI218" {
                  n1291 = local read "Last Data \nLSI218 (2)"() -> (w2581:dbl[])
                  n1292 = local read "Last Data \nLSI218 (1)"() -> (w2582:dbl[])
                  n1293 = local read "Labels LSI218 (2)"() -> (w2584:string[])
                  n1294 = local read "Labels LSI218 (1)"() -> (w2583:string[])
                  n1295 = Build Array (concatenate)(w2582, w2581) -> (w2580:dbl[])
                  n1296 = Build Array (concatenate)(w2583, w2584) -> (w2579:string[])
                }
                frame "LSI336" {
                  n1297 = local read "Last Data \nLSI336"() -> (w2586:dbl[])
                  n1298 = local read "Labels LSI336"() -> (w2585:string[])
                }
              }
            }
            n1299 = local read "DMMsConfig (variables)"() -> (w2550:T13)
            n1300 = local read "DMMsConfig"() -> (w2562:T11)
            n1301 = call-dynamic "DMMs_measure.vi"("DMMsData in"=w2569, "Sample #"="Sample #", "MeasurementIndex"=w2565, "SourceDataLabels"=w2557, "error in (no error)"=w2568, "SourceDataArray"=w2556) -> ("TimeArray"=w2564:timestamp[], "DMMsData out"=w2566:refnum<class "DMMsData.lvclass">, "LastData"=w2544:dbl[], "DataArray"=w2561:dbl[][], "DeviceActive?"=→"Active?":bool[], "error out"=w2567:errorcluster)  [unwired: 4 in]
            "DMM LastMeasurements" <- w2544
            n1302 = Array Size(array=w2550) -> (size(s)=w2548:i32)
            n1303 = Array Size(array=w2562) -> (size(s)=w2549:i32)
            n1304 = Add(x=w2549, y=w2548) -> (x+y=w2547:i32)
            n1305 = for {
              N: w2547 -> [_]
              tunnel: w2564 -> [w2589]
              tunnel: w2561 -> [w2593]
              shift-right: [w2587] -> w2546
              shift-left: T4 [] -> [w2588]
              i -> [w2592]
              n1306 = Index Array(array=w2593, index (col)=w2592) -> (element=w2591:dbl[])  [unwired: 1 in]
              n1307 = Bundle("TimeArray"=w2589, "DataArray"=w2591) -> (w2590:T36)  [unwired: 1 in]
              n1308 = Build Array (concatenate)(w2588, w2590) -> (w2587:T4)
            }
            "Graph DMMs 2" <- w2546
            "Graph DMMs 1" <- w2546
            "Graph DMMs 3" <- w2546
            n1309 = Index Array(array=w2544, index #1="index T_2", index #2="index T_ 1") -> (element #1=w2543:dbl, element #2=w2540:dbl)
            n1310 = Index Array(array=w2544, index #1="index V", index #2="index I") -> (element #1=w2553:dbl, element #2=w2552:dbl)
            n1311 = Subtract(x=w2543, y=w2540) -> (x-y=→"ƒ¢T=T_2 -T_1":dbl)
            n1312 = Multiply(x=w2553, y=w2552) -> (x*y=→"Q = I *V":dbl)
          }
          frame True {
            n1313 = local write "Initialize (DMMs)"(FALSE ("Initialize 2")) -> ()
            n1314 = local read "RUN Identifier"() -> (w2597:string)
            n1315 = local read "Base Path"() -> (w2602:path)
            n1316 = call-dynamic "DMMs_initialize.vi"("DMMsConfig (variables)"="DMMsConfig (variables)", "DMMsConfig"="DMMsConfig", "InstName"="InstName DMMs", "error in (no error)"=w2601, "base path"=w2602, "RunIdentifier"=w2597, "DMMsData in"=w2605) -> ("error out"=w2598:errorcluster, "DMMsLabels"=w2599:string[], "FileName"=→"DMMFileName":string, "DMMsData out"=w2604:refnum<class "DMMsData.lvclass">, "VariableSources"=→"VariableSources":T12)
            "DMMsLabels" <- w2599
            n1317 = stacked-sequence {
              tunnel: w2599 -> [w2607 w2630 w2653]
              frame #0 {
                n1318 = Array Size(array=w2607) -> (size(s)=w2616:i32)
                n1319 = control-ref of="Graph DMMs 1"() -> (w2613:refnum<vi>)
                n1320 = property class="XYGraph (strict)"(reference=w2613, error in=errorcluster {"status"=FALSE, "code"=0, "source"=""} ("error in (no error)")) -> (reference out=w2609:refnum<vi>, error out=w2612:errorcluster, "LegNumRows"=w2614:u32)
                n1321 = for {
                  N: w2614 -> [_]
                  shift-right: [w2625] -> w2615
                  shift-left: w2612 -> [w2626]
                  tunnel: w2609 -> [w2624]
                  tunnel: [w2623] -> w2608 mode=indexing
                  i -> [w2628]
                  n1322 = property class="XYGraph (strict)"(reference=w2624, error in=w2626, "Active Plot"=w2628, "Plot.Plot Name"="") -> (reference out=w2623:refnum<vi>, error out=w2625:errorcluster)
                }
                n1323 = for {
                  N: w2616 -> [_]
                  shift-right: [w2620] -> w2610
                  shift-left: w2615 -> [w2621]
                  tunnel: w2608 -> [w2618] mode=indexing
                  tunnel: w2607 -> [w2617] mode=indexing
                  i -> [w2622]
                  n1324 = property class="XYGraph (strict)"(reference=w2618, error in=w2621, "Active Plot"=w2622, "Plot.Plot Name"=w2617, "Plot.Visible?"=TRUE ("Plot.Visible")) -> (error out=w2620:errorcluster)  [unwired: 1 out]
                }
                "error out (DMM graphs)" <- w2610
              }
              frame #1 {
                n1325 = Array Size(array=w2630) -> (size(s)=w2638:i32)
                n1326 = control-ref of="Graph DMMs 2"() -> (w2633:refnum<vi>)
                n1327 = property class="XYGraph (strict)"(reference=w2633, error in=errorcluster {"status"=FALSE, "code"=0, "source"=""} ("error in (no error)")) -> (reference out=w2632:refnum<vi>, error out=w2635:errorcluster, "LegNumRows"=w2636:u32)
                n1328 = for {
                  N: w2636 -> [_]
                  shift-right: [w2647] -> w2637
                  shift-left: w2635 -> [w2648]
                  tunnel: w2632 -> [w2646]
                  tunnel: [w2645] -> w2631 mode=indexing
                  i -> [w2650]
                  n1329 = property class="XYGraph (strict)"(reference=w2646, error in=w2648, "Active Plot"=w2650, "Plot.Plot Name"="") -> (reference out=w2645:refnum<vi>, error out=w2647:errorcluster)
                }
                n1330 = for {
                  N: w2638 -> [_]
                  shift-right: [w2642] -> w2629
                  shift-left: w2637 -> [w2643]
                  tunnel: w2631 -> [w2640] mode=indexing
                  tunnel: w2630 -> [w2639] mode=indexing
                  i -> [w2644]
                  n1331 = property class="XYGraph (strict)"(reference=w2640, error in=w2643, "Active Plot"=w2644, "Plot.Plot Name"=w2639, "Plot.Visible?"=TRUE ("Plot.Visible")) -> (error out=w2642:errorcluster)  [unwired: 1 out]
                }
                n1332 = local write "error out (DMM graphs)"(w2629) -> ()
              }
              frame #2 {
                n1333 = Array Size(array=w2653) -> (size(s)=w2660:i32)
                n1334 = control-ref of="Graph DMMs 3"() -> (w2651:refnum<vi>)
                n1335 = property class="XYGraph (strict)"(reference=w2651, error in=errorcluster {"status"=FALSE, "code"=0, "source"=""} ("error in (no error)")) -> (reference out=w2655:refnum<vi>, error out=w2657:errorcluster, "LegNumRows"=w2658:u32)
                n1336 = for {
                  N: w2658 -> [_]
                  shift-right: [w2669] -> w2659
                  shift-left: w2657 -> [w2670]
                  tunnel: w2655 -> [w2668]
                  tunnel: [w2667] -> w2654 mode=indexing
                  i -> [w2672]
                  n1337 = property class="XYGraph (strict)"(reference=w2668, error in=w2670, "Active Plot"=w2672, "Plot.Plot Name"="") -> (reference out=w2667:refnum<vi>, error out=w2669:errorcluster)
                }
                n1338 = for {
                  N: w2660 -> [_]
                  shift-right: [w2664] -> w2652
                  shift-left: w2659 -> [w2665]
                  tunnel: w2654 -> [w2662] mode=indexing
                  tunnel: w2653 -> [w2661] mode=indexing
                  i -> [w2666]
                  n1339 = property class="XYGraph (strict)"(reference=w2662, error in=w2665, "Active Plot"=w2666, "Plot.Plot Name"=w2661, "Plot.Visible?"=TRUE ("Plot.Visible")) -> (error out=w2664:errorcluster)  [unwired: 1 out]
                }
                n1340 = local write "error out (DMM graphs)"(w2652) -> ()
              }
            }
          }
        }
        "error out (DMMs)" <- w2533
      }
    }
    n1341 = Get Notifier Status(notifier=w2522, error in (no error)=w2521) -> (current notification=w2519:bool, error out=w2520:errorcluster)  [unwired: 3 out]
    "cycle # (DMMs)" <- w2523
  }
  n1342 = call-dynamic "USBData_terminate.vi"("error in (no error)"=w24, "USBData in"=w25) -> ("error out"=w26:errorcluster)  [unwired: 8 in, 1 out]
  n1343 = local write "error out (USB6210)"(w26) -> ()
  n1344 = call-dynamic "DMMs_terminate.vi"("error in (no error)"=w7, "DMMsData in"=w8) -> ("error out"=→"error out (DMMs) 2":errorcluster)  [unwired: 8 in, 1 out]
  n1345 = call-dynamic "USBData_terminate.vi"("error in (no error)"=w39, "USBData in"=w40) -> ("error out"=w41:errorcluster)  [unwired: 8 in, 1 out]
  n1346 = call-dynamic "LSI336Data_terminate.vi"("error in (no error)"=w30, "LSI336Data in"=w31) -> ("error out"=w29:errorcluster)  [unwired: 8 in, 1 out]
  n1347 = Merge Errors(w11, w13) -> (w14:errorcluster)
  n1348 = local write "error out (USB6210)"(w41) -> ()
  n1349 = local write "error out (LSI336)"(w29) -> ()
  n1350 = call "LSI218Data_terminate.vi"("error in (no error)"=w34, "LSI218Data in"=w35) -> ("error out"=w33:errorcluster)  [unwired: 8 in, 1 out]
  n1351 = Release Notifier(notifier=w12, error in (no error)=w14) -> (error out=→"error out (notifier)":errorcluster)  [unwired: 1 in, 2 out]
  n1352 = local write "error out (LSI218)"(w33) -> ()
